vi "AlliGator Settings Window.vi"() -> ()   [LabVIEW 2021, in "AlliGator Settings.lvlib"]
doc: "GUI providing access to settings parameters for all aspect of AlliGator's functions."
uses:
  AlliGator Settings.lvlib
  Phasor Plot/AlliGator Phasor Plot Size.ctl
  AlliGator Background Subtraction Parameters.ctl
  Graphs/XY Graph/XY Graph Plot Shift Parameters.ctl
  Graphs/XY Graph/XY Graph Plot Shift Method.ctl
  Image/Image Save File Format.ctl
  AlliGator Low Count Pixels Rejection Options.ctl
  Phasor/Phasor Ratio Type.ctl
  Decay Analysis/Decay Preprocessing/AlliGator Baseline Subtraction Method.ctl
  Fits/IRF(X)PSED/Decay Fit Options v4.ctl
  Fits/Decay Convolution/Decay Model.ctl
  Fits/Residual Type.ctl
  Fits/IRF(X)PSED/Fit Weights Type v2.ctl
  Fits/Non-linear Fitting Method v2.ctl
  Fits/Fit Calculation Method.ctl
  Fits/Non-linear Fitting Algorithm.ctl
  Fits/IRF(X)PSED/Decay Fit Parameters & Derived Quantities List v2.ctl
  Decay Analysis/Decay Fit/AlliGator Decay Fit Parameter Constraints 2.ctl
  Fits/IRF(X)PSED/Decay Fit Parameters In List.ctl
  Decay Analysis/IRF/AlliGator IRF Optimization Controls.ctl
  Decay Analysis/IRF/AlliGator IRF Deconvolution Metrics.ctl
  Math/Advanced Signal Processing Toolkit/Wavelet Analysis Options.ctl
  AlliGator High Count Pixels Rejection Options.ctl
  AlliGator Image Smoothing Options.ctl
  Arrays/Kernel Type.ctl
  Arrays/Smoothing Algorithm.ctl
  Fits/Square Pulse/Square Pulse Options.ctl
  Fits/Square Pulse/Square Pulse Levels Type.ctl
  Source Image/AlliGator Image Binning Options.ctl
  Phasor Plot/AlliGator Phasor Plot Smoothing Options.ctl
  AlliGator Phasor Plot Graphics Options.ctl
  AlliGator Exported Image Settings.ctl
  Fits/IRF(X)PSED/IRF(X)PSED Extraction Options.ctl
  Fits/IRF(X)PSED/Fourier Series Smoothing Option.ctl
  Fits/IRF(X)PSED/Fourier Series Truncation.ctl
  Fits/IRF(X)PSED/IRF Extraction Method.ctl
  Phasor/Phasor Explorer Display Parameters.ctl
  Phasor/Phasor Type of Series.ctl
  Phasor/Phasor Explorer Decay Parameters.ctl
  Phasor/Phasor IRF Model.ctl
  Phasor/Phasor Explorer Phasor Parameters.ctl
  Phasor/Phasor Calculation Type.ctl
  Phasor/Phasor SEPL Type.ctl
  Phasor/Phasor Explorer Gate Parameters.ctl
  Phasor/Phasor Gate Type.ctl
  Phasor/Phasor Type of User-defined Function.ctl
  Phasor/Phasor Explorer Gate Parameter to Adjust.ctl
  AlliGator Define Gates to.ctl
  AlliGator Gates to Keep.ctl
  Phasor Ratio/AlliGator Phasor Ratio Color-Coded Quantity.ctl
  Phasor/Phasor Calibration Type.ctl
  Histograms/Linear Histogram Options.ctl
  Histograms/Histogram Bin Option.ctl
  Histograms/Histogram Bin Position.ctl
  AlliGator Gate Arithmetic.ctl
  Phasor Ratio/AlliGator Phasor Reference Associated with Shortest Lifetime.ctl
  AlliGator Python Settings.ctl
  SwissSPAD/SwissSPAD Live_Image Display Options.ctl
  AlliGator Average Lifetime Options.ctl
  Phasor Calibration/AlliGator Calibration Map Algorithm.ctl
  Decay Analysis/Decay Fit/AlliGator Guess Parameters Options.ctl
  Phasor/Phasor Standard Deviation Options.ctl
  Source Image/AlliGator Source Image Scale Bar Options.ctl
  Fits/IRF(X)PSED/MLE Baseline Offset Type.ctl
  Fits/Optimal Offset Selection Criterion.ctl
  AlliGator Settings Q Element.ctl
  AlliGator Settings Q Action.ctl
  Globals, Variables, Constants/AlliGator Refnums List.ctl
  AlliGator Settings List.ctl
  Globals, Variables, Constants/AlliGator Variables List.ctl
  Image/Image Hot Pixel Map Target.ctl
  Action Engine/AlliGator Q Element.ctl
  Action Engine/AlliGator Q Event.ctl
  Palette/Image Palette Information.ctl
  Image/Image Display Palette Type.ctl
  Notebook/Notebook Parameters List.ctl
  GUI/AlliGator Skippable Windows Status.ctl
  AlliGator Quantities.ctl
  f3e5a785-d283-42c9-a630-fb32b7f70655.vi
  c46dad3f-f40e-47bf-8043-7fc63249f95d.vi
  Variant/Variant to Data/Variant to [String].vi
  Variant/Variant to Data/Variant to I32.vi
  Variant/Variant to Data/Variant to Boolean.vi
  Formula/Aliases Definition Window.vi
  Variant/Variant to Data/Variant to U16.vi
  Variant/Variant to Data/Variant to String.vi
  Variant/Variant to Data/Variant to Path.vi
  Variant/Variant to Data/Variant to U32.vi
  Action Engine/AlliGator Action Engine.lvlib
  Globals, Variables, Constants/AlliGator Globals, Variables & Constants.lvlib
  Variant/Variant to Data/Variant to Data.lvlib
  Palette/Palette.lvlib
  Image/Image.lvlib
  GUI/AlliGator GUI.lvlib
  Phasor Plot/AlliGator Phasor Plot.lvlib
  Phasor Graph/AlliGator Phasor Graph.lvlib
  Error/Error.lvlib
  Graphs/Plot Editor/Plot Editor.lvlib
  Phasor/Phasor Explorer.lvlib
  Phasor Ratio/AlliGator Phasor Ratio.lvlib
  Utilities/Utilities.lvlib
  <vilib>/vision/NI_Vision_Development_Module.lvlib
  Python Plugins API/AlliGator Python Plugins.lvlib
  Notebook/Notebook.lvlib
  SwissSPAD/SwissSPAD Live.lvlib
  Formula/Formula.lvlib
  Fits/Fits.lvlib
  Phasor/Phasor.lvlib
  Graphs/XY Graph/XY Graph Add-Ons.lvlib
  Decay Analysis/Decay Fit/AlliGator Decay Fit.lvlib
  Decay Analysis/IRF/AlliGator IRF.lvlib
  Math/Math.lvlib
  Arrays/Arrays.lvlib
  Source Image/AlliGator Source Image.lvlib
  Histograms/Histogram Window.lvlib
  Phasor Calibration/AlliGator Phasor Calibration.lvlib
  Decay Analysis/Decay Preprocessing/AlliGator Decay Preprocessing.lvlib
panel:
  in  "Settings Tabs":T1(tab)
  in  "Source Image Tabs":T2(tab)
  in  "Hot Pixel Removal":T3 caption="Hot Pixel Removal (*)" {"Percentile" min=0 max=100}
  in  "Use Image Histogram for Contrast":bool=TRUE
  in  "Low Count Pixels Rejection Options":T4={"Background Low Threshold Factor"=0.0, "Fixed Low Background Threshold"=20000.0, "Reject Low Count Pixels"=FALSE, "Low Percentile"=0.0} {"Low Percentile" min=0.0 max=100.0}
  in  "High Count Pixels Rejection Options":T5={"Background High Threshold Factor"=0.0, "Fixed High Background Threshold"=1.0, "Reject High Count Pixels"=FALSE, "High Percentile"=100.0} {"High Percentile" min=0.0 max=100.0}
  in  "ROI Creation":string="ROI Creation"
  in  "Image Pre-Processing Operations Order":u16(ring) items=["Remove Screamers", "Pile-up Correction", "Binning", "Smoothing", "Rescaling"]
  in  "Dead Left Columns Correction":bool
  in  "ROI Diameter":i32=12
  in  "Use Fixed ROI Diameter":bool
  in  "ROI Center Color":u32(colorbox)=16711680
  in  "Peak Threshold":dbl=500.0
  in  "Image Smoothing Options":T6={"Use Image Smoothing"=FALSE, "Kernel Type"=enum."Bilinear", "Bin"=1, "Algorithm"=enum."Rapid"} caption="Image Smoothing Options (*)" {"Bin" min=1}
  in  "Image Binning Options":T9={"Use Image Binning"=FALSE, "X Bin"=1, "Y Bin"=1} caption="Image Binning Options (*)" {"Y Bin" min=1; "X Bin" min=1}
  in  "Invert Binary Mask":bool
  in  "Intensity Threshold":dbl=500.0
  in  "Overlay Analyzed ROI Center":bool
  in  "Save Source Image":bool caption="Save Image"
  in  "Median Overlay Color":u32(colorbox)
  in  "Overlay ROI Median":bool=TRUE caption="Use Image Brightness"
  in  "Use Image Brightness":bool=TRUE
  in  "Blend Overlay with Image Background":bool=TRUE
  in  "Scale Bar Options":T10 caption="Scale Bar Options (*)"
  in  "Image Resolution (Pixel Size)":dbl[unit]
  in  "Dataset Scaling Factor":dbl=1.0 caption="Scaling Factor" min=0.0
  in  "Gate Image Integration":dbl[unit]=3e-10 min=0.0 format="%#.3g"
  in  "Gate Image Exposure":dbl[unit]=3e-10 min=0.0 format="%#.3g"
  in  "Available Channel Names":string[](array[string])
  in  "Background File Subtraction":bool
  in  "Background Scaling Factor":dbl=1.0 caption="Scaling Factor" min=0.0
  in  "Background File":path caption="Background Dataset"
  in  "Background Pile-up Correction":bool caption="Pile-up Correction"
  in  "Background Pixel Well Capacity":u32=1 caption="Max Value" min=1 step=1
  in  "Pixel Well Capacity":u32=1 caption="Max Value" min=1 step=1
  in  "Pile-up Correction":bool
  in  "Channel Arithmetic":T11 caption="Channel Arithmetic (*)"
  in  "Channel Name":u16(ring) items=["Gate"]
  in  "Gates to Keep":T12={"First"=0, "Last"=4294967295} caption="Gates to Keep (*)"
  in  "Define Gates to":T13 caption="Define Gates to (*)"
  in  "SYNC Period":dbl[unit] min=0.0 format="%#.3g"
  out "Natural Frequency":dbl[unit] min=0.0 format="%#.3g"
  in  "# Gates":u32=1 min=1 step=1
  in  "Gate Step":u32=1 caption="Gate Step (*)" min=1 step=1
  in  "Gate Width":dbl[unit]=3e-10 min=0.0 format="%#.3g"
  in  "Nanotime Gate Separation":dbl[unit]=4e-11 caption="Gate Separation" min=0.0 format="%#.3g"
  in  "Gates to Skip":T14 caption="Gates to Skip (*)"
  in  "Laser Period":dbl[unit] min=0.0 format="%#.3g"
  in  "Fluorescence Decay Tabs":T15(tab) caption="Fluorescence Decay Tab"
  in  "[0-1]-Normalize Decay":bool caption="1- Normalize Decay"
  in  "# Folds":u32=1 min=1
  in  "Fold Decay":bool caption="Straighten Decay"
  in  "Use Decay Pre-Processing":bool=TRUE
  in  "Head Fraction":dbl min=0.0 max=1.0 format="%.4g"
  in  "Use Cursors":bool
  in  "Use Periodicity":bool
  in  "Pixel-Normalize Decay":bool
  in  "Constant Background":dbl=1.0
  in  "Verbose Decay Pre-Processing":bool=TRUE
  in  "Decay Pre-Processing Operations Order":u16(ring) items=["Background subtraction", "Reverse", "Smoothen", "Straighten", "Shift", "Extrapolate", "Normalize", "Fold"]
  in  "Straighten Decay":bool
  in  "Background Subtraction":bool=TRUE
  in  "Baseline Subtraction Method":T16=enum."Min"
  in  "Background Definition Range":T17={"Min Gate"=0.0, "Max Gate"=8e-10} {"Max Gate" min=0.0 format="%#_5g"; "Min Gate" min=0.0 format="%#_5g"}
  in  "Additional Points":u32
  in  "Tail Fraction":dbl min=0.0 max=1.0 format="%.4g"
  in  "Extrapolate Decay":bool
  in  "Shift Decay":bool
  in  "Smoothen Decay":bool
  in  "Smoothing Parameter":dbl=-1.0 min=0.0 max=1.0
  in  "1-Normalize Decay":bool caption="1- Normalize Decay"
  in  "Decay Shift Parameters":T18
  in  "Reverse Gates":bool
  in  "Average Lifetime Options":T20={"Use Local IRF "=TRUE, "Use IRF Offset"=TRUE, "Use Fixed Offset"=TRUE, "Fixed Offset"=0.0, "Baseline %"=0.0} caption="Use Local IRF" {"Baseline %" min=0.0 max=100.0}
  in  "IRF Extraction Options":T21={"Time Constant for IRF Extraction"=1e-18, "IRF Order"=1, "Fourier Series Smoothing"=enum."None", "Noise Threshold"=0.0, "Smoothing Width"=0.0, "Fourier Series Truncation"=enum."Automatic", "Truncation Order"=0, "Save Power Spectrum"=FALSE, "Smoothing"=FALSE, "Smoothing Parameter"=0.0, "Smoothing Order"=1, "Method"=enum."Direct"} {"Smoothing Order" max=100 step=1; "Smoothing Parameter" min=-1.0 max=1.0; "Time Constant for IRF Extraction" min=0.0 format="%#_5g"}
  in  "IRF Optimization Options":T25={"Search Range"=1e-18, "Search Step"=1e-09, "Tail Threshold (%)"=1e-09, "Regularized IRF"=FALSE, "Export Plot"=FALSE, "Export Data"=FALSE, "Smooth Metrics"=FALSE, "S-G Side Points"=1, "S-G Polynomial Order"=3, "Metrics"=enum."Tail Average"} {"S-G Polynomial Order" min=3 max=10; "S-G Side Points" min=1; "Tail Threshold (%)" min=0.0 max=100.0; "Search Step" min=0.0; "Search Range" min=0.0}
  in  "Square Pulse Options":T27={"Method"=enum."Mode", "# Bins"=0, "Threshold %"=10.0, "Center on Midpoint"=FALSE, "Smoothen Plot"=FALSE} {"Threshold %" min=0.0 max=100.0}
  in  "Wavelet Analysis Options":T29={"Wavelet"=enum."db02", "Option for Approximate Coefficients"=enum."None", "# Levels"=1, "Threshold Settings"={"Thresholding Rule"=enum."Universal", "Rescaling Method"=enum."Single level", "Soft Threshold?"=TRUE}, "Wavelet Transform Type"=enum."Discrete"}
  in  "Extract IRF instead of Decay":bool
  in  "Use Data Information Laser Period":bool
  in  "Use Legacy Fitting Approach":bool
  in  "Fit Options":T30={"Show Fit Residuals"=TRUE, "Fit Model"=enum."1-Exponential", "Residual Type"=enum."Standard", "Max Decay Percentile"=1.0, "Min Decay Percentile"=0.0, "Show Full Decay"=TRUE, "Weights"=enum."1/Variance (Neyman)", "Fitting Method"=enum."Least Square", "Compute Parameter Uncertainties"=TRUE, "Periodic Boundaries"=FALSE, "Model Calculation"=enum."Simulation", "Period"=1.2500000000000001e-08, "Termination Criteria"={"Max Iterations"=1000, "Max Function Calls"=0, "Max Time"=1000.0, "Function Tolerance"=1e-06, "Parameter Tolerance"=1e-06, "Gradient Tolerance"=0.0, "Min Lambda"=1e-06, "Max Lambda"=1e-06, "Initial Tick Count"=0}, "Offset Resolution"=4e-11, "Use Local IRF"=TRUE, "Fitting Algorithm"=enum."Levenberg-Marquardt", "Show Confidence Interval "=TRUE, "Confidence Level"=95.0} {"Confidence Level" min=0.0 max=100.0; "Offset Resolution" min=0.0; "Period" min=0.0; "Min Decay Percentile" min=0.0 max=100.0; "Max Decay Percentile" min=0.0 max=100.0}
  in  "MLE Baseline Offset Type":T37
  in  "MLE Baseline Offset":dbl
  in  "Optimal Offset Selection Criterion":T38
  in  "Guess Parameters Options":T39 caption="Options"
  in  "Use Last Fitted Parameters":bool
  in  "Guess Parameter Names":T40[](array[typedef]) caption="Names"
  in  "Use Guess Parameters":bool
  in  "Guess Parameter Values":dbl[](array[numeric]) caption="Values"
  in  "Fit Parameter Constraints":T41[](array[typedef]) {"Max Value" format="%#.3g"; "Min Value" format="%#.3g"}
  in  "Displayed Fit Parameters":T42[](array[typedef])
  in  "Export Tabulated Results":bool=TRUE
  in  "Fluorescence Decay Graph Default Plot Style":cluster{"X":dbl, "Y":dbl}[](graph) caption="Phasor Graph Default Plot Style"
  in  "Decay Graph Color Array":u32[](array[colorbox])
  in  "Show Last Decay Only":bool caption="Show Last Decay only"
  in  "Max Peak Value":dbl
  in  "Reject High Decay Peak Pixels":bool
  in  "Min Peak Value":dbl
  in  "Reject Low Decay Peak Pixels":bool
  in  "Intensity Correction File":path
  in  "Use Intensity Correction File":bool
  in  "Use File Timestamp":bool
  in  "Time Step":dbl[unit]=1.0
  in  "Phasor Plot Tabs":T43(tab)
  in  "Intensity-weighted Phasor Plot":bool
  in  "Phasor Plot Smoothing Options":T44={"Use Phasor Plot Smoothing"=FALSE, "Kernel Type"=enum."Uniform", "Bin"=1, "Algorithm"=enum."Rapid"} {"Bin" min=1 step=2}
  in  "Phasor Plot Frequency":dbl[unit]=80000000.0 caption="Phasor Frequency"
  in  "Selected Image ROI(s)":bool
  in  "All Image ROIs":bool
  in  "Selected Phasor Plot ROI(s)":bool
  in  "All Phasor Plot ROIs":bool
  in  "Cumulative Phasor Plot":bool
  in  "Store Phasor Harmonics":bool
  in  "Phasor Ratio Color Scale":dbl(ramp)
  in  "Phasor Ratio Decay Range":dbl=1.0 caption="Decay Range"
  in  "Phasor Ratio Reference Colors":T45={"Reference 1"=3381759, "Reference 2"=3381759, "Boundary"=3381759} caption="Reference Colors"
  in  "Exponential Fading":bool
  in  "Phasor Ratio Color Map Type":T46(radio) caption="Color Map Type"
  out "Phasor Ratio Color Map":string caption="Average Lifetime Color Map"
  out "Ref 2 Label":string="Ref 1"
  out "Ref 1 Label":string="Ref 2"
  in  "Phasor Ratio Display Range":cluster{dbl, dbl}(slide)={0.0, 454.0} caption="Average Lifetime Display Range" scale=0.0..0.1 scale format="%#.3g"
  in  "Reference Radius":i32=512 min=1
  in  "Phasor Ratio Color-Coded Quantity":T47 caption="Displayed Quantity"
  in  "Draw Reference Segment":bool
  in  "User-Defined Quantity":string
  in  "Blend Overlay with Phasor Background":bool=TRUE
  in  "Use Phasor Brightness":bool
  in  "Phasor Plot Size":T48={"H"=512, "V"=512, "Margin"=0.2} {"Margin" min=0.0}
  in  "Phasor Plot Graphics Options":T49={"UC Color"=3381759, "Show UC Tau Ticks"=FALSE, "SEPL Color"=3381759, "Show SEPL Tau Ticks"=FALSE, "Axes Color"=16776960, "Show (g,s) Ticks"=FALSE, "Show UC"=FALSE, "Show SEPL"=FALSE, "Show Axes"=FALSE, "Show UC Tau Labels"=FALSE, "Show SEPL Tau Labels"=FALSE, "Show (g,s) Labels"=FALSE, "UC Label Size"=18, "UC Label Distance"=0.0, "SEPL Label Size"=18, "SEPL Label Distance"=0.0, "Axes Label Size"=18, "Axes Label Distance"=0.0}
  in  "Intensity-weighted Phasor Graph":bool
  in  "Define Shortest Lifetime as":T50
  in  "Save Phasor Graph Image":bool
  in  "Phasor Graph Frequency":dbl[unit]=80000000.0 caption="Phasor Frequency"
  in  "Phasor Ratio Type":T51
  in  "Pixel-level Phasor Computation":bool
  in  "Phasor SDV Options":T52={"Compute Estimated SDV"=FALSE, "# Replicas"=100, "Use Estimated Average Phasor"=FALSE}
  in  "SEPL Tabs":enum32{"Display", "Phasor", "IRF", "Gates"}(tab)
  in  "Display Parameters":T53={"# Points"=1000, "Ramp Type"=enum."Logarithmic", "Type of Series"=enum."1-Exp Decays", "Min tau"=1.0000000000000002e-12, "Max tau"=1.0000000000000001e-07, "Include 0"=FALSE, "Include Infinity"=FALSE} {"Min tau" min=0.0; "Max tau" min=0.0; "# Points" min=1 step=1}
  in  "Phasor Parameters":T55={"Harmonic Frequency"=0.0, "Use f* = 1/D Frequency"=FALSE, "Calibrated Phasor"=FALSE, "Calibration Lifetime"=1e-09, "Phasor Calculation"=enum."Direct Sum", "SEPL Type"=enum."UC", "# Gates"=1.0, "Square Gate Width"=1e-09, "Show Ticks"=FALSE} {"Square Gate Width" min=0.0; "# Gates" min=0.0; "Calibration Lifetime" min=0.0; "Harmonic Frequency" min=0.0}
  in  "Decay & IRF Parameters":T58={"Lifetime"=3.0000000000000004e-09, "IRF Offset"=0.0, "IRF Period"=1.2500000000000001e-08, "Normalized Decays"=FALSE, "IRF Model"=enum."Dirac", "IRF Parameter 1"=0.0} caption="IRF Parameters" {"Lifetime" min=0.0; "IRF Period" min=0.0}
  in  "Edit User-defined Function":bool caption="Edit User-defined Gate"
  in  "Gate Parameter to Adjust":T60 caption="Adjust"
  in  "Match Laser Period":bool=TRUE
  in  "Gate Parameters":T61={"First Gate Start"=0.0, "Use Gate Center"=FALSE, "Gate Width"=0.0, "Gate Step"=0.0, "# Gates"=1.0, "Gate Type"=enum."Square", "Edge Width"=0.0, "Top Slope"=0.0, "Reversed Sawtooth?"=FALSE, "Analytical Computation"=FALSE, "Integration"=enum."Item 0", "Tolerance"=1.0, "# Steps"=1.0, "Type of User-defined Function"=enum."Gate", "Use Gate Step"=FALSE} {"# Steps" min=0.0; "Tolerance" min=0.0; "Top Slope" min=0.0; "Edge Width" min=0.0; "Gate Step" min=0.0; "# Gates" min=1.0 step=1.0; "Gate Width" min=0.0}
  in  "Use Current Dataset Parameters":bool
  in  "Calibration Map Algorithm":T64
  in  "Calibration Type":T65=enum."Single Phasor"
  in  "Backup Calibration Type":T66(ring) caption="Backup Calibration"
  in  "Use Backup Calibration if needed":bool=TRUE
  in  "Calibration Lifetime":dbl[unit]=1e-09
  in  "Lifetime Analysis Graph Default Plot Style":cluster{"X":dbl, "Y":dbl}[](graph) caption="Phasor Graph Default Plot Style"
  in  "Decay Analysis Parameters":T18
  in  "Plugins Folder":bool
  in  "Parameter Names only":bool
  in  "Send JSON to Clipboard":bool
  in  "Reset Python Session":bool
  out "Valid Python Session":bool
  in  "Python Settings":T67
  in  "Transparent Mask Color":u32(colorbox)
  in  "ROI Description Max Characters":i32=256
  in  "Beep on Error":bool caption="Verbose Error Mode"
  in  "# Logical Processors Used":i32 caption="Used" min=1 max=16
  out "# Logical Processors":i32
  in  "Histogram Options":T68={"Bin Size"=0.0, "Bin Number"=0, "Bin Option"=enum."Bin Number", "Min Value"=-inf, "Max Value"=inf, "Filter NaN & Infinite Values"=TRUE, "Frequency Plot"=FALSE, "Align Bins"=FALSE, "Bin Location"=enum."Left", "Project Outside Values"=FALSE, "Max Histogram Size"=100000} {"Max Histogram Size" format="%.0e"}
  in  "Exported Gate Image Settings":T71
  in  "Restore Skipped Dialogs":bool
  in  "Verbose Error Mode":bool
  in  "Verbose Settings Mode":bool
  in  "Beep after Script":bool
  in  "Include Loading in Timing":bool
  in  "Verbose Mode":bool
  in  "Saved Displayed Image File Format":T72
  # "Image ROI"
  # "Gates Characteristics"
  # "Dataset Pile-up Correction (*)"
  # "Background File Subtraction (*)"
  # "Guess Parameters"
  # "Limit Phasor Plot Calculation  to:"
  # "Limit Phasor Plot Analysis  to:"
  # "Phasor Ratio/Average Lifetime Style Options"
  # "Phasor Plot Size & Style"
  # "Calibration Options"
  # "Image Saving Options"
  # "UI Options"
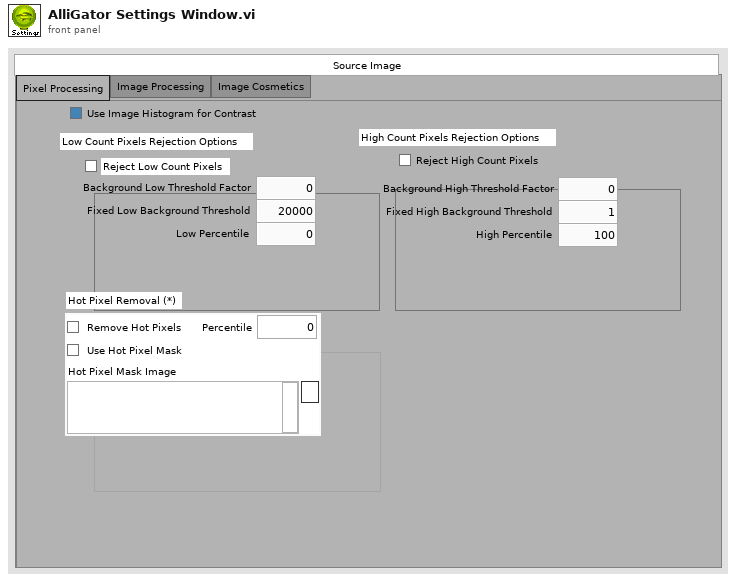
[diagram p1: front panel]
types:
  T1 = enum32{"Source Image", "Data Information", "Fluorescence Decay", "Fluorescence Decay Statistics", "Intensity Time Trace", "Phasor Plot", "Phasor Graph", "Single-Exponential Phasor Locus (SEPL)", "Phasor Calibration", "Lifetime Analysis", "Plugins", "Miscellaneous"}
  T2 = enum32{"Pixel Processing", "Image Processing", "Image Cosmetics"}
  T3 = typedef "SwissSPAD Live.lvlib/SwissSPAD Live_Image Display Options.ctl" = cluster{"Remove Screamers":bool, "Delta":sgl, "Equalize Histogram":bool, "Percentile":sgl, "Hot Pixel Mask Image":path, "Use Hot Pixel Mask":bool}
  T4 = typedef "AlliGator Settings.lvlib/AlliGator Low Count Pixels Rejection Options.ctl" = cluster{"Background Low Threshold Factor":dbl, "Fixed Low Background Threshold":dbl, "Reject Low Count Pixels":bool, "Low Percentile":dbl}
  T5 = typedef "AlliGator Settings.lvlib/AlliGator High Count Pixels Rejection Options.ctl" = cluster{"Background High Threshold Factor":dbl, "Fixed High Background Threshold":dbl, "Reject High Count Pixels":bool, "High Percentile":dbl}
  T6 = typedef "AlliGator Settings.lvlib/AlliGator Image Smoothing Options.ctl" = cluster{"Use Image Smoothing":bool, "Kernel Type":T7, "Bin":i32, "Algorithm":T8}
  T7 = typedef "Arrays.lvlib/Kernel Type.ctl" = enum16{"Uniform", "Bilinear", "Gaussian"}
  T8 = typedef "Arrays.lvlib/Smoothing Algorithm.ctl" = enum16{"Rapid", "Thorough"}
  T9 = typedef "AlliGator Source Image.lvlib/AlliGator Image Binning Options.ctl" = cluster{"Use Image Binning":bool, "X Bin":i32, "Y Bin":i32}
  T10 = typedef "AlliGator Source Image.lvlib/AlliGator Source Image Scale Bar Options.ctl" = cluster{"Show Scale Bar Overlay":bool, "Scale Bar Length":dbl[unit], "Scale Bar Color":u32, "Scale Bar X":u32, "Scale Bar Y":u32, "Scale Bar Height":dbl[unit]}
  T11 = typedef "AlliGator Settings.lvlib/AlliGator Gate Arithmetic.ctl" = enum16{"None", "INT-G2", "G2/INT*<INT>", "(1 - G2/INT)*<INT>"}
  T12 = typedef "AlliGator Settings.lvlib/AlliGator Gates to Keep.ctl" = cluster{"First":u32, "Last":u32}
  T13 = typedef "AlliGator Settings.lvlib/AlliGator Define Gates to.ctl" = enum32{"Skip", "Keep"}
  T14 = typedef "AlliGator Settings.lvlib/AlliGator Background Subtraction Parameters.ctl" = cluster{"Start":u32, "End":u32}
  T15 = enum32{"Decay Pre-Processing", "Advanced Analysis", "Fit Options", "Fit Parameters", "Styles"}
  T16 = typedef "AlliGator Decay Preprocessing.lvlib/AlliGator Baseline Subtraction Method.ctl" = enum16{"Mean", "Min", "Square Gated Single-Exponential", "File", "Constant"}
  T17 = cluster{"Min Gate":dbl[unit], "Max Gate":dbl[unit]}
  T18 = typedef "XY Graph Add-Ons.lvlib/XY Graph Plot Shift Parameters.ctl" = cluster{"Type":T19, "Shift":dbl[unit], "Threshold":dbl, "Rotate":bool}
  T19 = typedef "XY Graph Add-Ons.lvlib/XY Graph Plot Shift Method.ctl" = enum16{"Default", "CFD", "Threshold", "Cross-Correlation"}
  T20 = typedef "AlliGator Settings.lvlib/AlliGator Average Lifetime Options.ctl" = cluster{"Use Local IRF ":bool, "Use IRF Offset":bool, "Use Fixed Offset":bool, "Fixed Offset":dbl[unit], "Baseline %":dbl}
  T21 = typedef "Fits.lvlib/IRF(X)PSED Extraction Options.ctl" = cluster{"Time Constant for IRF Extraction":dbl[unit], "IRF Order":i32, "Fourier Series Smoothing":T22, "Noise Threshold":dbl, "Smoothing Width":dbl, "Fourier Series Truncation":T23, "Truncation Order":i32, "Save Power Spectrum":bool, "Smoothing":bool, "Smoothing Parameter":dbl, "Smoothing Order":u32, "Method":T24}
  T22 = typedef "Fits.lvlib/Fourier Series Smoothing Option.ctl" = enum16{"None", "Lanczos Factors", "Fejer Summation"}
  T23 = typedef "Fits.lvlib/Fourier Series Truncation.ctl" = enum16{"Automatic", "Fixed"}
  T24 = typedef "Fits.lvlib/IRF Extraction Method.ctl" = enum16{"Direct", "Topless", "Toeplitz"}
  T25 = typedef "AlliGator IRF.lvlib/AlliGator IRF Optimization Controls.ctl" = cluster{"Search Range":dbl[unit], "Search Step":dbl[unit], "Tail Threshold (%)":dbl, "Regularized IRF":bool, "Export Plot":bool, "Export Data":bool, "Smooth Metrics":bool, "S-G Side Points":i32, "S-G Polynomial Order":i32, "Metrics":T26}
  T26 = typedef "AlliGator IRF.lvlib/AlliGator IRF Deconvolution Metrics.ctl" = enum16{"Tail Average", "Tail SDV", "Tail Max", "Tail Average * SDV", "Tail Slope", "Residuals ACF SDV", "Delta tau", "Reduced Chi2", "Residuals Area"}
  T27 = typedef "Fits.lvlib/Square Pulse Options.ctl" = cluster{"Method":T28, "# Bins":i32, "Threshold %":dbl, "Center on Midpoint":bool, "Smoothen Plot":bool}
  T28 = typedef "Fits.lvlib/Square Pulse Levels Type.ctl" = enum16{"Mode", "Mean"}
  T29 = typedef "Math.lvlib/Wavelet Analysis Options.ctl" = cluster{"Wavelet":enum16{"db02", "db03", "db04", "db05", "db06", "db07", "db08", "db09", "db10", "db11", "db12", "db13", "db14", "Haar", "bior1_3", "bior1_5", "bior2_2", "bior2_4", "bior2_6", "bior2_8", "bior3_1", "bior3_3", "bior3_5", "bior3_7", "bior3_9", "bior4_4 (FBI)", "bior5_5", "bior6_8", "coif1", "coif2", "coif3", "coif4", "coif5", "sym2", "sym3", "sym4", "sym5", "sym6", "sym7", "sym8"}, "Option for Approximate Coefficients":enum16{"None", "Threshold", "Detrend"}, "# Levels":i32, "Threshold Settings":cluster{"Thresholding Rule":enum16{"SURE", "Hybrid", "Universal", "Minimax"}, "Rescaling Method":enum16{"One", "Single level", "Multiple levels"}, "Soft Threshold?":bool}, "Wavelet Transform Type":enum16{"Discrete", "Undecimated"}}
  T30 = typedef "Fits.lvlib/Decay Fit Options v4.ctl" = cluster{"Show Fit Residuals":bool, "Fit Model":T31, "Residual Type":T32, "Max Decay Percentile":dbl, "Min Decay Percentile":dbl, "Show Full Decay":bool, "Weights":T33, "Fitting Method":T34, "Compute Parameter Uncertainties":bool, "Periodic Boundaries":bool, "Model Calculation":T35, "Period":dbl[unit], "Termination Criteria":cluster{"Max Iterations":i32, "Max Function Calls":i32, "Max Time":dbl[unit], "Function Tolerance":dbl, "Parameter Tolerance":dbl, "Gradient Tolerance":dbl, "Min Lambda":dbl, "Max Lambda":dbl, "Initial Tick Count":u32}, "Offset Resolution":dbl[unit], "Use Local IRF":bool, "Fitting Algorithm":T36, "Show Confidence Interval ":bool, "Confidence Level":dbl}
  T31 = typedef "Fits.lvlib/Decay Model.ctl" = enum16{"1-Exponential", "2-Exponentials"}
  T32 = typedef "Fits.lvlib/Residual Type.ctl" = enum16{"Standard", "Normalized", "Reduced"}
  T33 = typedef "Fits.lvlib/Fit Weights Type v2.ctl" = enum16{"Unweighted", "1/Variance (Neyman)", "1/Variance (Pearson)", "Best of All"}
  T34 = typedef "Fits.lvlib/Non-linear Fitting Method v2.ctl" = enum16{"Least Square", "Least Absolute Residual", "Bisquare", "MLE", "-", "Best of All"}
  T35 = typedef "Fits.lvlib/Fit Calculation Method.ctl" = enum16{"Simulation", "Convolution", "Integration"}
  T36 = typedef "Fits.lvlib/Non-linear Fitting Algorithm.ctl" = enum16{"Levenberg-Marquardt", "Trust-Region Dogleg"}
  T37 = typedef "Fits.lvlib/MLE Baseline Offset Type.ctl" = enum32{"Absolute", "Percentage"}
  T38 = typedef "Fits.lvlib/Optimal Offset Selection Criterion.ctl" = enum16{"Min Chi^2", "Max R^2"}
  T39 = typedef "AlliGator Decay Fit.lvlib/AlliGator Guess Parameters Options.ctl" = enum16{"Numerically estimated", "User-provided", "User-provided (normalized)", "Last valid fitted parameters"}
  T40 = typedef "Fits.lvlib/Decay Fit Parameters In List.ctl" = enum16{"Offset", "Baseline", "A_1", "tau_1", "A_2", "tau_2"}
  T41 = typedef "AlliGator Decay Fit.lvlib/AlliGator Decay Fit Parameter Constraints 2.ctl" = cluster{"Fit Parameter":T40, "Min Value":dbl, "Max Value":dbl, "Global":bool, "Used":bool}
  T42 = typedef "Fits.lvlib/Decay Fit Parameters & Derived Quantities List v2.ctl" = enum16{"Offset", "Baseline", "A_1", "tau_1", "A_2", "tau_2", "<tau>_a", "f1_a", "f2_a", "<tau>_i", "f1_i", "f2_i", "-", "R^2", "Chi^2"}
  T43 = enum32{"Phasor Plot Calculation", "Phasor Plot Information Overlay", "Phasor Plot Appearance"}
  T44 = typedef "AlliGator Phasor Plot.lvlib/AlliGator Phasor Plot Smoothing Options.ctl" = cluster{"Use Phasor Plot Smoothing":bool, "Kernel Type":T7, "Bin":i32, "Algorithm":T8}
  T45 = cluster{"Reference 1":u32, "Reference 2":u32, "Boundary":u32}
  T46 = enum32{"Interpolate Reference Colors", "Use Custom Map"}
  T47 = typedef "AlliGator Phasor Ratio.lvlib/AlliGator Phasor Ratio Color-Coded Quantity.ctl" = enum16{"Phasor Ratio (f1 or a1)", "Average Lifetime (<tau>_i or <tau>_a))", "User-Defined Quantity"}
  T48 = typedef "AlliGator Phasor Plot.lvlib/AlliGator Phasor Plot Size.ctl" = cluster{"H":i32, "V":i32, "Margin":dbl}
  T49 = typedef "AlliGator Settings.lvlib/AlliGator Phasor Plot Graphics Options.ctl" = cluster{"UC Color":u32, "Show UC Tau Ticks":bool, "SEPL Color":u32, "Show SEPL Tau Ticks":bool, "Axes Color":u32, "Show (g,s) Ticks":bool, "Show UC":bool, "Show SEPL":bool, "Show Axes":bool, "Show UC Tau Labels":bool, "Show SEPL Tau Labels":bool, "Show (g,s) Labels":bool, "UC Label Size":i16, "UC Label Distance":dbl, "SEPL Label Size":i16, "SEPL Label Distance":dbl, "Axes Label Size":i16, "Axes Label Distance":dbl}
  T50 = typedef "AlliGator Phasor Ratio.lvlib/AlliGator Phasor Reference Associated with Shortest Lifetime.ctl" = enum32{"Reference 1", "Reference 2"}
  T51 = typedef "Phasor.lvlib/Phasor Ratio Type.ctl" = enum32{"Intensity-weighted", "Amplitude-weighted"}
  T52 = typedef "Phasor.lvlib/Phasor Standard Deviation Options.ctl" = cluster{"Compute Estimated SDV":bool, "# Replicas":u32, "Use Estimated Average Phasor":bool}
  T53 = typedef "Phasor Explorer.lvlib/Phasor Explorer Display Parameters.ctl" = cluster{"# Points":i32, "Ramp Type":enum16{"Linear", "Logarithmic"}, "Type of Series":T54, "Min tau":dbl[unit], "Max tau":dbl[unit], "Include 0":bool, "Include Infinity":bool}
  T54 = typedef "Phasor.lvlib/Phasor Type of Series.ctl" = enum16{"1-Exp Decays", "Linear Combination of 1-Exp"}
  T55 = typedef "Phasor Explorer.lvlib/Phasor Explorer Phasor Parameters.ctl" = cluster{"Harmonic Frequency":dbl[unit], "Use f* = 1/D Frequency":bool, "Calibrated Phasor":bool, "Calibration Lifetime":dbl[unit], "Phasor Calculation":T56, "SEPL Type":T57, "# Gates":dbl, "Square Gate Width":dbl[unit], "Show Ticks":bool}
  T56 = typedef "Phasor.lvlib/Phasor Calculation Type.ctl" = enum16{"Direct Sum", "Analytical Formula"}
  T57 = typedef "Phasor.lvlib/Phasor SEPL Type.ctl" = enum16{"UC", "L_N", "L_N[W]", "L_X"}
  T58 = typedef "Phasor Explorer.lvlib/Phasor Explorer Decay Parameters.ctl" = cluster{"Lifetime":dbl[unit], "IRF Offset":dbl[unit], "IRF Period":dbl[unit], "Normalized Decays":bool, "IRF Model":T59, "IRF Parameter 1":dbl[unit]}
  T59 = typedef "Phasor.lvlib/Phasor IRF Model.ctl" = enum16{"Dirac", "Exponential"}
  T60 = typedef "Phasor Explorer.lvlib/Phasor Explorer Gate Parameter to Adjust.ctl" = enum16{"Gate Step", "# Gates"}
  T61 = typedef "Phasor Explorer.lvlib/Phasor Explorer Gate Parameters.ctl" = cluster{"First Gate Start":dbl[unit], "Use Gate Center":bool, "Gate Width":dbl[unit], "Gate Step":dbl[unit], "# Gates":dbl, "Gate Type":T62, "Edge Width":dbl[unit], "Top Slope":dbl[unit], "Reversed Sawtooth?":bool, "Analytical Computation":bool, "Integration":enum32{"Item 0", "Item 1"}, "Tolerance":dbl, "# Steps":dbl, "Type of User-defined Function":T63, "Use Gate Step":bool}
  T62 = typedef "Phasor.lvlib/Phasor Gate Type.ctl" = enum16{"Square", "Finite Edge Square", "Finite Edge, Tilted Top Square", "Triangle", "Sawtooth", "User-defined"}
  T63 = typedef "Phasor.lvlib/Phasor Type of User-defined Function.ctl" = enum16{"Gate", "IRF"}
  T64 = typedef "AlliGator Phasor Calibration.lvlib/AlliGator Calibration Map Algorithm.ctl" = enum16{"Simple Search", "Min Distance"}
  T65 = typedef "Phasor.lvlib/Phasor Calibration Type.ctl" = enum16{"None", "Single Phasor", "Phasor Series", "Phasor Map"}
  T66 = enum16{"Single Calibration", "Nearest Valid Calibration"}
  T67 = typedef "AlliGator Settings.lvlib/AlliGator Python Settings.ctl" = cluster{"Python Version":string, "Use PATH definition":bool, "Python.exe Path":path, "Include Example Plugins":bool}
  T68 = typedef "Histogram Window.lvlib/Linear Histogram Options.ctl" = cluster{"Bin Size":dbl, "Bin Number":i32, "Bin Option":T69, "Min Value":dbl, "Max Value":dbl, "Filter NaN & Infinite Values":bool, "Frequency Plot":bool, "Align Bins":bool, "Bin Location":T70, "Project Outside Values":bool, "Max Histogram Size":i32}
  T69 = typedef "Histogram Window.lvlib/Histogram Bin Option.ctl" = enum32{"Bin Number", "Bin Size"}
  T70 = typedef "Histogram Window.lvlib/Histogram Bin Position.ctl" = enum16{"Left", "Center", "Right"}
  T71 = typedef "AlliGator Settings.lvlib/AlliGator Exported Image Settings.ctl" = cluster{"bitness":bool, " Min Value":sgl, " Max Value":sgl}
  T72 = typedef "Image.lvlib/Image Save File Format.ctl" = enum16{"PNG", "JPEG", "BMP"}
  T73 = typedef "AlliGator Settings.lvlib/AlliGator Settings List.ctl" = enum16{"GUI:Visible Settings Tab", "GUI:Last Run Version", "Source Image:Use Image Histogram for Contrast", "Source Image:Low Count Pixels Rejection Options", "Source Image:High Count Pixels Rejection Options", "Source Image:Use Image Brightness", "Source Image:Blend Overlay with Image Background", "Source Image:Use Fixed ROI Diameter", "Source Image:ROI Diameter", "Source Image:ROI Center Color", "Source Image:Peak Threshold", "Source Image:Intensity Threshold", "Source Image:Image Binning Options", "Source Image:Image Smoothing Options", "Source Image:Image Histogram Active", "Source Image:Invert Binary Mask", "Source Image:Hot Pixel Removal", "Source Image:Overlay Analyzed ROI Center", "Source Image:Auto-Adjust Contrast", "Source Image:Histogram Lower Percentile", "Source Image:Histogram Upper Percentile", "Source Image:Save Source Image", "Source Image:Scale Bar Options", "Source Image:Image Resolution (Pixel Size)", "Source Image:Flatfield Correction", "Source Image:Show Dead Left Columns Correction", "Source Image:Dead Left Columns Correction", "Source Image:Image Pre-Processing Operations Order", "Source Image:Overlay ROI Median", "Source Image:Median Overlay Color", "Data Information:Gate Width", "Data Information:Nanotime Gate Separation", "Data Information:Macrotime Gate Separation", "Data Information:Gate Step", "Data Information:# Gates", "Data Information:Gate Image Exposure", "Data Information:Gate Image Integration", "Data Information:Gates to Skip", "Data Information:Gates to Keep", "Data Information:Define Gates to", "Data Information:Channel Name", "Data Information:Available Channel Names", "Data Information:Channel Arithmetic", "Data Information:Background File Subtraction", "Data Information:Background File", "Data Information:Background Scaling Factor", "Data Information:Background Pile-up Correction", "Data Information:Background Pixel Well Capacity", "Data Information:Laser Period", "Data Information:SYNC Period", "Data Information:Pile-up Correction", "Data Information:Pixel Well Capacity", "Data Information:Dataset Scaling Factor", "Fluorescence Decay_Decay Pre-Processing:Reverse Gates", "Fluorescence Decay_Decay Pre-Processing:Verbose Decay Pre-Processing", "Fluorescence Decay_Decay Pre-Processing:Use Decay Pre-Processing", "Fluorescence Decay_Decay Pre-Processing:Background Subtraction", "Fluorescence Decay_Decay Pre-Processing:Background Definition Range", "Fluorescence Decay_Decay Pre-Processing:Baseline Subtraction Method", "Fluorescence Decay_Decay Pre-Processing:Decay Pre-Processing Operations Order", "Fluorescence Decay_Decay Pre-Processing:Smoothing Parameter", "Fluorescence Decay_Decay Pre-Processing:Shift Decay", "Fluorescence Decay_Decay Pre-Processing:Decay Shift Parameters", "Fluorescence Decay_Decay Pre-Processing:Fold Decay", "Fluorescence Decay_Decay Pre-Processing:# Folds", "Fluorescence Decay_Decay Pre-Processing:1-Normalize Decay", "Fluorescence Decay_Decay Pre-Processing:[0-1]-Normalize Decay", "Fluorescence Decay_Decay Pre-Processing:Smoothen Decay", "Fluorescence Decay_Decay Pre-Processing:Extrapolate Decay", "Fluorescence Decay_Decay Pre-Processing:Use Periodicity", "Fluorescence Decay_Decay Pre-Processing:Use Cursors", "Fluorescence Decay_Decay Pre-Processing:Tail Fraction", "Fluorescence Decay_Decay Pre-Processing:Head Fraction", "Fluorescence Decay_Decay Pre-Processing:Additional Points", "Fluorescence Decay_Decay Pre-Processing:Straighten Decay", "Fluorescence Decay_Decay Pre-Processing:Constant Background", "Fluorescence Decay_Decay Pre-Processing:Pixel-Normalize Decay", "Fluorescence Decay_Advanced Analysis:Extract IRF instead of Decay", "Fluorescence Decay_Advanced Analysis:IRF Extraction Options", "Fluorescence Decay_Advanced Analysis:IRF Optimization Options", "Fluorescence Decay_Advanced Analysis:Square Pulse Options", "Fluorescence Decay_Advanced Analysis:IRF Order", "Fluorescence Decay_Advanced Analysis:IRF Time Constants", "Fluorescence Decay_Advanced Analysis:Wavelet Analysis Options", "Fluorescence Decay_Advanced Analysis:Average Lifetime Options", "Fluorescence Decay_Fit Options:Fit Options", "Fluorescence Decay_Fit Options:Use Legacy Fitting Approach", "Fluorescence Decay_Fit Options:Use Data Information Laser Period", "Fluorescence Decay_Fit Parameters:Displayed Fit Parameters", "Fluorescence Decay_Fit Parameters:Fit Parameter Constraints", "Fluorescence Decay_Fit Parameters:Export Tabulated Results", "Fluorescence Decay_Fit Parameters:MLE Baseline Offset Type", "Fluorescence Decay_Fit Parameters:MLE Baseline Offset", "Fluorescence Decay_Fit Parameters:Guess Parameter Names", "Fluorescence Decay_Fit Parameters:Guess Parameter Values", "Fluorescence Decay_Fit Parameters:Guess Parameters Options", "Fluorescence Decay_Fit Parameters:Optimal Offset Selection Criterion", "Fluorescence Decay_Styles:Show Last Decay Only", "Fluorescence Decay_Styles:Decay Graph Color Array", "Fluorescence Decay:Decay Graph Active", "Fluorescence Decay Statistics:Min Peak Value", "Fluorescence Decay Statistics:Reject Low Decay Peak Pixels", "Fluorescence Decay Statistics:Reject High Decay Peak Pixels", "Fluorescence Decay Statistics:Max Peak Value", "Time Traces:Use File Timestamp", "Time Traces:Time Step", "Time Traces:Use Intensity Correction File", "Time Traces:Intensity Correction File", "Phasor Plot:Phasor Plot Smoothing Options", "Phasor Plot:Phasor Plot Size", "Phasor Plot:Phasor Plot Graphics Options", "Phasor Plot:Cumulative Phasor Plot", "Phasor Plot:Use Phasor Brightness", "Phasor Plot:Blend Overlay with Phasor Background", "Phasor Plot:Save Phasor Plot", "Phasor Plot:Show References", "Phasor Plot:Phasor Ratio Decay Range", "Phasor Plot:Exponential Fading", "Phasor Plot:Phasor Ratio Reference Colors", "Phasor Plot:Reference Radius", "Phasor Plot:Show Color Map Vertices", "Phasor Plot:Phasor Plot Active", "Phasor Plot:Phasor Ratio Color Map Type", "Phasor Plot:Phasor Ratio Color Map", "Phasor Plot:Phasor Ratio Display Range", "Phasor Plot:Selected Image ROI(s)", "Phasor Plot:All Image ROIs", "Phasor Plot:Selected Phasor Plot ROI(s)", "Phasor Plot:All Phasor Plot ROIs", "Phasor Plot:Phasor Ratio Color-Coded Quantity", "Phasor Plot:Store Phasor Harmonics", "Phasor Plot:Draw Reference Segment", "Phasor Plot:User-Defined Quantity", "Phasor Plot:Color Scale High Color", "Phasor Plot:Color Scale Low Color", "Phasor Plot:Intensity-weighted Phasor Plot", "Phasor Graph:Phasor Frequency", "Phasor Graph:Phasor Ratio Type", "Phasor Graph:Pixel-level Phasor Computation", "Phasor Graph:Save Phasor Graph", "Phasor Graph:Phasor Graph Active", "Phasor Graph:Phasor SDV Options", "Phasor Graph:Intensity-weighted Phasor Graph", "Phasor Graph:Define Shortest Lifetime as", "Phasor Calibration:Use Backup Calibration if needed", "Phasor Calibration:Backup Calibration Type", "Phasor Calibration:Calibration Type", "Phasor Calibration:Calibration Lifetime", "Phasor Calibration:Calibration Map Algorithm", "Single-Exponential Phasor Locus (SEPL):Gate Parameters", "Single-Exponential Phasor Locus (SEPL):User-defined Gate", "Single-Exponential Phasor Locus (SEPL):User-defined IRF", "Single-Exponential Phasor Locus (SEPL):Phasor Parameters", "Single-Exponential Phasor Locus (SEPL):Decay & IRF Parameters", "Single-Exponential Phasor Locus (SEPL):Display Parameters", "Lifetime Analysis:Decay Analysis Parameters", "Lifetime Analysis:Lifetime Map Active", "Plugins:Python Settings", "Miscellaneous:Verbose Mode", "Miscellaneous:Beep after Script", "Miscellaneous:Saved Image File Format", "Miscellaneous:Exported Gate Image Settings", "Miscellaneous:Include Loading in Timing", "Miscellaneous:Verbose Settings Mode", "Miscellaneous:Histogram Options", "Miscellaneous:Beep on Error", "Miscellaneous:# Logical Processors Used", "Miscellaneous:ROI Description Max Characters", "Miscellaneous:Verbose Error Mode", "Miscellaneous:Transparent Mask Color"}
  T74 = typedef "AlliGator Globals, Variables & Constants.lvlib/AlliGator Refnums List.ctl" = enum16{"---------- AlliGator Controls ----------", "AlliGator Tab Control Refnum", "---------- AlliGator Indicators ----------", "Source Image Display Refnum", "Phasor Plot Display Refnum", "Decay Fit Parameter Map Refnum", "---------- AlliGator VIs ----------", "AlliGator Refnum", "AlliGator Settings Refnum", "AlliGator Launcher Refnum"}
  T75 = enum32{"Invalid", "Standard", "Closed", "Hidden", "Minimized", "Maximized"}
  T76 = typedef "AlliGator Settings.lvlib/AlliGator Settings Q Action.ctl" = enum16{"Idle", "Initialization", "End Initialization", "Refresh All Parameters", "Show Window", "Cumulative Phasor Plot Checkbox", "Shift Decay Checkbox", "Use Cursor (Extrapolate) Checkbox", "Use Periodicity (Extrapolate) Checkbox", "Baseline Subtraction Method", "Extrapolate Decay Checkbox", "Use Fixed ROI Diameter Checkbox", "Use File Timestamp Checkbox", "Use Calibration Phasor Curve Checkbox (deprecated)", "Use Single Phasor Calibration Checkbox (deprecated)", "Use Calibration Phasor Map Checkbox (deprecated)", "Smooth Decay Checkbox", "Phasor Ratio Color Map Type Radio Button", "Set Phasor Ratio Color Map", "Update SEPL Parameters", "Update SEPL Plot", "Define IRF Time Constants", "Set SEPL Parameters to Dataset Ones", "Define Gates to Use", "Fit Options Changed", "Phasor Ratio Color-Coded Quantity Changed", "Update Natural Frequency", "Channel Name Changed", "Send Parameters JSON Strings to Clipboard", "Load Hot Pixel Mask Image", "Get Phasor Ratio Color Scale Hi/Lo Colors", "Store Phasor Ratio Color Scale Hi/Lo Colors", "Quit"}
  T77 = typedef "AlliGator Settings.lvlib/AlliGator Settings Q Element.ctl" = cluster{"Action":T76, "Data":variant}
  T78 = typedef "AlliGator Globals, Variables & Constants.lvlib/AlliGator Variables List.ctl" = enum16{"---- GUI ----", "GUI:Initialization Status", "GUI:State Indicators Refnum", "GUI:Original AlliGator Menu Items", "GUI:Current Action Loop State", "GUI:Script in progress", "GUI:Playback", "GUI:Loop Playback", "GUI:Search ROI Used", "GUI:Search ROI", "Decay Graph Max Legend Size", "Intensity Graph Max Legend Size", "Decay Statistics Graph Max Legend Size", "Phasor Graph Max Legend Size", "Phasor Ratio Graph Max Legend Size", "Lifetime Graph Max Legend Size", "---- Files ----", "Files:Export Dataset Frames as Individual Files", "Files:Show Batch Export Help Balloons", "Files:Frames in Dataset", "Files:ptu File Frame Start Indices", "Files:Current Frame in Dataset", "Files:Current Frame Timestamp", "Files:Dataset Loaded", "Files:Dataset Metadata", "Files:Dataset Channel", "Files:Dataset Data Description", "Files:Background Dataset Metadata", "Files:Background Dataset Channel", "Files:Background Dataset Data Description", "Files:Background File Subtraction", "Files:Background File Path", "Files:Background File Pile-up Correction", "Files:Background File Pixel Well Capacity", "Files:Background File Scaling Factor", "Files:Current Dataset Load Settings", "Files:Dataset Path", "Files:ICCD-specific Information", "Files:Macrotime Gate Separation", "------ Python Plugins ------", "Python Plugins:Information", "Python Plugins:Python Session", "Python Plugins:Valid Python Session?", "---- Source Image ----", "Source Image:ROIs", "Source Image:Current ROI", "Source Image:ROI Event Refnum", "X_Source Image:Display Range", "X_Source Image:Palette Information", "X_Source Image:Type of Displayed Image", "X_Time Gate Slider", "Source Image:Palette List", "Source Image:Scale", "Source Image:ROI Overlay Color", "Source Image:Overlay to Erase", "Source Image:Is Displayed Image Accumulated", "Source Image:White Light Image Modified", "Source Image:Mask Image Modified", "---- Image Profile Window ----", "Image Profile:Window Event Refnum", "Image Profile:IntensityType", "Image Profile:Intensity Average Type", "Image Profile:Intensity-weighted SDV", "Image Profile:Box Profile Type", "Image Profile:Window Open", "Image Profile:Plotted Fit Parameter", "------ Phasor Graph -------", "Phasor Graph:Show Line", "---- Phasor Plot ---", "Phasor Plot:Parameters Changed", "Phasor Plot:FLI Dataset Modified since last Calculation", "Phasor Harmonics Data", "Selected Phasor Harmonics", "Phasor Harmonic Manager Event Refnum", "Phasor Plot:ROIs", "Phasor Plot:Current ROI", "Phasor Plot:ROI Event Refnum", "Phasor Plot:Image Reference Points", "Phasor Plot:Computed", "Phasor Plot:Palette Information", "Phasor Plot:Palette List", "Phasor Plot:Phasor Ratio Palette Information", "Phasor Plot:Phasor Ratio Palette List", "Phasor Plot:Image Scale", "Phasor Plot:Image Overlay to Erase", "Phasor Plot:Image Elements to Update", "Phasor Plot:Current Calculation Parameters", "Phasor Plot:Current Calibration Options", "Phasor Plot:Reset Cumulated Phasor Plot", "Phasor Plot:Reference 1", "Phasor Plot:Lifetime Reference 1", "Phasor Plot:Reference 1 Frequency", "Phasor Plot:Reference 2", "Phasor Plot:Lifetime Reference 2", "Phasor Plot:Reference 2 Frequency", "---- Decay Analysis ----", "Number of Selected Decays to Fit", "LS Fit Results", "LAR Fit Results", "BS Fit Results", "Last Decay Max - Min", "Best Fit Parameters", "Best Fit Parameter Names", "Actual Size X", "Actual Size Y", "Binning X", "Binning Y", "Actual # Gates", "Dataset Number", "Gates to...", "Gates Skipped", "Gates to keep", "Gate Step", "Gate Separation", "Reversed Gates", "Pile-up Correction", "Pixel Well Capacity", "Background Subtracted", "Background Subtraction Method", "Background Definition Range", "Background File (deprecated)", "Number of Dataset Accumulated", "Array of Accumulated Dataset Paths", "Do Averaged Datasets", "Destination File Path", "Process Plot Target", "Use 1/D as Phasor Frequency", "---- Decay Fit Parameter Map -----", "Decay Fit Parameter Map:Palette Information", "Decay Fit Parameter Map:Palette List", "Decay Fit Parameter Map:X Resolution", "Decay Fit Parameter Map:Y Resolution", "Decay Fit Parameter Map:Use Decay Fit Result Constraints", "Decay Fit Parameter Map:Decay Fit Result Constraints", "Decay Fit Parameter Map:Decay Fit Result Constraints Applied", "---- Parameter Map ----", "Parameter Map:Palette Information", "Parameter Map:Palette List", "------- Local Decay Window ---------", "Local Decay Graph Window:Event Refnum", "Local Decay Graph Window:Use normalized IRF for convolution", "----- Miscellaneous ----", "Misc:Skippable Dialog Windows Status"}
  T79 = typedef "Image.lvlib/Image Hot Pixel Map Target.ctl" = enum16{"U8", "U16", "SGL"}
  T80 = typedef "AlliGator Action Engine.lvlib/AlliGator Q Element.ctl" = cluster{"AlliGator Q Event":T81, "Data":variant}
  T81 = typedef "AlliGator Action Engine.lvlib/AlliGator Q Event.ctl" = enum16{"---- Files ----", "Files:Set Batch Export Files To Save", "Files:Set Dataset Loading & Pre-processing Options", "Files:Check #Frames in Dataset", "Files:Increment Frame Index", "Files:Open Mask Image", "Files:Open White Light Image", "Files:Open Single Dataset", "Files:New Folder of Folders Selected", "Files:Load File (all Types)_Scriptable", "Files:Move Flattened Series to Folders Series", "Files:Select Folder", "Files:Load FLI Dataset", "Files:Load Swiss SPAD 1 Dataset", "Files:Load Swiss SPAD 2 Dataset", "Files:Load .sdt FLI Dataset", "Files:Load .ptu FLI Dataset", "Files:Load .bin FLI Dataset", "Files:Load Single Gate Image Folder", "Files:Load I/m/phi Dataset (deprecated)", "Files:Load Single Image", "Files:Subtract Background File", "Files:Export FLI Dataset", "Files:Load HDF5 FLI Dataset", "Files:Set Destination File Path", "Files:Save Mask Image", "Files:Batch Conversion", "Files:New Folder Selected", "Files:Close FLI Dataset", "Files:Close FLI Dataset Series", "Files:Close White Light Image", "Files:Close Mask Image", "---- FLI Dataset ----", "FLI Dataset:Channel Arithmetic", "FLI Dataset:Export Average Lifetime Map as ASCII", "FLI Dataset:Export User-Defined Quantity Map as ASCII", "FLI Dataset:Python Function FLI Dataset Event", "FLI Dataset:ROI Analysis", "FLI Dataset:Tilted Logistic Square Gated IRF Characteristics Map", "FLI Dataset:Logistic Square Gated IRF Characteristics Map", "FLI Dataset:Square Gated IRF Characteristics Map", "FLI Dataset:Multi-ROI Single-Pixel Phasor Analysis", "FLI Dataset:Multi-ROI Single-Pixel NLSF Analysis", "FLI Dataset:All ROIs IRF Extraction", "FLI Dataset:All ROIs Decay Fit Non-Interactive (Fast + Individual IRF)", "FLI Dataset:All ROIs Phasor Analysis", "FLI Dataset:All ROIs Decay Fit", "FLI Dataset:Fluorescence Decay Statistics", "FLI Dataset:Update Decay Statistics Graph", "FLI Dataset:Get Decay from ROI", "FLI Dataset:All ROIs Average Lifetimes", "FLI Dataset:Save/Load Local IRFs", "FLI Dataset:Clear Local IRFs", "FLI Dataset:Phasor Calibration Maps (# Gates Series) Script", "FLI Dataset:Calibrated Phasor Map Series", "---- FLI Dataset Series ----", "FLI Dataset Series:Sum All Datasets in Series", "FLI Dataset Series:Add Dataset to Accumulated Dataset", "FLI Dataset Series:Display Accumulated Dataset", "FLI Dataset Series:Clear Dataset Series Sum", "FLI Dataset Series:Time-Series Analysis (NLSF)", "FLI Dataset Series:Time-Series Analysis (Phasor)", "---- Image ----", "Image:Update Image Profile Plots", "Image:Image Histogram Cursor Move", "Image:Image Histogram", "Image:Image Contrast", "Image:Set Image Histogram Cursor Move Flag", "Image:Clear Image Overlay", "Image:Use ROI as Search Area", "Image:Set ROI Diameter", "Image:Save Image Data as TIFF", "Image:Save Displayed Image with Overlay", "Image:Save Image Overlay Only", "Image:Save Image as Hot Pixel Mask", "Image:Change Source Image Color Palette", "Image:Copy Image to Clipboard", "Image:Source Image ROI Selection", "Image:Delete All ROIs", "Image:Delete All Unselected ROIs", "Image:Delete ROI", "Image:Merge All ROIs", "Image:Store ROI", "Image:Source Image ROI Storage", "Image:Export ROI Description to Notebook", "Image:Save ROI", "Image:Load ROI", "Image:Paste ROI Definition", "Image:Clear ROI", "Image:Identify ROIs in Mask Image", "Image:Create Complementary ROI", "Image:Create Contour ROI", "Image:Create ROI(s) from Pixels with Peak above Min_Scriptable", "Image:Create ROI(s) from Pixels with Intensity above Min_Scriptable", "Image:Compute ROI Statistics", "Image:Delete ROI(s) based on ROI Characteristics", "Image:Create ROI Grid", "Image:ROI to Individual Pixel ROIs", "Image:Python Function Source Image Event", "Image:Show Phasor Calibration Map ROI Centers", "Image:Convert ROI to Mask Image", "Image:Mouse Move", "Image:Mouse Up", "Image:Set Source Image Mouse Move Flag", "Image:Add Scale Bar Overlay", "Image:Delete Existing ROIs Option", "Image:Overlay ROI Median", "Image:Check Current ROI", "Image:Update True Pixel Value", "---- Decay ----", "Decay:Clear IRF/Reference Plot", "Decay:Add Decay to Graph", "Decay:Smoothen Plot", "Decay:Smoothen Plot Tail", "Decay:Average Selected Plots", "Decay:Extract IRF", "Decay:Optimal IRF Extraction", "Decay:Threshold IRF", "Decay:Fit to Model IRF", "Decay:Fit IRF to Square Gate", "Decay:Fit IRF to Logistic Square Gate", "Decay:Fit IRF to Tilted Logistic Square Gate", "Decay:Create Bounding Cursors Set", "Decay:Export Bounding Cursors Definition to Notebook", "Decay:Denoise Plot", "Decay:Compute Cumulative Function", "Decay:Use as Reference Decay", "Decay:Show Reference Decay/IRF", "Decay:Extrapolate Decay", "Decay:Create Head & Tail Bounding Cursors", "Decay:Store Cursor-defined Head & Tail Fractions", "Decay:Rebin Plot", "Decay:1-Normalize Decay", "Decay:[0-1]-Normalize Plot", "Decay:Straighten Decay", "Decay:Shift Decay", "Decay:Fold Decay", "Decay:Fit Decay", "Decay:Global Fit of Selected Decays", "Decay:Post Global Fit Script", "Decay:Add Global Fit Parameters to Graph", "Decay:Add Decay Parameter(s) to Plot (Graph)", "Decay:Export Decay to Phasor Graph", "Decay:Compute Average Lifetime", "Decay:Plot Convolution", "Decay:Graph Tip Strip Update", "---- Decay Statistics ----", "Decay Statistics:Tip Strip Update", "---- Intensity Time Trace ----", "Intensity Time Trace:Use File Timestamp", "Intensity Time Trace:Load Intensity Corrections File", "Intensity Time Trace:Clear Intensity Corrections File", "Intensity Time Trace:Tip Strip Update", "---- Phasor Plot ----", "Phasor Plot:Build Phasor Plot", "Phasor Plot:Change Phasor Plot Color Palette", "Phasor Plot:Adjust Phasor Plot Display Range", "Phasor Plot:Highlight Image ROI in Phasor Plot", "Phasor Plot:Save Phasor Plot Image with Overlay", "Phasor Plot:Export Complex Phasor Map", "Phasor Plot:Export Phasor Ratio Map", "Phasor Plot:Export Average Lifetime Map", "Phasor Plot:Compute Phase Lifetime Histogram", "Phasor Plot:Compute Phasor Ratio Histogram", "Phasor Plot:Compute Phase Lifetime vs Intensity Scatter Plot", "Phasor Plot:Weber 2-Component Decomposition", "Phasor Plot:Update Phasor Color Map Vertices", "Phasor Plot:Clear Phasor Overlay", "Phasor Plot:Use Segment Extremities as References", "Phasor Plot:Use UC/Segment Intersections as References", "Phasor Plot:Use UC/Principal Axis Intersections as References", "Phasor Plot:Use UC/Linear Fit Intersections as References", "Phasor Plot:Update Phasor Plot Reference", "Phasor Plot:Show Local Phasor Info in Phasor Plot", "Phasor Plot:Update Phasor Plot State", "Phasor Plot:Phasor Plot ROI Storage", "Phasor Plot:Phasor Plot ROI Selection", "Phasor Plot:Python Function Phasor Plot Event", "Phasor Plot:Overlay Phasor ROI, Ratio or Map in Source Image", "Phasor Plot:Compute Decay of Selected Phasors", "Phasor Plot:Phasor at Image Pixel", "Phasor Plot:Mouse Move", "Phasor Plot:Mouse Up", "Phasor Plot:Display Range Mouse Move", "Phasor Plot:Set Mouse Move Flag", "Phasor Plot:Update True Phasor Plot Value", "---- Phasor Graph ----", "Phasor Graph:Get Phasor Value", "Phasor Graph:Create New Phasor Plot Dialog", "Phasor Graph:Update Last Phasor Value", "Phasor Graph:Update Phasor (m, phi)", "Phasor Graph:Remove Single Phasor from Plot", "Phasor Graph:Add Single Phasor to Plot", "Phasor Graph:Remove Phasor Plot", "Phasor Graph:Remove Selected Phasor Plots", "Phasor Graph:Clear Phasor Data", "Phasor Graph:Clear Phasor Graph", "Phasor Graph:Cursor Move", "Phasor Graph:Draw Cursor Connecting Line", "Phasor Graph:Clear Cursor Connecting Line", "Phasor Graph:Find UC Intersection", "Phasor Graph:Use UC/Cursor-Defined Line Intersections", "Phasor Graph:Use Selected Plots Fitted Line/UC Intersections", "Phasor Graph:Use Selected Plots Principal Axis/UC Intersections", "Phasor Graph:Show Single Phasor", "Phasor Graph:Save Single Phasor Plot", "Phasor Graph:Save All Phasor Plots", "Phasor Graph:Load Phasor Plot(s)", "Phasor Graph:Phasor Multiplication", "Phasor Graph:Compute Average Phasor", "Phasor Graph:Compute Multiple Average Phasors (Selected Plots)", "Phasor Graph:Export Single Phasor Plot Phase Lifetimes", "Phasor Graph:Parameter 2 vs Parameter 1 Scatter Plot", "Phasor Graph:Use Cursor n Location", "Phasor Graph:Set Reference n to Current Phase Lifetime Value", "Phasor Graph:Set Reference n to Lifetime Value", "Phasor Graph:Set Cursor n Location", "Phasor Graph:Save Phasor Graph Image", "Phasor Graph:Update SEPL Plot", "Phasor Graph:Export Single Phasor Plot Data", "Phasor Graph:Export Selected Phasor Plots Data", "Phasor Graph:Python Function Phasor Graph Event", "Phasor Graph:Tip Strip Update", "---- Calibration ----", "Calibration:Set Calibration Type", "Calibration:Load/Save Phasor Calibration", "Calibration:Load/Save Phasor Calibration Series", "Calibration:Load/Save Phasor Calibration Map", "Calibration:Use as Calibration", "Calibration:Compute Optimal Calibration from Phasor References", "Calibration:Clear Phasor Calibration", "Calibration:Single Phasor Calibration Information", "Calibration:Use as Calibration Series", "Calibration:Use as Calibration Map", "Calibration:Clear Calibration Series", "Calibration:Phasor Calibration Series Information", "Calibration:Clear Calibration Map", "Calibration:Phasor Calibration Map Information", "Calibration:Apply Phasor Calibration", "Calibration:Update Single Plot Calibration", "Calibration:Update Multiple Plots Calibration", "Calibration:Clear Single Plot Calibration", "Calibration:Clear All Plots Calibrations", "Calibration:Clear Plot(s) Calibration(s)?", "---- Phasor Ratio ----", "Phasor Ratio:Clear Reference n", "Phasor Ratio:Toggle Selected Plot(s)  Lock to Reference 1", "Phasor Ratio:Use as Reference n", "Phasor Ratio:Send Reference n to Notebook", "Phasor Ratio:Toggle Selected Plot(s)  Lock to Reference 2", "Phasor Ratio:Compute Phasor Ratio at Mouse Location", "Phasor Ratio:Compute Phasor Plot's Average Phasor Ratio", "Phasor Ratio:Compute Time-Series Phasor Ratios", "Phasor Ratio:Fit Line to Phasor Ratio Plot", "Phasor Ratio:Save References", "Phasor Ratio:Load References", "Phasor Ratio:Update Phasor Reference 1", "Phasor Ratio:Update Phasor Reference 2", "Phasor Ratio:Move Cursor n to Reference n", "Phasor Ratio:Use as Phasor Reference 1 Lifetime", "Phasor Ratio:Use as Phasor Reference 2 Lifetime", "Phasor Ratio:Export Phasor Ratio Map as ASCII", "Phasor Ratio:Tip Strip Update", "---- Lifetime & Other Parameters Graph ----", "Lifetime:Compute Sliced Mean, SDV and CV Plots", "Lifetime:Plot Decay Shifts", "Lifetime:Plot Histogram", "---- Decay Fit Parameter Map ----", "Decay Fit Parameter Map:Export ROI NLSF Data as ASCII", "Decay Fit Parameter Map:Set Decay Fit Parameter Map Selection", "Decay Fit Parameter Map:Build Decay Fit Parameter Map", "Decay Fit Parameter Map:Change Decay Fit Parameter Map Color Palette", "Decay Fit Parameter Map:Export Decay Fit Parameter Map Data as ASCII", "Decay Fit Parameter Map:Export All Decay Fit Parameter Maps Data as ASCII", "Decay Fit Parameter Map:Selected Parameter Scatterplot", "Decay Fit Parameter Map:Parameter 2 vs Parameter 1 Scatterplot", "Decay Fit Parameter Map:Save Decay Fit Parameter Map Image", "Decay Fit Parameter Map:Save-Load IRFs & Fit Data", "Decay Fit Parameter Map:Update Local Decay Plots", "Decay Fit Parameter Map:Python Function Decay Fit Parameters Map Event", "Decay Fit Parameter Map:Overlay Decay Fit Parameter Map in Source Image", "Decay Fit Parameter Map:Selected Parameter vs Intensity Scatterplot", "Decay Fit Parameter Map:Mouse Up", "Decay Fit Parameter Map:Mouse Move", "Decay Fit Parameter Map:Display Range Mouse Move", "Decay Fit Parameter Map:Change Map Resolution", "Decay Fit Parameter Map:Variance Significance Maps", "Decay Fit Parameter Map:Fit Result Constraints Window", "---- Parameter Map ----", "Parameter Map:Export ROI Parameters Data as ASCII", "Parameter Map:Delete Parameter Map Set", "Parameter Map:Update Parameter List", "Parameter Map:Build Parameter Map", "Parameter Map:Change Parameter Map Color Palette", "Parameter Map:Export Parameter Map Data as ASCII", "Parameter Map:Export All Parameter Maps Data as ASCII", "Parameter Map:Selected Parameter Scatterplot", "Parameter Map:Parameter 2 vs Parameter 1 Scatterplot", "Parameter Map:Selected Parameter vs Intensity Scatterplot", "Parameter Map:Save Parameter Map Image", "Parameter Map:Save-Load IRFs & Parameter Maps (TODO)", "Parameter Map:Set Parameter Map Selection", "Parameter Map:Python Function Parameter Map Event", "Parameter Map:Overlay Parameter Map in Source Image", "Parameter Map:Update Local Decay Plots", "Parameter Map:Mouse Up", "Parameter Map:Mouse Move", "Parameter Map:Display Range Mouse Move", "---- Generic Graph ----", "Generic Graph:Generic XY Graph Event", "Generic Graph:Python Function XY Graph Event", "Generic Graph:New Plot", "Generic Graph:Save Plot", "Generic Graph:XY Plot Histogram", "Generic Graph:Set XY Graph Plot Name", "Generic Graph:Set Last Cursor Style", "Generic Graph:Tip Strip Update", "---- GUI ----", "GUI:Start Script", "GUI:Type of Displayed Image Changed", "GUI:Gate Image Slide Changed", "GUI:Show Busy Icon", "GUI:Show Busy Icon & Abort Button", "GUI:Hide Busy Icon", "GUI:Hide Busy Icon & Abort Button", "GUI:Abort", "GUI:End Script", "GUI:Start Timing", "GUI:End Timing", "GUI:Set State Indicator", "GUI:Send Parameters JSON Strings to Clipboard", "GUI:Set Gate Step", "GUI:Idle", "GUI:Initialization", "GUI:Quit", "GUI:Increment Dataset Index", "GUI:Set Dataset Index to -1", "GUI:Time Series Slider Moved", "GUI:Time Series Slider Changed", "GUI:Toggle Playback or Loop", "GUI:Playback Script", "GUI:Set Phasor Frequency", "GUI:Open Window", "GUI:Start Test Script", "GUI:End Test Script", "GUI:Set Verbose Mode", "GUI:Set Verbose Settings Mode", "DEBUG"}
  T82 = typedef "Palette.lvlib/Image Palette Information.ctl" = cluster{"Palette Name [# Colors,int?,inv?]":string, "Palette Type":T83, "Palette Colors":u32[], "Interpolate?":bool}
  T83 = typedef "Image.lvlib/Image Display Palette Type.ctl" = u32
  T84 = typedef "Palette.lvlib/Interpolated Color Scale Definition.ctl" = cluster{"Color Scale Points":cluster{"Value":dbl, "Color":u32}[], "Color Scale Name":string}
  T85 = typedef "Notebook.lvlib/Notebook Parameters List.ctl" = enum16{"First Opening?", "Saved Notebook?", "Saved Notebook Path", "Beep on Error?", "Notebook Themes", "Current Theme Name"}
  T86 = typedef "AlliGator GUI.lvlib/AlliGator Skippable Windows Status.ctl" = cluster{"Dialog Window Name":string, "Is skipped":bool}
  T87 = typedef "AlliGator Settings.lvlib/AlliGator Quantities.ctl" = string[]
  T88 = typedef "XY Graph Add-Ons.lvlib/XY Graph Plot Data.ctl" = cluster{"X Array":dbl[], "Y Array":dbl[]}
  T89 = typedef "AlliGator Settings Window Messages.ctl" = enum16{"Idle", "Subscribe", "Unsubscribe", "Refresh Parameter", "Refresh All Parameters", "Quit"}
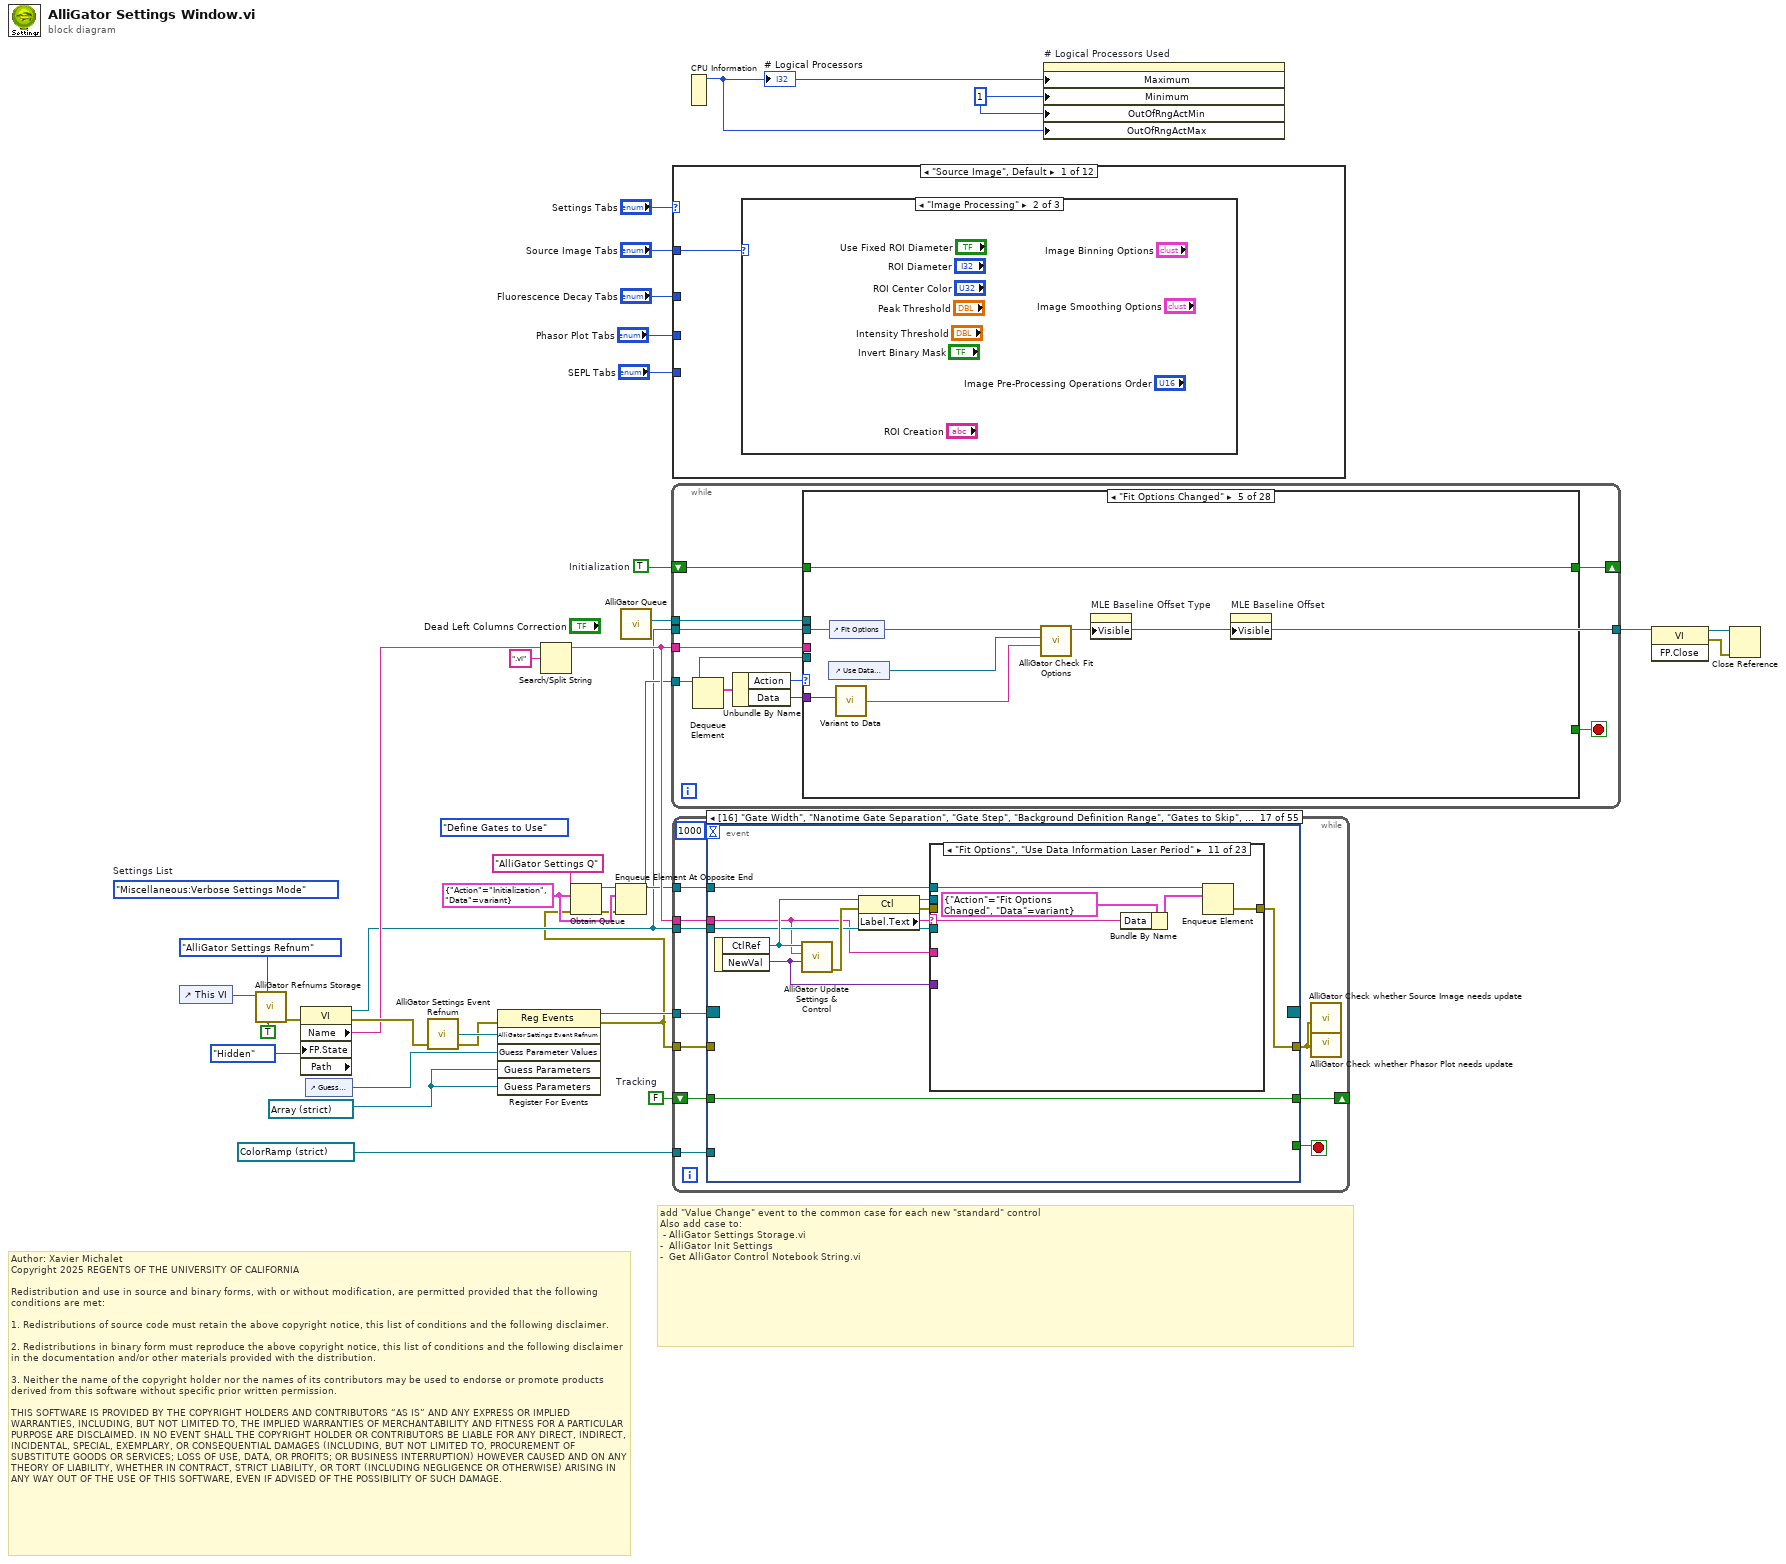
[diagram p0: block diagram]
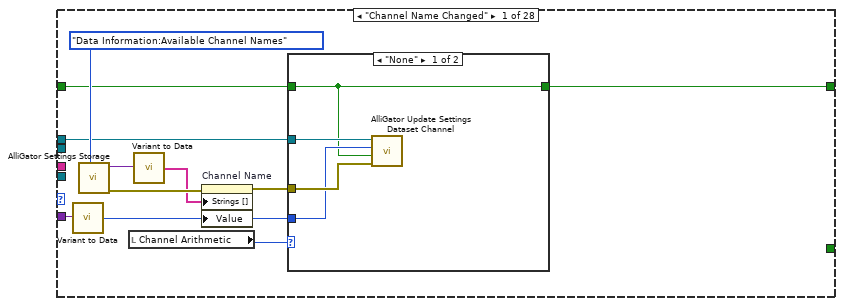
[diagram p2: hidden frame]
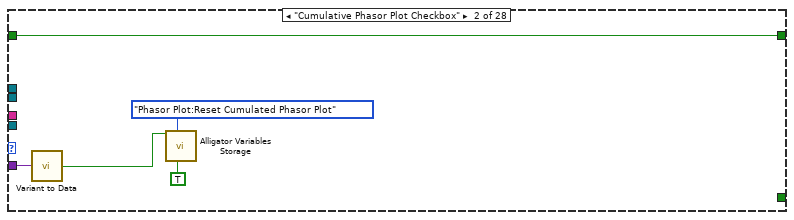
[diagram p4: hidden frame]
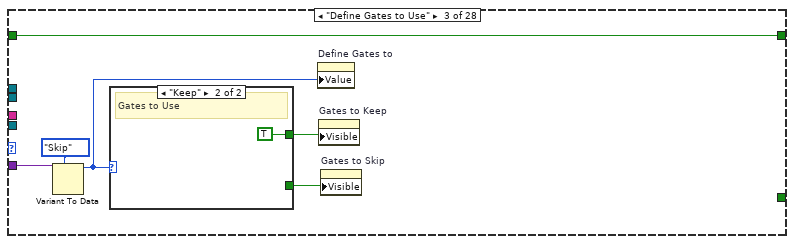
[diagram p5: hidden frame]
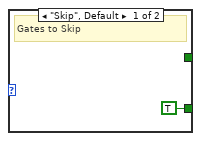
[diagram p6: hidden frame]
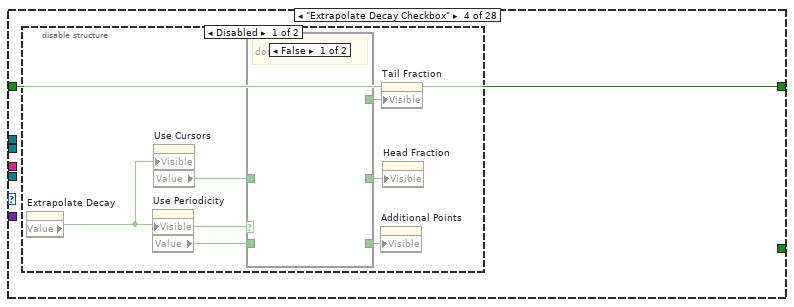
[diagram p7: hidden frame]
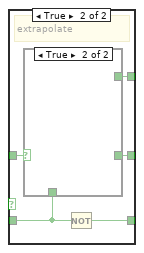
[diagram p8: hidden frame]
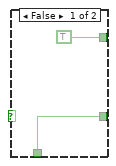
[diagram p9: hidden frame]
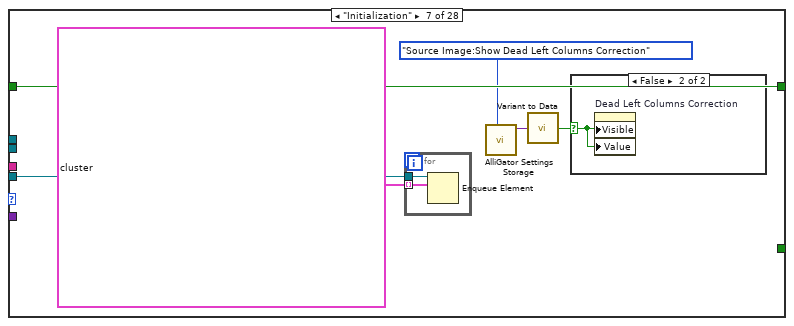
[diagram p12: hidden frame]
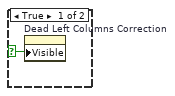
[diagram p13: hidden frame]
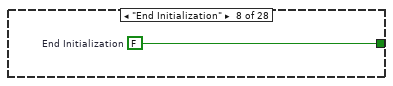
[diagram p14: hidden frame]
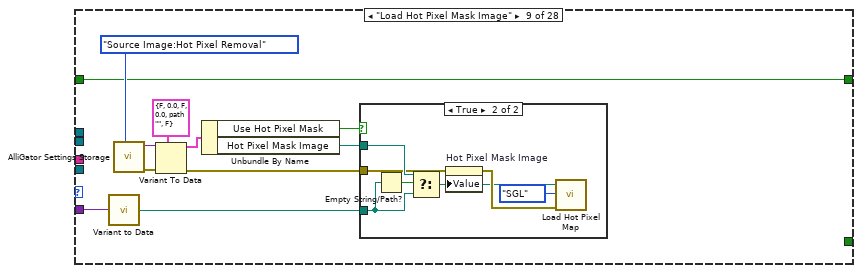
[diagram p15: hidden frame]
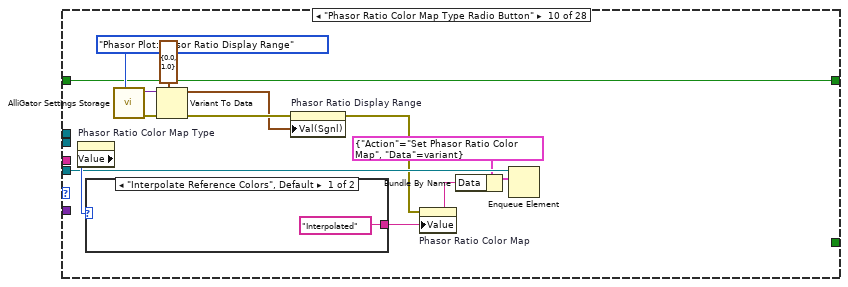
[diagram p17: hidden frame]
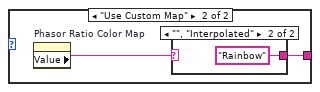
[diagram p18: hidden frame]
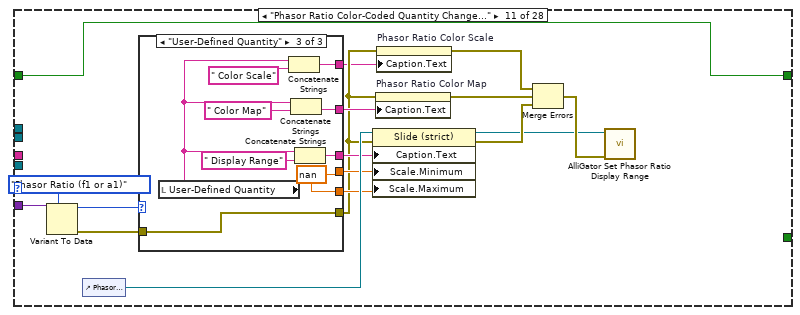
[diagram p20: hidden frame]
diagram:
  w5 = TRUE  # Initialization
  (unwired) AlliGator_Settings_List."Miscellaneous:Verbose Settings Mode"  # Settings List
  w10 = 1 ("Data Entry Limits:Minimum")
  (unwired) AlliGator_Settings_Q_Action."Define Gates to Use" ("Action")
  w17 = T77 {"Action"=enum."Initialization", "Data"=variant} ("AlliGator Settings Q Element")
  w25 = FALSE  # Tracking
  w26 = refnum<vi> refnum ("Guess Parameters")
  # "Author: Xavier Michalet\nCopyright 2025 REGENTS OF THE UNIVERSITY OF CALIFORNIA\n\nRedistribution and use in source and binary forms, with or without modification, are permitted provided that the following conditions are met:\n\n1. Redistributions of source code must retain the above copyright notice, this list of conditions and the following disclaimer.\n\n2. Redistributions in binary form must reproduce the above copyright notice, this list of conditions and the following disclaimer in the documentation and/or other materials provided with the distribution.\n\n3. Neither the name of the copyright holder nor the names of its contributors may be used to endorse or promote products derived from this software without specific prior written permission.\n\nTHIS SOFTWARE IS PROVIDED BY THE COPYRIGHT HOLDERS AND CONTRIBUTORS “AS IS” AND ANY EXPRESS OR IMPLIED WARRANTIES, INCLUDING, BUT NOT LIMITED TO, THE IMPLIED WARRANTIES OF MERCHANTABILITY AND FITNESS FOR A PARTICULAR PURPOSE ARE DISCLAIMED. IN NO EVENT SHALL THE COPYRIGHT HOLDER OR CONTRIBUTORS BE LIABLE FOR ANY DIRECT, INDIRECT, INCIDENTAL, SPECIAL, EXEMPLARY, OR CONSEQUENTIAL DAMAGES (INCLUDING, BUT NOT LIMITED TO, PROCUREMENT OF SUBSTITUTE GOODS OR SERVICES; LOSS OF USE, DATA, OR PROFITS; OR BUSINESS INTERRUPTION) HOWEVER CAUSED AND ON ANY THEORY OF LIABILITY, WHETHER IN CONTRACT, STRICT LIABILITY, OR TORT (INCLUDING NEGLIGENCE OR OTHERWISE) ARISING IN ANY WAY OUT OF THE USE OF THIS SOFTWARE, EVEN IF ADVISED OF THE POSSIBILITY OF SUCH DAMAGE."
  # "add \"Value Change\" event to the common case for each new \"standard\" control\nAlso add case to:\n - AlliGator Settings Storage.vi\n-  AlliGator Init Settings\n-  Get AlliGator Control Notebook String.vi"
  n1 = control-ref of="This VI"() -> (w1:refnum<vi>)
  n2 = call "AlliGator Refnums Storage.vi"("Get(F)/Set"=TRUE, "AlliGator Refnum List"=AlliGator_Refnums_List."AlliGator Settings Refnum", "Data in"=w1) -> ("Error Out"=w8:errorcluster)  [unwired: 7 in, 1 out]
  n3 = property class="VI" props=["Name", "FP.State", "Path"](error in=w8, "FP.State"=T75."Hidden" ("Front Panel Window:State")) -> (reference out=w15:refnum<vi>, error out=w32:errorcluster, "Name"=w31:string)  [unwired: 1 in, 1 out]
  n4 = control-ref of="Guess Parameter Values"() -> (w27:refnum<vi>)
  n5 = call "AlliGator Settings Event Refnum.vi"("Error In"=w32) -> ("AlliGator Settings Event Refnum"=w35:refnum<user-event>, "Error Out"=w34:errorcluster)  [unwired: 7 in]
  n6 = register-events(error in=w34, w35, w27, w26, w26) -> (reference out=w33:refnum<event-registration>, error out=w14:errorcluster)  [unwired: 1 in]
  n7 = Search/Split String(string=w31, search string/char (-)=".vi") -> (substring before match=w20:string)  [unwired: 1 in, 2 out]
  n8 = Obtain Queue(name (unnamed)="AlliGator Settings Q", element data type=w17, error in (no error)=w14) -> (queue out=w21:refnum<queue>, error out=w16:errorcluster)  [unwired: 2 in, 1 out]
  n9 = Enqueue Element At Opposite End(queue=w21, element=w17, error in (no error)=w16) -> (queue out=w18:refnum<queue>)  [unwired: 1 in, 2 out]
  n10 = call "AlliGator Queue.vi"() -> ("AlliGator Q"=w19:refnum<queue>)  [unwired: 8 in, 1 out]
  n11 = while {
    tunnel: w18 -> [w40]
    tunnel: w20 -> [w41]
    tunnel: w19 -> [w39]
    tunnel: w15 -> [w38]
    tunnel: [w38] -> w12
    shift-right: [w36] -> _
    shift-left: w5 -> [w37]
    stop <- w43 stop-if-true
    n12 = Dequeue Element(queue=w40) -> (element=w45:T77)  [unwired: 2 in, 3 out]
    n13 = Unbundle By Name(w45) -> ("Action"=w44:T76, "Data"=w42:variant)
    n14 = case shown="\"Fit Options Changed\"" w44 {
      tunnel: [_ _ _ _ _ _ _ _ _ _ _ _ _ TRUE _ _ _ _ _ _ _ _ _ _ _ _ _ _] -> w43
      tunnel: w42 -> [w54 w66 w72 _ w93 _ _ _ w117 _ w159 _ _ _ _ _ w223 _ _ _ _ _ _ _ w322 _ _ w338]
      tunnel: w41 -> [_ _ _ _ _ _ _ _ _ _ _ _ _ _ _ _ _ _ _ _ _ _ w301 _ _ _ _ _]
      tunnel: w40 -> [_ _ _ _ _ _ w101 _ _ w136 _ _ _ _ _ _ _ _ _ _ _ _ _ _ _ _ _ _]
      tunnel: w39 -> [w50 _ _ _ _ _ _ _ _ _ _ _ _ _ _ w215 _ _ _ _ _ _ _ w319 _ _ w335 _]
      tunnel: w38 -> [_ _ _ _ _ _ _ _ _ _ _ _ _ _ w209 _ _ _ _ w287 _ _ w313 _ _ _ _ _]
      tunnel: w37 -> [w47 w62 w67 w75 w89 w95 w99 _ w107 w126 w146 w192 w200 w201 w203 w210 w220 w274 w281 w283 w288 w290 w295 w318 w321 w333 w334 w337]
      tunnel: [w46 w62 w67 w75 w89 w95 w99 w106 w107 w126 w146 w192 w200 w201 w203 w210 w220 w274 w281 w283 w288 w290 w295 w318 w321 w333 w334 w337] -> w36
      frame "Channel Name Changed" {
        n15 = call-poly "Variant to Data.vi"("Variant"=w54) -> ("U16 Value"=w51:u16)  [unwired: 8 in]
        n16 = call "AlliGator Settings Storage.vi"("AlliGator Settings List"=AlliGator_Settings_List."Data Information:Available Channel Names") -> ("Error Out"=w53:errorcluster, "Variant Data out"=w56:variant)  [unwired: 9 in]
        n17 = local read "Channel Arithmetic"() -> (w52:T11)
        n18 = call-poly "Variant to Data.vi"("Variant"=w56) -> ("String Array"=w48:string[])  [unwired: 8 in]
        n19 = property on="Channel Name" class="Ring (strict)"(error in=w53, "Strings []"=w48, "Value"=w51) -> (error out=w49:errorcluster)  [unwired: 1 in, 1 out]
        n20 = case shown="\"None\"" w52 {
          tunnel: w51 -> [w58 _]
          tunnel: w50 -> [w60 _]
          tunnel: w49 -> [w59 _]
          tunnel: w47 -> [w57 w61]
          tunnel: [w57 w61] -> w46
          frame "None" {
            n21 = call "AlliGator Update Settings Dataset Channel.vi"("error in (no error)"=w59, "Initialization?"=w57, "Selected Channel"=w58, "AlliGator Queue"=w60) -> ()  [unwired: 7 in, 1 out]
          }
          frame "INT-G2", Default {
          }
        }
      }
      frame "Cumulative Phasor Plot Checkbox" {
        n22 = call-poly "Variant to Data.vi"("Variant"=w66) -> ("Value"=w65:bool)  [unwired: 8 in]
        n23 = call "Alligator Variables Storage.vi"("Get(F)/Set"=TRUE, "AlliGator Variable"=AlliGator_Variables_List."Phasor Plot:Reset Cumulated Phasor Plot" ("Alligator Variable"), "Data in"=w65) -> ()  [unwired: 6 in, 3 out]
      }
      frame "Define Gates to Use" {
        n24 = Variant To Data(type=AlliGator_Define_Gates_to."Skip" ("Define Gates to"), Variant=w72) -> (data=w68:T13)  [unwired: 1 in, 1 out]
        n25 = case shown="\"Keep\"" w68 {
          tunnel: [TRUE ("Visible") _] -> w70
          tunnel: [_ TRUE ("Visible")] -> w69
          frame "Skip", Default {
            # "Gates to Skip"
          }
          frame "Keep" {
            # "Gates to Use"
          }
        }
        n26 = property on="Define Gates to" class="RadioBtnsControl (strict)"("Value"=w68) -> ()  [unwired: 2 in, 2 out]
        n27 = property on="Gates to Keep" class="Clust (strict)"("Visible"=w69) -> ()  [unwired: 2 in, 2 out]
        n28 = property on="Gates to Skip" class="Clust (strict)"("Visible"=w70) -> ()  [unwired: 2 in, 2 out]
      }
      frame "Extrapolate Decay Checkbox" {
        n29 = disable-structure shown="Disabled" {
          frame Disabled {
            n30 = property on="Extrapolate Decay" class="Bool (strict)"() -> ("Value"=w79:bool)  [unwired: 2 in, 2 out]
            n31 = property on="Use Periodicity" class="Bool (strict)"("Visible"=w79) -> ("Value"=w81:bool)  [unwired: 2 in, 2 out]
            n32 = property on="Use Cursors" class="Bool (strict)"("Visible"=w79) -> ("Value"=w76:bool)  [unwired: 2 in, 2 out]
            n33 = case shown="False" w79 {
              tunnel: w81 -> [_ w82]
              tunnel: [_ w83] -> w80
              tunnel: w76 -> [_ w86]
              tunnel: [_ w84] -> w78
              tunnel: [_ w85] -> w77
              frame False {
                # "don't extrapolate"
              }
              frame True {
                # "extrapolate"
                n34 = case shown="True" w86 {
                  tunnel: [TRUE ("Use Cursors") _] -> w85
                  tunnel: [w87 _] -> w84
                  tunnel: w82 -> [w87 _]
                  frame False {
                  }
                  frame True {
                  }
                }
                n35 = Not(x=w82) -> (.not. x?=w83:bool)
              }
            }
            n36 = property on="Additional Points" class="DigNum (strict)"("Visible"=w80) -> ()  [unwired: 2 in, 2 out]
            n37 = property on="Tail Fraction" class="DigNum (strict)"("Visible"=w77) -> ()  [unwired: 2 in, 2 out]
            n38 = property on="Head Fraction" class="DigNum (strict)"("Visible"=w78) -> ()  [unwired: 2 in, 2 out]
          }
          frame Enabled {
          }
        }
      }
      frame "Fit Options Changed" {
        n39 = control-ref of="Use Data Information Laser Period"() -> (w92:refnum<vi>)
        n40 = control-ref of="Fit Options"() -> (w94:refnum<vi>)
        n41 = call-poly "Variant to Data.vi"("Variant"=w93) -> ("String"=w91:string)  [unwired: 8 in]
        n42 = call "AlliGator Check Fit Options.vi"("Modified Option"=w91, "Use Data Information Period Refnum"=w92, "Fit Options Refnum"=w94) -> ("MLE Options Visible?"=w90:bool)  [unwired: 7 in, 1 out]
        n43 = property on="MLE Baseline Offset Type" class="RadioBtnsControl (strict)"("Visible"=w90) -> ()  [unwired: 2 in, 2 out]
        n44 = property on="MLE Baseline Offset" class="DigNum (strict)"("Visible"=w90) -> ()  [unwired: 2 in, 2 out]
      }
      frame "Idle", Default {
      }
      frame "Initialization" {
        n45 = for {
          tunnel: w101 -> [w105]
          tunnel: T77[] [{"Action"=enum."Refresh All Parameters", "Data"=variant}, {"Action"=enum."Extrapolate Decay Checkbox", "Data"=variant}, {"Action"=enum."Phasor Ratio Color Map Type Radio Button", "Data"=variant}, {"Action"=enum."Shift Decay Checkbox", "Data"=variant}, {"Action"=enum."Use Cursor (Extrapolate) Checkbox", "Data"=variant}, {"Action"=enum."Baseline Subtraction Method", "Data"=variant}, {"Action"=enum."Show Window", "Data"=variant}, {"Action"=enum."Define Gates to Use", "Data"=variant}, {"Action"=enum."Update Natural Frequency", "Data"=variant}, {"Action"=enum."Load Hot Pixel Mask Image", "Data"=variant}, {"Action"=enum."Fit Options Changed", "Data"=variant}, {"Action"=enum."Phasor Ratio Color-Coded Quantity Changed", "Data"=variant}, {"Action"=enum."Get Phasor Ratio Color Scale Hi/Lo Colors", "Data"=variant}, {"Action"=enum."End Initialization", "Data"=variant}] ("element") -> [w104] mode=indexing
          n46 = Enqueue Element(queue=w105, element=w104) -> ()  [unwired: 2 in, 3 out]
        }
        n47 = call "AlliGator Settings Storage.vi"("AlliGator Settings List"=AlliGator_Settings_List."Source Image:Show Dead Left Columns Correction") -> ("Variant Data out"=w97:variant)  [unwired: 9 in, 1 out]
        n48 = call-poly "Variant to Data.vi"("Variant"=w97) -> ("Value"=w96:bool)  [unwired: 8 in]
        n49 = case shown="False" w96 {
          selector: w96 -> [w102 w103]
          frame True {
            n50 = property on="Dead Left Columns Correction" class="Bool (strict)"("Visible"=w102) -> ()  [unwired: 2 in, 2 out]
          }
          frame False {
            n51 = property on="Dead Left Columns Correction" class="Bool (strict)"("Visible"=w103, "Value"=w103) -> ()  [unwired: 2 in, 2 out]
          }
        }
      }
      frame "End Initialization" {
        w106 = FALSE  # End Initialization
      }
      frame "Load Hot Pixel Mask Image" {
        n52 = call-poly "Variant to Data.vi"("Variant"=w117) -> ("Path"=w116:path)  [unwired: 8 in]
        n53 = call "AlliGator Settings Storage.vi"("AlliGator Settings List"=AlliGator_Settings_List."Source Image:Hot Pixel Removal") -> ("Error Out"=w113:errorcluster, "Variant Data out"=w114:variant)  [unwired: 9 in]
        n54 = Variant To Data(error in=w113, type=T3 {"Remove Screamers"=FALSE, "Delta"=0.0, "Equalize Histogram"=FALSE, "Percentile"=0.0, "Hot Pixel Mask Image"=path "", "Use Hot Pixel Mask"=FALSE} ("Image Display Options"), Variant=w114) -> (data=w111:T3, error out=w109:errorcluster)
        n55 = Unbundle By Name(w111) -> ("Use Hot Pixel Mask"=w108:bool, "Hot Pixel Mask Image"=w110:path)
        n56 = case shown="True" w108 {
          tunnel: w116 -> [_ w124]
          tunnel: w110 -> [_ w123]
          tunnel: w109 -> [_ w121]
          frame False {
          }
          frame True {
            n57 = Empty String/Path?(string/path=w124) -> (empty?=w122:bool)
            n58 = Select(t=w123, s=w122, f=w124) -> (s? t:f=w119:path)
            n59 = property on="Hot Pixel Mask Image" class="Path"(error in=w121, "Value"=w119) -> (error out=w120:errorcluster)  [unwired: 1 in, 1 out]
            n60 = call "Load Hot Pixel Map.vi"("Error In"=w120, "Hot Pixel Map Target"=Image_Hot_Pixel_Map_Target."SGL", "Hot Pixel Mask Image Path"=w119) -> ()  [unwired: 7 in, 2 out]
          }
        }
      }
      frame "Phasor Ratio Color Map Type Radio Button" {
        n61 = property on="Phasor Ratio Color Map Type" class="RadioBtnsControl (strict)"() -> ("Value"=w137:T46)  [unwired: 2 in, 2 out]
        n62 = case shown="\"Interpolate Reference Colors\", Default" w137 {
          tunnel: ["Interpolated" w139] -> w133
          frame "Interpolate Reference Colors", Default {
          }
          frame "Use Custom Map" {
            n63 = property on="Phasor Ratio Color Map" class="Str"() -> ("Value"=w140:string)  [unwired: 2 in, 2 out]
            n64 = case shown="\"\", \"Interpolated\"" w140 {
              selector: w140 -> [w141 _]
              tunnel: [w141 "Rainbow"] -> w139
              frame Default {
              }
              frame "", "Interpolated" {
              }
            }
          }
        }
        n65 = call "AlliGator Settings Storage.vi"("AlliGator Settings List"=AlliGator_Settings_List."Phasor Plot:Phasor Ratio Display Range") -> ("Error Out"=w131:errorcluster, "Variant Data out"=w129:variant)  [unwired: 9 in]
        n66 = Variant To Data(error in=w131, type=cluster{dbl, dbl} {0.0, 1.0} ("Phasor Ratio Display Range 2"), Variant=w129) -> (data=w125:cluster{dbl, dbl}, error out=w128:errorcluster)
        n67 = property on="Phasor Ratio Display Range" class="Slide (strict)"(error in=w128, "Val(Sgnl)"=w125) -> (error out=w127:errorcluster)  [unwired: 1 in, 1 out]
        n68 = property on="Phasor Ratio Color Map" class="Str"(error in=w127, "Value"=w133) -> ()  [unwired: 1 in, 2 out]
        n69 = Bundle By Name(cluster=T77 {"Action"=enum."Set Phasor Ratio Color Map", "Data"=variant} ("element"), "Data"=w133) -> (w134:T77)
        n70 = Enqueue Element(queue=w136, element=w134) -> ()  [unwired: 2 in, 3 out]
      }
      frame "Phasor Ratio Color-Coded Quantity Changed" {
        n71 = Variant To Data(type=AlliGator_Phasor_Ratio_Color-Coded_Quantity."Phasor Ratio (f1 or a1)" ("Fit Options"), Variant=w159) -> (data=w157:T47, error out=w153:errorcluster)  [unwired: 1 in]
        n72 = control-ref of="Phasor Ratio Display Range"() -> (w152:refnum<vi>)
        n73 = case shown="\"User-Defined Quantity\"" w157 {
          tunnel: ["Phasor Ratio Color Scale" ("Caption.Text") "Average Lifetime Color Scale" ("Caption.Text") w182] -> w144
          tunnel: ["Phasor Ratio Color Map" ("Caption.Text") "Average Lifetime Color Map" ("Caption.Text") w180] -> w156
          tunnel: ["Phasor Ratio Display Range" ("Caption.Text") "Average Lifetime Display Range" ("Caption.Text") w177] -> w151
          tunnel: [0.0 ("Scale.Range:Minimum") w169 w175] -> w150
          tunnel: [1.0 ("Scale.Range:Maximum") w168 w175] -> w149
          tunnel: [w160 w167 w176] -> w145
          tunnel: w153 -> [w160 w166 w176]
          frame "Phasor Ratio (f1 or a1)", Default {
          }
          frame "Average Lifetime (<tau>_i or <tau>_a))" {
            n74 = call "AlliGator Get-Set Phasor Ratio References.vi"("error in (no error)"=w166) -> ("Reference Lifetime 1"=w171:dbl[unit], "Reference Lifetime 2"=w170:dbl[unit], "error out"=w167:errorcluster)  [unwired: 7 in, 5 out]
            n75 = node(w171) -> (w169:dbl)
            n76 = node(w170) -> (w168:dbl)
          }
          frame "User-Defined Quantity" {
            w175 = nan ("Scale.Range:Minimum")
            n77 = local read "User-Defined Quantity"() -> (w179:string)
            n78 = Concatenate Strings(w179, " Color Scale" ("Caption.Text")) -> (w182:string)
            n79 = Concatenate Strings(w179, " Color Map" ("Caption.Text")) -> (w180:string)
            n80 = Concatenate Strings(w179, " Display Range" ("Caption.Text")) -> (w177:string)
          }
        }
        n81 = property class="Slide (strict)"(reference=w152, error in=w145, "Caption.Text"=w151, "Scale.Minimum"=w150, "Scale.Maximum"=w149) -> (reference out=w147:refnum<vi>, error out=w148:errorcluster)
        n82 = property on="Phasor Ratio Color Map" class="Str"(error in=w145, "Caption.Text"=w156) -> (error out=w154:errorcluster)  [unwired: 1 in, 1 out]
        n83 = property on="Phasor Ratio Color Scale" class="ColRmp (strict)"(error in=w145, "Caption.Text"=w144) -> (error out=w143:errorcluster)  [unwired: 1 in, 1 out]
        n84 = Merge Errors(w143, w154, w148) -> (w155:errorcluster)
        n85 = call "AlliGator Set Phasor Ratio Display Range.vi"("error in (no error)"=w155, "Phasor Ratio Display Range"=w147) -> ()  [unwired: 9 in, 1 out]
      }
      frame "Get Phasor Ratio Color Scale Hi/Lo Colors" {
        n86 = call "AlliGator Settings Storage.vi"("AlliGator Settings List"=AlliGator_Settings_List."Phasor Plot:Color Scale Low Color") -> ("Error Out"=w190:errorcluster, "Variant Data out"=w185:variant)  [unwired: 9 in]
        n87 = call-poly "Variant to Data.vi"("Variant"=w185) -> ("Value"=w184:u32)  [unwired: 8 in]
        n88 = call "AlliGator Settings Storage.vi"("AlliGator Settings List"=AlliGator_Settings_List."Phasor Plot:Color Scale High Color", "Error In"=w190) -> ("Error Out"=w188:errorcluster, "Variant Data out"=w187:variant)  [unwired: 8 in]
        n89 = call-poly "Variant to Data.vi"("Variant"=w187) -> ("Value"=w186:u32)  [unwired: 8 in]
        n90 = property on="Phasor Ratio Color Scale" class="ColRmp (strict)"(error in=w188, "Scale.High Color"=w186, "Scale.Low Color"=w184) -> ()  [unwired: 1 in, 2 out]
      }
      frame "Store Phasor Ratio Color Scale Hi/Lo Colors" {
        w197 = TRUE ("Get(F)/Set")
        n91 = property on="Phasor Ratio Color Scale" class="ColRmp (strict)"() -> (error out=w193:errorcluster, "Scale.High Color"=w195:u32, "Scale.Low Color"=w194:u32)  [unwired: 2 in, 1 out]
        n92 = call "AlliGator Settings Storage.vi"("Get(F)/Set"=w197, "AlliGator Settings List"=AlliGator_Settings_List."Phasor Plot:Color Scale Low Color", "Error In"=w193, "Variant Data in"=w194) -> ("Error Out"=w198:errorcluster)  [unwired: 6 in, 1 out]
        n93 = call "AlliGator Settings Storage.vi"("Get(F)/Set"=w197, "AlliGator Settings List"=AlliGator_Settings_List."Phasor Plot:Color Scale High Color", "Error In"=w198, "Variant Data in"=w195) -> ()  [unwired: 6 in, 2 out]
      }
      frame "Quit" {
      }
      frame "Refresh All Parameters" {
        n94 = call "AlliGator Settings Storage.vi"("AlliGator Settings List"=AlliGator_Settings_List."Miscellaneous:Verbose Settings Mode") -> ("Error Out"=w205:errorcluster, "Variant Data out"=w207:variant)  [unwired: 9 in]
        n95 = call-poly "Variant to Data.vi"("Variant"=w207) -> ("Value"=w206:bool)  [unwired: 8 in]
        n96 = call "AlliGator Refresh All Settings.vi"("Error In"=w205, "Verbose (T)"=w206, "VI Refnum in"=w209) -> ("Error Out"=w204:errorcluster)  [unwired: 8 in]
        n97 = call "Tiny Clear Error.vi"("Error In"=w204) -> ()  [unwired: 8 in, 1 out]
      }
      frame "Send Parameters JSON Strings to Clipboard" {
        n98 = Bundle By Name(cluster=T80 {"AlliGator Q Event"=enum."GUI:Send Parameters JSON Strings to Clipboard", "Data"=variant} ("element"), "Data"="Parameter Names only") -> (w212:T80)
        n99 = Build Array(w212) -> (w213:T80[])
        n100 = Enqueue Element(queue=w215, element=w213) -> ()  [unwired: 2 in, 3 out]
      }
      frame "Set Phasor Ratio Color Map" {
        w217 = AlliGator_Variables_List."Phasor Plot:Phasor Ratio Palette List" ("Alligator Variable")
        n101 = local read "Phasor Ratio Color Map Type"() -> (w221:T46)
        n102 = call "Alligator Variables Storage.vi"("Get(F)/Set"=FALSE, "AlliGator Variable"=w217) -> ("Data out"=w219:variant)  [unwired: 7 in, 2 out]
        n103 = call-poly "Variant to Data.vi"("Variant"=w219) -> ("String Array"=w218:string[])  [unwired: 8 in]
        n104 = call-poly "Variant to Data.vi"("Variant"=w223) -> ("String"=w222:string)  [unwired: 8 in]
        n105 = case shown="\"Use Custom Map\"" w221 {
          tunnel: w222 -> [w226 _]
          tunnel: w218 -> [w225 _]
          tunnel: w217 -> [w224 _]
          frame "Use Custom Map" {
            n106 = case shown="Default" w226 {
              selector: w226 -> [_ w237]
              tunnel: w225 -> [w228 w235]
              tunnel: w224 -> [w227 w233]
              frame "Edit Palette List..." {
                n107 = call "Edit Image Palette List Dialog.vi"("Palette List (in)"=w228) -> ("Palette List (out)"=w230:string[])  [unwired: 10 in]
                n108 = call "Alligator Variables Storage.vi"("Get(F)/Set"=TRUE, "AlliGator Variable"=w227, "Data in"=w230) -> ()  [unwired: 6 in, 3 out]
              }
              frame Default {
                w241 = TRUE ("Get(F)/Set")
                n109 = call "Get User Palette Choice.vi"("Palette"=w237) -> ("Error Out"=w244:errorcluster, "Palette Colors"=w247:u32[], "Palette Type"=w248:T83, "Palette Name (# Colors)"=w234:string, "Interpolate?"=w243:bool, "Built-in Palette?"=w232:bool)  [unwired: 3 in, 2 out]
                n110 = Bundle(cluster=T82 {"Palette Name [# Colors,int?,inv?]"="", "Palette Type"=0, "Palette Colors"=[], "Interpolate?"=FALSE} ("Image Display Palette Information"), "Palette Name [# Colors,int?,inv?]"=w234, "Palette Type"=w248, "Palette Colors"=w247, "Interpolate?"=w243) -> (w239:T82)
                n111 = call "Alligator Variables Storage.vi"("Get(F)/Set"=w241, "AlliGator Variable"=AlliGator_Variables_List."Phasor Plot:Phasor Ratio Palette Information" ("Alligator Variable"), "Error In"=w244, "Data in"=w239) -> ("Error Out"=w240:errorcluster)  [unwired: 5 in, 2 out]
                n112 = local write "Phasor Ratio Color Map"(w234) -> ()
                n113 = control-ref of="Phasor Ratio Color Scale"() -> (w231:refnum<vi>)
                n114 = call "AlliGator Settings Storage.vi"("Get(F)/Set"=w241, "AlliGator Settings List"=AlliGator_Settings_List."Phasor Plot:Phasor Ratio Color Map", "Error In"=w240, "Variant Data in"=w234) -> ("Error Out"=w238:errorcluster)  [unwired: 6 in, 1 out]
                n115 = call "Set Color Ramp Palette v3.vi"("error in (no error)"=w238, "Image Display Palette Information"=w239, "ColorRamp in"=w231) -> ("Error Out"=w236:errorcluster)  [unwired: 6 in, 2 out]
                n116 = case shown="False" w232 {
                  tunnel: w236 -> [w255 _]
                  tunnel: w234 -> [w254 _]
                  tunnel: w235 -> [w253 _]
                  tunnel: w233 -> [w251 _]
                  frame False {
                    n117 = Build Array (concatenate)(w253, w254) -> (w252:string[])
                    n118 = call "Remove Duplicates From 1D Array.vim"("array"=w252) -> ("array with duplicates removed"=w250:string[])  [unwired: 10 in]
                    n119 = call "Alligator Variables Storage.vi"("Get(F)/Set"=TRUE, "AlliGator Variable"=w251, "Error In"=w255, "Data in"=w250) -> ()  [unwired: 5 in, 3 out]
                  }
                  frame True {
                  }
                }
              }
            }
          }
          frame "Interpolate Reference Colors" {
            w265 = TRUE ("Get(F)/Set")
            n120 = property on="Reference 1" class="ColBox"() -> ("Value"=w259:u32)  [unwired: 2 in, 2 out]
            n121 = property on="Reference 2" class="ColBox"() -> ("Value"=w258:u32)  [unwired: 2 in, 2 out]
            n122 = call "AlliGator Get Phasor Ratio Interpolated Color Scale.vi"("Reference 2 Color"=w258, "Reference 1 Color"=w259) -> ("Error Out"=w260:errorcluster, "Interpolated Color Scale Definition"=w261:T84)  [unwired: 8 in]
            n123 = call "Get User Palette Choice.vi"("Error In"=w260, "Interpolated Color Scale Definition"=w261, "Palette"="Interpolated") -> ("Error Out"=w269:errorcluster, "Palette Colors"=w272:u32[], "Palette Type"=w273:T83, "Palette Name (# Colors)"=w267:string, "Interpolate?"=w268:bool)  [unwired: 1 in, 3 out]
            n124 = control-ref of="Phasor Ratio Color Scale"() -> (w256:refnum<vi>)
            n125 = Bundle(cluster=T82 {"Palette Name [# Colors,int?,inv?]"="", "Palette Type"=0, "Palette Colors"=[], "Interpolate?"=FALSE} ("Image Display Palette Information"), "Palette Name [# Colors,int?,inv?]"=w267, "Palette Type"=w273, "Palette Colors"=w272, "Interpolate?"=w268) -> (w263:T82)
            n126 = call "Alligator Variables Storage.vi"("Get(F)/Set"=w265, "AlliGator Variable"=AlliGator_Variables_List."Phasor Plot:Phasor Ratio Palette Information" ("Alligator Variable"), "Error In"=w269, "Data in"=w263) -> ("Error Out"=w264:errorcluster)  [unwired: 5 in, 2 out]
            n127 = call "AlliGator Settings Storage.vi"("Get(F)/Set"=w265, "AlliGator Settings List"=AlliGator_Settings_List."Phasor Plot:Phasor Ratio Color Map", "Error In"=w264, "Variant Data in"=w267) -> ("Error Out"=w262:errorcluster)  [unwired: 6 in, 1 out]
            n128 = local write "Phasor Ratio Color Map"(w267) -> ()
            n129 = call "Set Color Ramp Palette v3.vi"("error in (no error)"=w262, "Image Display Palette Information"=w263, "ColorRamp in"=w256) -> ()  [unwired: 6 in, 3 out]
          }
        }
      }
      frame "Set SEPL Parameters to Dataset Ones" {
        n130 = local read "Nanotime Gate Separation"() -> (w279:dbl[unit])
        n131 = local read "# Gates"() -> (w278:u32)
        n132 = control-ref of="Gate Parameters"() -> (w277:refnum<vi>)
        n133 = local read "Gate Width"() -> (w280:dbl[unit])
        n134 = property on="Match Laser Period" class="Bool (strict)"("Value"=FALSE ("Match Laser Period")) -> (error out=w275:errorcluster)  [unwired: 2 in, 1 out]
        n135 = call "AlliGator Update Settings SEPL Parameters.vi"("Gate Duration"=w280, "Error In"=w275, "Gate Separation"=w279, "# Gates"=w278, "Gate Parameters Refnum"=w277) -> ()  [unwired: 6 in, 1 out]
      }
      frame "Shift Decay Checkbox" {
        n136 = control-ref of="Decay Shift Parameters"() -> (w282:refnum<vi>)
        n137 = call "AlliGator Update Settings Decay Shift Parameters Visibility.vi"("Shift Parameters Refnum"=w282) -> ()  [unwired: 9 in, 2 out]
      }
      frame "Show Window" {
        # "This updates the Natural Frequency"
        n138 = local read "Extrapolate Decay"() -> (w286:bool)
        n139 = property on="Extrapolate Decay" class="Bool (strict)"("Val(Sgnl)"=w286) -> (error out=w284:errorcluster)  [unwired: 2 in, 1 out]
        n140 = property class="VI"(reference=w287, error in=w284, "FP.State"=T75."Standard" ("Front Panel Window:State")) -> ()  [unwired: 2 out]
      }
      frame "Smooth Decay Checkbox" {
        n141 = disable-structure shown="Enabled" {
          frame Disabled {
            n142 = property on="Smoothen Decay" class="Bool (strict)"() -> ("Value"=w289:bool)  [unwired: 2 in, 2 out]
            n143 = property on="Smoothing Parameter" class="DigNum (strict)"("Visible"=w289) -> ()  [unwired: 2 in, 2 out]
          }
          frame Enabled {
          }
        }
      }
      frame "Update Natural Frequency" {
        n144 = call "AlliGator Compute Natural Frequency.vi"() -> ("Natural Frequency"=w291:dbl[unit])  [unwired: 10 in, 1 out]
        n145 = local write "Natural Frequency"(w291) -> ()
      }
      frame "Update SEPL Parameters" {
        n146 = property on="Gate Type" class="Enum (strict)"() -> ("Value"=w293:T62)  [unwired: 2 in, 2 out]
        n147 = control-ref of="Decay & IRF Parameters"() -> (w300:refnum<vi>)
        n148 = control-ref of="Phasor Parameters"() -> (w297:refnum<vi>)
        n149 = control-ref of="Gate Parameters"() -> (w298:refnum<vi>)
        n150 = control-ref of="Display Parameters"() -> (w299:refnum<vi>)
        n151 = call "Phasor Explorer Update Parameters.vi"("VI in"=w313) -> ("error out"=w312:errorcluster, "Display Parameters"=w303:T53, "Decay & IRF Parameters"=w304:T58, "Gate Parameters"=w305:T61, "Phasor Parameters"=w306:T55)  [unwired: 3 in, 3 out]
        n152 = Build Array(w297, w298, w300, w299) -> (w296:refnum<vi>[])
        n153 = To Variant(anything=w306) -> (Variant=w308:variant)
        n154 = To Variant(anything=w305) -> (Variant=w309:variant)
        n155 = To Variant(anything=w304) -> (Variant=w310:variant)
        n156 = To Variant(anything=w303) -> (Variant=w307:variant)
        n157 = Equal?(x=Phasor_Gate_Type."User-defined" ("Value"), y=w293) -> (x = y?=w292:bool)
        n158 = call <vilib>:"Clear Errors.vi"("error in (no error)"=w312) -> ("error out"=w311:errorcluster)  [unwired: 5 in, 1 out]
        n159 = Build Array(w308, w309, w310, w307) -> (w302:variant[])
        n160 = property on="Edit User-defined Function" class="Bool"("Visible"=w292) -> ()  [unwired: 2 in, 2 out]
        n161 = for {
          tunnel: w311 -> [w317]
          tunnel: w302 -> [w316] mode=indexing
          tunnel: w301 -> [w315]
          tunnel: w296 -> [w314] mode=indexing
          n162 = call "AlliGator Update Settings & Control.vi"("Error In"=w317, "Value"=w316, "Sender"=w315, "CtlRef"=w314) -> ()  [unwired: 7 in, 1 out]
        }
      }
      frame "Update SEPL Plot" {
        n163 = Enqueue Element(queue=w319, element=T80[] [{"AlliGator Q Event"=enum."Phasor Graph:Update SEPL Plot", "Data"=variant}]) -> ()  [unwired: 2 in, 3 out]
      }
      frame "Use Cursor (Extrapolate) Checkbox" {
        n164 = disable-structure shown="Enabled" {
          disable-tunnel: w322 -> [w328 _]
          frame Disabled {
            n165 = call-poly "Variant to Data.vi"("Variant"=w328) -> ("Value"=w326:bool)  [unwired: 8 in]
            n166 = property on="Use Periodicity" class="Bool (strict)"() -> ("Value"=w325:bool)  [unwired: 2 in, 2 out]
            n167 = Not(x=w326) -> (.not. x?=w327:bool)
            n168 = case shown="True" w326 {
              tunnel: w325 -> [w330 w332]
              tunnel: [w330 _] -> w324
              tunnel: [w329 w331] -> w323
              frame False {
                # "No Cursor: show Head Fraction/Add'l Points if Use Periodicity"
                n169 = Not(x=w330) -> (.not. x?=w329:bool)
              }
              frame True {
                # "Use Cursor: don't show Head Fraction/Add'l Points"
                n170 = Not(x=w332) -> (.not. x?=w331:bool)
              }
            }
            n171 = property on="Head Fraction" class="DigNum (strict)"("Visible"=w324) -> ()  [unwired: 2 in, 2 out]
            n172 = property on="Additional Points" class="DigNum (strict)"("Visible"=w323) -> ()  [unwired: 2 in, 2 out]
            n173 = property on="Tail Fraction" class="DigNum (strict)"("Visible"=w327) -> ()  [unwired: 2 in, 2 out]
          }
          frame Enabled {
          }
        }
      }
      frame "Use File Timestamp Checkbox" {
        # "deprecated"
      }
      frame "Use Fixed ROI Diameter Checkbox" {
        n174 = Enqueue Element(queue=w335, element=T80[] [{"AlliGator Q Event"=enum."Image:Set ROI Diameter", "Data"=variant}]) -> ()  [unwired: 2 in, 3 out]
      }
      frame "Use Periodicity (Extrapolate) Checkbox" {
        n175 = disable-structure shown="Disabled" {
          disable-tunnel: w338 -> [w343 _]
          frame Disabled {
            n176 = call-poly "Variant to Data.vi"("Variant"=w343) -> ("Value"=w340:bool)  [unwired: 8 in]
            n177 = property on="Use Cursors" class="Bool (strict)"() -> ("Value"=w341:bool)  [unwired: 2 in, 2 out]
            n178 = Not(x=w340) -> (.not. x?=w342:bool)
            n179 = case shown="False" w341 {
              tunnel: w340 -> [w344 _]
              tunnel: [w344 _] -> w339
              frame False {
              }
              frame True {
              }
            }
            n180 = property on="Additional Points" class="DigNum (strict)"("Visible"=w342) -> ()  [unwired: 2 in, 2 out]
            n181 = property on="Head Fraction" class="DigNum (strict)"("Visible"=w339) -> ()  [unwired: 2 in, 2 out]
          }
          frame Enabled {
          }
        }
      }
    }
  }
  n182 = case shown="\"Source Image\", Default" "Settings Tabs" {
    tunnel: "Fluorescence Decay Tabs" -> [_ _ w346 _ _ _ _ _ _ _ _ _]
    tunnel: "SEPL Tabs" -> [_ _ _ _ _ _ _ w348 _ _ _ _]
    tunnel: "Source Image Tabs" -> [w345 _ _ _ _ _ _ _ _ _ _ _]
    tunnel: "Phasor Plot Tabs" -> [_ _ _ _ _ w347 _ _ _ _ _ _]
    frame "Source Image", Default {
      n183 = case shown="\"Image Processing\"" w345 {
        frame "Pixel Processing", Default {
        }
        frame "Image Processing" {
        }
        frame "Image Cosmetics" {
        }
      }
    }
    frame "Data Information" {
    }
    frame "Fluorescence Decay" {
      n184 = case shown="\"Fit Parameters\"" w346 {
        frame "Decay Pre-Processing", Default {
        }
        frame "Advanced Analysis" {
        }
        frame "Fit Options" {
        }
        frame "Fit Parameters" {
        }
        frame "Styles" {
        }
      }
    }
    frame "Fluorescence Decay Statistics" {
    }
    frame "Intensity Time Trace" {
    }
    frame "Phasor Plot" {
      n185 = case shown="\"Phasor Plot Calculation\", Default" w347 {
        frame "Phasor Plot Calculation", Default {
        }
        frame "Phasor Plot Information Overlay" {
        }
        frame "Phasor Plot Appearance" {
        }
      }
    }
    frame "Phasor Graph" {
    }
    frame "Single-Exponential Phasor Locus (SEPL)" {
      n186 = case shown="\"IRF\"" w348 {
        frame "Display", Default {
        }
        frame "Phasor" {
        }
        frame "IRF" {
        }
        frame "Gates" {
        }
      }
    }
    frame "Phasor Calibration" {
    }
    frame "Lifetime Analysis" {
    }
    frame "Plugins" {
    }
    frame "Miscellaneous" {
    }
  }
  n187 = while {
    tunnel: w15 -> [w357]
    tunnel: w33 -> [w358]
    tunnel: w20 -> [w356]
    tunnel: w14 -> [w352]
    shift-right: [w354] -> _
    shift-left: w25 -> [w355]
    tunnel: w18 -> [w353]
    tunnel: refnum<vi> refnum ("event source") -> [w349]
    stop <- w359 stop-if-true
    n188 = event shown="[16] \"Gate Width\", \"Nanotime Gate Separation\", \"Gate Step\", \"Background Definition Range\", \"Gates to Skip\", \"Reject Low Decay Peak Pixels\", \"Min Peak Value\", \"Time Step\", \"Phasor Plot Size\", \"Phasor Plot Graphics Options\", \"Use Phasor Brightness\", \"Calibration Lifetime\", \"Verbose Mode\", \"Saved Displayed Image File Format\", \"Phasor Ratio Decay Range\", \"Phasor Ratio Reference Colors\", \"Exponential Fading\", \"Include Loading in Timing\", \"1-Normalize Decay\", \"Smoothing Parameter\", \"Beep after Script\", \"Use Backup Calibration if needed\", \"Backup Calibration Type\", \"Reject High Decay Peak Pixels\", \"Max Peak Value\", \"Use Intensity Correction File\", \"Phasor Ratio Type\", \"Fit Options\", \"Pixel-level Phasor Computation\", \"Show Last Decay Only\", \"Decay Graph Color Array\", \"Save Phasor Graph Image\", \"Export Tabulated Results\", \"Peak Threshold\", \"IRF Optimization Options\", \"Wavelet Analysis Options\", \"Tail Fraction\", \"Additional Points\", \"Verbose Settings Mode\", \"Extract IRF instead of Decay\", \"High Count Pixels Rejection Options\", \"Reverse Gates\", \"Laser Period\", \"Pixel Well Capacity\", \"Low Count Pixels Rejection Options\", \"Use Image Brightness\", \"Phasor Plot Smoothing Options\", \"Use Image Histogram for Contrast\", \"ROI Diameter\", \"ROI Center Color\", \"Verbose Error Mode\", \"Straighten Decay\", \"Verbose Decay Pre-Processing\", \"Square Pulse Options\", \"# Gates\", \"Exported Gate Image Settings\", \"Constant Background\", \"Pixel-Normalize Decay\", \"Phasor Ratio Display Range\", \"IRF Extraction Options\", \"Phasor Graph Frequency\", \"SYNC Period\", \"Pile-up Correction\", \"Head Fraction\", \"Invert Binary Mask\", \"Use Decay Pre-Processing\", \"Intensity Threshold\", \"Reference Radius\", \"Gates to Keep\", \"Selected Image ROI(s)\", \"All Image ROIs\", \"All Phasor Plot ROIs\", \"Selected Phasor Plot ROI(s)\", \"Calibration Type\", \"Fold Decay\", \"# Folds\", \"Histogram Options\", \"# Logical Processors Used\", \"Channel Name\", \"Channel Arithmetic\", \"Background File Subtraction\", \"Background Scaling Factor\", \"Background Pile-up Correction\", \"Background Pixel Well Capacity\", \"Define Shortest Lifetime as\", \"Python Settings\", \"Beep on Error\", \"Hot Pixel Removal\", \"Average Lifetime Options\", \"[0-1]-Normalize Decay\", \"Calibration Map Algorithm\", \"Gate Image Exposure\", \"Gate Image Integration\", \"Use Legacy Fitting Approach\", \"ROI Description Max Characters\", \"Available Channel Names\", \"Guess Parameters Options\", \"Transparent Mask Color\", \"Use Data Information Laser Period\", \"Phasor SDV Options\", \"Save Source Image\", \"Draw Reference Segment\", \"Dataset Scaling Factor\", \"Blend Overlay with Image Background\", \"Blend Overlay with Phasor Background\", \"Overlay Analyzed ROI Center\", \"User-Defined Quantity\", \"Scale Bar Options\", \"Image Resolution (Pixel Size)\", \"MLE Baseline Offset Type\", \"MLE Baseline Offset\", \"Dead Left Columns Correction\", \"Overlay ROI Median\", \"Median Overlay Color\", \"Optimal Offset Selection Criterion\", \"Intensity-weighted Phasor Plot\", \"Intensity-weighted Phasor Graph\": Value Change" {
      selector: w358 -> [_ _ _ _ _ _ _ _ _ _ _ _ _ _ _ _ _ _ _ _ _ _ _ _ _ _ _ _ _ _ _ _ _ _ _ _ _ _ _ _ _ _ _ _ _ _ _ _ _ w1006 w1062 _ w1073 w1078 _]
      dyn-events: [_ _ _ _ _ _ _ _ _ _ _ _ _ _ _ _ _ _ _ _ _ _ _ _ _ _ _ _ _ _ _ _ _ _ _ _ _ _ _ _ _ _ _ _ _ _ _ _ _ _ w1061 _ w1072 _ _] -> _
      timeout: 1000 -> [_ _ _ _ _ _ _ _ _ _ _ _ _ _ _ _ _ _ _ _ _ _ _ _ _ _ _ _ _ _ _ _ _ _ _ _ _ _ _ _ _ _ _ _ _ _ _ _ _ _ _ _ _ _ _]
      tunnel: [_ _ _ _ _ _ _ _ _ _ _ _ _ _ _ _ _ _ _ _ _ _ _ _ _ _ _ _ _ _ _ _ _ _ _ _ _ _ _ _ _ _ _ _ _ _ _ _ _ w1009 _ _ _ w1074 _] -> w359
      tunnel: w357 -> [_ _ _ _ _ _ _ _ _ _ _ _ _ _ _ _ w507 _ _ _ _ _ _ _ _ _ _ _ _ _ _ _ _ _ _ _ _ w896 _ _ _ _ _ _ _ _ _ _ _ w1012 _ _ _ _ _]
      tunnel: w356 -> [w365 w374 w383 w393 _ _ w411 _ w425 w437 w445 _ w480 _ w498 _ w506 _ w715 w730 _ w747 w757 _ _ _ _ w805 _ _ _ _ w861 _ _ _ _ _ _ w935 w943 _ _ _ w967 w975 w983 w992 _ w1010 _ _ _ _ _]
      tunnel: w355 -> [w367 w375 w382 w392 w396 w400 w412 w418 w429 w436 w446 w468 w479 w484 w499 w501 w516 w709 w724 w729 w740 w751 w756 w767 w775 w795 w798 w804 w809 w833 w846 w849 w860 w867 w876 w887 w893 w898 w923 w934 w942 w946 w953 w959 w966 w974 w981 w991 w995 w1008 _ w1068 _ w1077 w1081]
      tunnel: [w367 w375 w382 w392 w396 w400 w412 w418 w429 w436 w446 w468 w479 w484 w499 w501 w516 w709 w724 w729 w740 w751 w756 w767 w775 w795 w798 w804 w809 w833 w846 w849 w860 w867 w876 w887 w893 w898 w923 w934 w942 w946 w953 w959 w966 w974 w981 w991 w995 w1008 w1058 w1068 w1071 w1077 w1081] -> w354
      tunnel: w353 -> [_ w371 w381 w391 w395 _ _ _ _ w435 _ w449 w478 _ _ _ w513 _ _ _ _ _ _ w766 _ _ _ w803 _ w832 _ _ w859 _ _ _ w891 _ _ w933 w941 _ _ w958 w965 w973 w980 w990 _ w1007 _ _ _ w1076 w1079]
      tunnel: w352 -> [_ _ _ _ _ _ _ _ _ _ _ _ _ _ _ _ _ _ _ _ _ _ _ _ _ _ _ _ _ _ _ _ _ _ _ _ _ _ _ _ _ _ _ _ _ _ _ _ _ w1005 _ _ _ _ _]
      tunnel: [w366 w368 w376 w385 _ w397 w410 w415 w424 w432 w444 w447 w474 _ w497 _ w509 _ w712 w725 w737 w746 w752 w764 w771 _ _ w799 w807 w830 w841 _ w856 _ _ w877 _ w894 w922 w929 w937 _ _ _ w962 w969 w977 w987 _ w1005 _ w1063 _ _ _] -> w351
      tunnel: w349 -> [_ _ _ _ _ _ _ _ _ _ _ _ _ _ _ _ _ _ _ _ _ _ _ _ _ _ _ _ _ _ _ _ _ _ _ _ _ _ _ _ _ _ _ _ _ _ _ _ _ _ _ _ _ _ _]
      event "Background File", "Intensity Correction File": Value Change {
        # "Fixes a LabVIEW bug in 2021 SP1"
        n189 = event-data() -> ("CtlRef"=w362:refnum<vi>, "NewVal"=w364:path)  [unwired: 1 in]
        n190 = property class="Path"(reference=w362, "Value"=w364) -> (reference out=w361:refnum<vi>, error out=w363:errorcluster, "Label.Text"=w360:string)  [unwired: 1 in]
        n191 = call "AlliGator Update Settings & Control.vi"("Control Label"=w360, "Error In"=w363, "Value"=w364, "Sender"=w365, "CtlRef"=w361) -> ("Error Out"=w366:errorcluster)  [unwired: 6 in]
      }
      event "Background Subtraction": Value Change {
        n192 = event-data() -> ("CtlRef"=w373:refnum<vi>, "NewVal"=w372:bool)  [unwired: 1 in]
        n193 = call "AlliGator Update Settings & Control.vi"("Value"=w372, "Sender"=w374, "CtlRef"=w373) -> ("Error Out"=w370:errorcluster)  [unwired: 8 in]
        n194 = Enqueue Element(queue=w371, element=T77 {"Action"=enum."Baseline Subtraction Method", "Data"=variant}, error in (no error)=w370) -> (error out=w368:errorcluster)  [unwired: 1 in, 2 out]
      }
      event Value Change {
        n195 = event-data() -> ("CtlRef"=w384:refnum<vi>, "NewVal"=w377:T16)  [unwired: 1 in]
        n196 = call "AlliGator Update Settings & Control.vi"("Value"=w377, "Sender"=w383, "CtlRef"=w384) -> ("Error Out"=w380:errorcluster)  [unwired: 8 in]
        n197 = Bundle By Name(cluster=T77 {"Action"=enum."Baseline Subtraction Method", "Data"=variant} ("element"), "Data"=w377) -> (w378:T77)
        n198 = Enqueue Element(queue=w381, element=w378, error in (no error)=w380) -> (error out=w376:errorcluster)  [unwired: 1 in, 2 out]
      }
      event "Cumulative Phasor Plot": Value Change {
        n199 = event-data() -> ("CtlRef"=w389:refnum<vi>, "NewVal"=w386:bool)  [unwired: 1 in]
        n200 = call "AlliGator Update Settings & Control.vi"("Value"=w386, "Sender"=w393, "CtlRef"=w389) -> ("Error Out"=w390:errorcluster)  [unwired: 8 in]
        n201 = Bundle By Name(cluster=T77 {"Action"=enum."Cumulative Phasor Plot Checkbox", "Data"=variant} ("element"), "Data"=w386) -> (w387:T77)
        n202 = Enqueue Element(queue=w391, element=w387, error in (no error)=w390) -> (error out=w385:errorcluster)  [unwired: 1 in, 2 out]
      }
      event "Match Laser Period": Value Change {
        n203 = event-data() -> ()  [unwired: 1 in, 1 out]
        n204 = Enqueue Element(queue=w395, element=T77 {"Action"=enum."Update SEPL Parameters", "Data"=variant}) -> ()  [unwired: 2 in, 3 out]
      }
      event Shortcut Menu Selection (User) {
        n205 = event-data() -> ("ItemTag"=w399:string, "CtlRef"=w398:refnum<vi>)  [unwired: 1 in]
        n206 = case shown="\"Use Dataset Period\"" w399 {
          tunnel: w398 -> [_ w401]
          tunnel: [_ w402] -> w397
          frame "", Default {
          }
          frame "Use Dataset Period" {
            n207 = control-ref of="Laser Period"() -> (w406:refnum<vi>)
            n208 = To More Specific Class(target class=w406, reference=w401) -> (specific class reference=w407:refnum<vi>, error out=w405:errorcluster)  [unwired: 1 in]
            n209 = property class="DigNum (strict)"(reference=w406, error in=w405) -> (error out=w403:errorcluster, "Value"=w404:dbl[unit])  [unwired: 1 out]
            n210 = property class="DigNum (strict)"(reference=w407, error in=w403, "Val(Sgnl)"=w404) -> (error out=w402:errorcluster)  [unwired: 1 out]
          }
        }
      }
      event Value Change {
        n211 = event-data() -> ("CtlRef"=w414:refnum<vi>, "NewVal"=w408:T18)  [unwired: 1 in]
        n212 = call "AlliGator Update Settings Decay Shift Parameters Visibility.vi"("Shift Parameters Refnum"=w414) -> ("error out"=w409:errorcluster, "Shift Parameters Refnum"=w413:refnum<vi>)  [unwired: 9 in]
        n213 = call "AlliGator Update Settings & Control.vi"("Error In"=w409, "Value"=w408, "Sender"=w411, "CtlRef"=w413) -> ("Error Out"=w410:errorcluster)  [unwired: 7 in]
      }
      event "Decay Pre-Processing Operations Order": Shortcut Menu Selection (User) {
        n214 = event-data() -> ("CtlRef"=w417:refnum<vi>, "ItemTag"=w416:string)  [unwired: 1 in]
        n215 = case shown="\"Reorder Operations\"" w416 {
          tunnel: w417 -> [_ w420 w422]
          tunnel: [_ w419 w421] -> w415
          frame "", Default {
          }
          frame "Reorder Operations" {
            n216 = call "AlliGator Reorder Decay Pre-processing Operations.vi"("Ring in"=w420) -> ("Error Out"=w419:errorcluster)  [unwired: 10 in]
          }
          frame "Export JSON String to Clipboard" {
            n217 = call "AlliGator Export Settings Parameter JSON String to Clipboard.vi"("Control Refnum"=w422) -> ("Error Out"=w421:errorcluster)  [unwired: 9 in, 1 out]
          }
        }
      }
      event "Decay Pre-Processing Operations Order": Value Change {
        n218 = event-data() -> ("CtlRef"=w428:refnum<vi>)  [unwired: 1 in]
        n219 = property class="Ring (strict)"(reference=w428) -> (reference out=w426:refnum<vi>, error out=w423:errorcluster, "Strings []"=w427:string[])  [unwired: 1 in]
        n220 = call "AlliGator Update Settings & Control.vi"("Error In"=w423, "Value"=w427, "Sender"=w425, "CtlRef"=w426) -> ("Error Out"=w424:errorcluster)  [unwired: 7 in]
      }
      event Value Change {
        n221 = event-data() -> ("CtlRef"=w438:refnum<vi>, "NewVal"=w430:T13)  [unwired: 1 in]
        n222 = call "AlliGator Update Settings & Control.vi"("Value"=w430, "Sender"=w437, "CtlRef"=w438) -> ("Error Out"=w433:errorcluster)  [unwired: 8 in]
        n223 = Bundle By Name(cluster=T77 {"Action"=enum."Define Gates to Use", "Data"=variant} ("element"), "Data"=w430) -> (w431:T77)
        n224 = Enqueue Element(queue=w435, element=w431, error in (no error)=w433) -> (error out=w432:errorcluster)  [unwired: 1 in, 2 out]
      }
      event "Displayed Fit Parameters": Value Change {
        n225 = event-data() -> ("CtlRef"=w443:refnum<vi>, "NewVal"=w442:T42[])  [unwired: 1 in]
        n226 = call "Remove Duplicates From 1D Array.vim"("array"=w442) -> ("array with duplicates removed"=w439:T42[])  [unwired: 10 in]
        n227 = property class="Arr (strict)"(reference=w443, "Value"=w439) -> (reference out=w441:refnum<vi>, error out=w440:errorcluster)  [unwired: 1 in]
        n228 = call "AlliGator Update Settings & Control.vi"("Error In"=w440, "Value"=w439, "Sender"=w445, "CtlRef"=w441) -> ("Error Out"=w444:errorcluster)  [unwired: 7 in]
      }
      event "Edit User-defined Function": Value Change {
        n229 = event-data() -> ("CtlRef"=w465:refnum<vi>)  [unwired: 1 in]
        n230 = property class="Bool"(reference=w465) -> (error out=w463:errorcluster, "BoolText.Text"=w458:string)  [unwired: 1 in, 1 out]
        n231 = Equal?(x="Gate", y=w458) -> (x = y?=w456:bool)
        n232 = Select(t=AlliGator_Settings_List."Single-Exponential Phasor Locus (SEPL):User-defined Gate" ("AlliGator Settings List"), s=w456, f=AlliGator_Settings_List."Single-Exponential Phasor Locus (SEPL):User-defined IRF" ("AlliGator Settings List")) -> (s? t:f=w451:T73)
        n233 = call "AlliGator Settings Storage.vi"("AlliGator Settings List"=w451, "Error In"=w463) -> ("Error Out"=w462:errorcluster, "Variant Data out"=w461:variant)  [unwired: 8 in]
        n234 = Variant To Data(error in=w462, Variant=w461) -> (data=w459:T88, error out=w460:errorcluster)  [unwired: 1 in]
        n235 = Format Into String(format string="User-defined %s Plot" ("Original Graph Name"), error in=w460, w458) -> (resulting string=w467:string, error out=w464:errorcluster)  [unwired: 1 in]
        n236 = call "Plot Editor.vi"("Original Graph Name"=w467, "Error In"=w464, "Plot in"=w459) -> ("Error Out"=w453:errorcluster, "Plot out"=w452:T88)  [unwired: 6 in, 1 out]
        n237 = call "AlliGator Settings Storage.vi"("Get(F)/Set"=TRUE, "AlliGator Settings List"=w451, "Error In"=w453, "Variant Data in"=w452) -> ("Error Out"=w448:errorcluster)  [unwired: 6 in, 1 out]
        n238 = disable-structure shown="Disabled" {
          disable-tunnel: w449 -> [w471 _]
          disable-tunnel: w448 -> [w470 w473]
          disable-tunnel: [w469 w473] -> w447
          frame Disabled {
            n239 = Enqueue Element(queue=w471, element=T77 {"Action"=enum."Update SEPL Plot", "Data"=variant}, error in (no error)=w470) -> (error out=w469:errorcluster)  [unwired: 1 in, 2 out]
          }
          frame Enabled {
          }
        }
      }
      event "Extrapolate Decay": Value Change {
        n240 = event-data() -> ("CtlRef"=w481:refnum<vi>, "NewVal"=w477:bool)  [unwired: 1 in]
        n241 = call "AlliGator Update Settings & Control.vi"("Value"=w477, "Sender"=w480, "CtlRef"=w481) -> ("Error Out"=w476:errorcluster)  [unwired: 8 in]
        n242 = Enqueue Element(queue=w478, element=T77 {"Action"=enum."Extrapolate Decay Checkbox", "Data"=variant}, error in (no error)=w476) -> (error out=w474:errorcluster)  [unwired: 1 in, 2 out]
      }
      event Shortcut Menu Selection (User) {
        n243 = event-data() -> ("CtlRef"=w482:refnum<vi>, "ItemTag"=w483:string)  [unwired: 1 in]
        n244 = case shown="\"Export JSON String to Clipboard\"" w483 {
          tunnel: w482 -> [_ w485 w487]
          frame "", Default {
          }
          frame "Use Data Information >> Laser Period" {
            n245 = property on="Laser Period" class="DigNum (strict)"() -> ("Value"=w486:dbl[unit])  [unwired: 2 in, 2 out]
            n246 = property class="DigNum (strict)"(reference=w485, "Val(Sgnl)"=w486) -> ()  [unwired: 1 in, 2 out]
          }
          frame "Export JSON String to Clipboard" {
            n247 = call "AlliGator Export Settings Parameter JSON String to Clipboard.vi"("Control Refnum"=w487) -> ()  [unwired: 9 in, 2 out]
          }
        }
      }
      event "Fit Parameter Constraints": Value Change {
        n248 = event-data() -> ("CtlRef"=w496:refnum<vi>, "OldVal"=w495:T41[], "NewVal"=w494:T41[])  [unwired: 1 in]
        n249 = call "AlliGator Remove Duplicated Fit Parameter Constraints.vi"("New Constraints in"=w494, "Old Constraints"=w495) -> ("Error Out"=w489:errorcluster, "Offset Fitted?"=w490:bool, "New Constraints out"=w492:T41[])  [unwired: 7 in]
        n250 = property on="Optimal Offset Selection Criterion" class="Enum (strict)"(error in=w489, "Visible"=w490) -> (error out=w488:errorcluster)  [unwired: 1 in, 1 out]
        n251 = property class="Arr (strict)"(reference=w496, error in=w488, "Value"=w492) -> (reference out=w493:refnum<vi>, error out=w491:errorcluster)
        n252 = call "AlliGator Update Settings & Control.vi"("Error In"=w491, "Value"=w492, "Sender"=w498, "CtlRef"=w493) -> ("Error Out"=w497:errorcluster)  [unwired: 7 in]
      }
      event "Fluorescence Decay Tabs": Value Change {
        n253 = event-data() -> ("NewVal"=w500:T15)  [unwired: 1 in]
        n254 = case shown="\"Decay Pre-Processing\"" w500 {
          frame "Decay Pre-Processing" {
            n255 = call "AlliGator Settings Storage.vi"("AlliGator Settings List"=AlliGator_Settings_List."Fluorescence Decay_Decay Pre-Processing:Decay Pre-Processing Operations Order") -> ("Error Out"=w502:errorcluster, "Variant Data out"=w504:variant)  [unwired: 9 in]
            n256 = call-poly "Variant to Data.vi"("Variant"=w504) -> ("String Array"=w503:string[])  [unwired: 8 in]
            n257 = property on="Decay Pre-Processing Operations Order" class="Ring (strict)"(error in=w502, "Strings []"=w503) -> ()  [unwired: 1 in, 2 out]
          }
          frame "Advanced Analysis", Default {
          }
        }
      }
      event "Gate Width", "Nanotime Gate Separation", "Gate Step", "Background Definition Range", "Reject Low Decay Peak Pixels", "Min Peak Value", "Time Step", "Use Phasor Brightness", "Calibration Lifetime", "Verbose Mode", "Phasor Ratio Decay Range", "Phasor Ratio Reference Colors", "Exponential Fading", "Include Loading in Timing", "1-Normalize Decay", "Smoothing Parameter", "Beep after Script", "Use Backup Calibration if needed", "Backup Calibration Type", "Reject High Decay Peak Pixels", "Max Peak Value", "Use Intensity Correction File", "Pixel-level Phasor Computation", "Show Last Decay Only", "Decay Graph Color Array", "Save Phasor Graph Image", "Export Tabulated Results", "Peak Threshold", "Tail Fraction", "Additional Points", "Verbose Settings Mode", "Extract IRF instead of Decay", "Reverse Gates", "Laser Period", "Pixel Well Capacity", "Use Image Brightness", "Use Image Histogram for Contrast", "ROI Diameter", "ROI Center Color", "Verbose Error Mode", "Straighten Decay", "Verbose Decay Pre-Processing", "# Gates", "Constant Background", "Pixel-Normalize Decay", "Phasor Ratio Display Range", "Phasor Graph Frequency", "SYNC Period", "Pile-up Correction", "Head Fraction", "Invert Binary Mask", "Use Decay Pre-Processing", "Intensity Threshold", "Reference Radius", "Selected Image ROI(s)", "All Image ROIs", "All Phasor Plot ROIs", "Selected Phasor Plot ROI(s)", "Fold Decay", "# Folds", "# Logical Processors Used", "Channel Name", "Background File Subtraction", "Background Scaling Factor", "Background Pile-up Correction", "Background Pixel Well Capacity", "Beep on Error", "[0-1]-Normalize Decay", "Gate Image Exposure", "Gate Image Integration", "Use Legacy Fitting Approach", "ROI Description Max Characters", "Available Channel Names", "Transparent Mask Color", "Use Data Information Laser Period", "Save Source Image", "Draw Reference Segment", "Dataset Scaling Factor", "Blend Overlay with Image Background", "Blend Overlay with Phasor Background", "Overlay Analyzed ROI Center", "User-Defined Quantity", "Image Resolution (Pixel Size)", "MLE Baseline Offset", "Dead Left Columns Correction", "Overlay ROI Median", "Median Overlay Color", "Intensity-weighted Phasor Plot", "Intensity-weighted Phasor Graph": Value Change {
        n258 = event-data() -> ("CtlRef"=w515:refnum<vi>, "NewVal"=w512:variant)  [unwired: 1 in]
        n259 = call "AlliGator Update Settings & Control.vi"("Value"=w512, "Sender"=w506, "CtlRef"=w515) -> ("Error Out"=w510:errorcluster)  [unwired: 8 in]
        n260 = property class="Ctl"(reference=w515, error in=w510) -> (reference out=w508:refnum<vi>, error out=w511:errorcluster, "Label.Text"=w514:string)
        n261 = case shown="\"Fit Options\", \"Use Data Information Laser Period\"" w514 {
          selector: w514 -> [_ _ _ _ _ _ _ _ _ _ w594 _ _ _ _ _ _ _ _ _ _ _ _]
          tunnel: w513 -> [_ w521 _ _ _ _ _ _ _ w593 w598 _ w610 w620 w634 _ _ w652 _ _ _ _ _]
          tunnel: w512 -> [_ _ w526 w530 w543 w551 _ w577 _ w588 _ w601 w607 _ w632 w639 w645 w651 w666 _ w682 w690 w702]
          tunnel: w511 -> [w517 w519 w522 w529 w541 w549 w560 w572 w579 w592 _ w602 w609 w619 w631 w637 w643 w650 w665 w677 w680 w688 w701]
          tunnel: [w517 w518 w523 w528 w540 w548 w559 w573 w578 w591 w597 w599 w608 w618 w630 w636 w642 w649 w664 w678 w679 w687 w695] -> w509
          tunnel: w506 -> [_ _ _ _ _ _ _ _ _ _ _ _ _ _ w625 w640 w646 w648 _ _ _ _ _]
          tunnel: w508 -> [_ _ _ _ _ _ _ _ _ _ _ _ _ _ _ _ _ _ _ w676 _ _ _]
          tunnel: w507 -> [_ _ _ _ _ _ _ _ _ _ _ _ _ _ _ _ _ _ _ _ _ _ _]
          frame "", Default {
          }
          frame "# Gates", "Additional Points", "Decay Shift Parameters", "Extrapolate Decay", "Gate Separation", "Gate Step", "Gates to Skip", "Shift Decay", "Use Decay Pre-Processing" {
            n262 = Enqueue Element(queue=w521, element=T77 {"Action"=enum."Update Natural Frequency", "Data"=variant}, error in (no error)=w519) -> (error out=w518:errorcluster)  [unwired: 1 in, 2 out]
          }
          frame "# Logical Processors Used" {
            n263 = call-poly "Variant to Data.vi"("Variant"=w526) -> ("Value"=w524:i32)  [unwired: 8 in]
            n264 = call "Logical Processors Used.vi"("Set/Get (F)"=TRUE, "# Logical Processor Used"=w524) -> ()  [unwired: 4 in, 1 out]
            n265 = call "IMAQ Multi-Core Options"("Get/Set Number of Cores (Get)"=enum32{"Get", "Set", "Set Max Available"}."Set", "error in (no error)"=w522, "Specified Number of Cores"=w524) -> ("error out"=w523:errorcluster)  [unwired: 7 in, 1 out]
          }
          frame "1-Normalize Decay" {
            n266 = disable-structure shown="Disabled" {
              disable-tunnel: w530 -> [w534 _]
              disable-tunnel: w529 -> [w532 _]
              disable-tunnel: [w531 _] -> w528
              frame Disabled {
                n267 = call-poly "Variant to Data.vi"("Variant"=w534) -> ("Value"=w533:bool)  [unwired: 8 in]
                n268 = case shown="True" w533 {
                  selector: w533 -> [_ w539]
                  tunnel: w532 -> [w535 w537]
                  tunnel: [w535 w536] -> w531
                  frame False {
                  }
                  frame True {
                    n269 = Not(x=w539) -> (.not. x?=w538:bool)
                    n270 = property on="Pixel-Normalize Decay" class="Bool (strict)"(error in=w537, "Val(Sgnl)"=w538) -> (error out=w536:errorcluster)  [unwired: 1 in, 1 out]
                  }
                }
              }
              frame Enabled {
              }
            }
          }
          frame "All Image ROIs" {
            n271 = call-poly "Variant to Data.vi"("Variant"=w543) -> ("Value"=w542:bool)  [unwired: 8 in]
            n272 = case shown="False" w542 {
              tunnel: w541 -> [w544 w546]
              tunnel: [w544 w545] -> w540
              frame False {
              }
              frame True {
                n273 = property on="Selected Image ROI(s)" class="Bool (strict)"(error in=w546, "Val(Sgnl)"=FALSE ("Value (Signaling)")) -> (error out=w545:errorcluster)  [unwired: 1 in, 1 out]
              }
            }
          }
          frame "All Phasor Plot ROIs" {
            n274 = call-poly "Variant to Data.vi"("Variant"=w551) -> ("Value"=w550:bool)  [unwired: 8 in]
            n275 = case shown="True" w550 {
              tunnel: w549 -> [w552 w554]
              tunnel: [w552 w553] -> w548
              frame False {
              }
              frame True {
                n276 = property on="Selected Phasor Plot ROI(s)" class="Bool (strict)"(error in=w554, "Val(Sgnl)"=FALSE ("Value (Signaling)")) -> (error out=w553:errorcluster)  [unwired: 1 in, 1 out]
              }
            }
          }
          frame "Backup Calibration Type" {
            n277 = call "AlliGator Settings Storage.vi"("AlliGator Settings List"=AlliGator_Settings_List."Phasor Calibration:Use Backup Calibration if needed") -> ("Variant Data out"=w557:variant)  [unwired: 9 in, 1 out]
            n278 = call-poly "Variant to Data.vi"("Variant"=w557) -> ("Value"=w556:bool)  [unwired: 8 in]
            n279 = case shown="True" w556 {
              tunnel: w560 -> [w561 w563]
              tunnel: [w561 w562] -> w559
              frame False {
              }
              frame True {
                n280 = call "Alligator Variables Storage.vi"("AlliGator Variable"=AlliGator_Variables_List."Phasor Plot:Computed" ("Alligator Variable"), "Error In"=w563) -> ("Error Out"=w564:errorcluster, "Data out"=w566:variant)  [unwired: 7 in, 1 out]
                n281 = call-poly "Variant to Data.vi"("Variant"=w566) -> ("Value"=w565:bool)  [unwired: 8 in]
                n282 = case shown="True" w565 {
                  tunnel: w564 -> [w568 w571]
                  tunnel: [w568 w569] -> w562
                  frame False {
                  }
                  frame True {
                    n283 = call "AlliGator Set Phasor Plot Update LED.vi"("error in (no error)"=w571, "Off/On"=TRUE) -> ("error out"=w569:errorcluster)  [unwired: 9 in]
                  }
                }
              }
            }
          }
          frame "Beep on Error" {
            n284 = call-poly "Variant to Data.vi"("Variant"=w577) -> ("Value"=w576:bool)  [unwired: 8 in]
            n285 = call "Notebook Parameter Storage.vi"("Get(F)/Set"=TRUE, "Notebook Parameter List"=Notebook_Parameters_List."Beep on Error?", "Error In"=w572, "Data in"=w576) -> ("Error Out"=w573:errorcluster)  [unwired: 6 in, 1 out]
          }
          frame "Calibration Lifetime", "Calibration Map Algorithm", "Calibration Type", "Use Backup Calibration if needed" {
            n286 = call "Alligator Variables Storage.vi"("AlliGator Variable"=AlliGator_Variables_List."Phasor Plot:Computed" ("Alligator Variable"), "Error In"=w579) -> ("Error Out"=w580:errorcluster, "Data out"=w582:variant)  [unwired: 7 in, 1 out]
            n287 = call-poly "Variant to Data.vi"("Variant"=w582) -> ("Value"=w581:bool)  [unwired: 8 in]
            n288 = case shown="True" w581 {
              tunnel: w580 -> [w584 w587]
              tunnel: [w584 w585] -> w578
              frame False {
              }
              frame True {
                n289 = call "AlliGator Set Phasor Plot Update LED.vi"("error in (no error)"=w587, "Off/On"=TRUE) -> ("error out"=w585:errorcluster)  [unwired: 9 in]
              }
            }
          }
          frame "Channel Name" {
            n290 = Bundle By Name(cluster=T77 {"Action"=enum."Channel Name Changed", "Data"=variant} ("element"), "Data"=w588) -> (w589:T77)
            n291 = Enqueue Element(queue=w593, element=w589, error in (no error)=w592) -> (error out=w591:errorcluster)  [unwired: 1 in, 2 out]
          }
          frame "Fit Options", "Use Data Information Laser Period" {
            n292 = Bundle By Name(cluster=T77 {"Action"=enum."Fit Options Changed", "Data"=variant} ("element"), "Data"=w594) -> (w595:T77)
            n293 = Enqueue Element(queue=w598, element=w595) -> (error out=w597:errorcluster)  [unwired: 2 in, 2 out]
          }
          frame "Fold Decay" {
            n294 = call-poly "Variant to Data.vi"("Variant"=w601) -> ("Value"=w600:bool)  [unwired: 8 in]
            n295 = property on="# Folds" class="DigNum (strict)"(error in=w602, "Visible"=w600) -> (error out=w599:errorcluster)  [unwired: 1 in, 1 out]
          }
          frame "Hot Pixel Removal" {
            n296 = Variant To Data(type=T3 {"Remove Screamers"=TRUE, "Delta"=inf, "Equalize Histogram"=FALSE, "Percentile"=0.0, "Hot Pixel Mask Image"=path "", "Use Hot Pixel Mask"=TRUE} ("Hot Pixel Removal"), Variant=w607) -> (data=w605:T3)  [unwired: 1 in, 1 out]
            n297 = Unbundle By Name(w605) -> ("Use Hot Pixel Mask"=w603:bool, "Hot Pixel Mask Image"=w604:path)
            n298 = case shown="True" w603 {
              tunnel: w610 -> [_ w617]
              tunnel: w609 -> [w611 w616]
              tunnel: [w611 w615] -> w608
              tunnel: w604 -> [_ w613]
              frame False {
              }
              frame True {
                n299 = Bundle By Name(cluster=T77 {"Action"=enum."Load Hot Pixel Mask Image", "Data"=variant} ("element"), "Data"=w613) -> (w612:T77)
                n300 = Enqueue Element(queue=w617, element=w612, error in (no error)=w616) -> (error out=w615:errorcluster)  [unwired: 1 in, 2 out]
              }
            }
          }
          frame "IRF Order" {
            n301 = disable-structure shown="Disabled" {
              disable-tunnel: w620 -> [w623 _]
              disable-tunnel: w619 -> [w622 _]
              disable-tunnel: [w621 _] -> w618
              frame Disabled {
                # "hidden control: unused"
                n302 = Enqueue Element(queue=w623, element=T77 {"Action"=enum."Define IRF Time Constants", "Data"=variant}, error in (no error)=w622) -> (error out=w621:errorcluster)  [unwired: 1 in, 2 out]
              }
              frame Enabled {
              }
            }
          }
          frame "Phasor Graph Frequency" {
            n303 = Variant To Data(error in=w631, type=dbl[unit] 0.0 ("Phasor Frequency 2"), Variant=w632) -> (data=w629:dbl[unit], error out=w628:errorcluster)
            n304 = local write "Phasor Plot Frequency"(w629) -> ()
            n305 = control-ref of="Phasor Plot Frequency"() -> (w626:refnum<vi>)
            n306 = call "AlliGator Update Settings & Control.vi"("Error In"=w628, "Value"=w629, "Sender"=w625, "CtlRef"=w626) -> ("Error Out"=w627:errorcluster)  [unwired: 7 in]
            n307 = Enqueue Element(queue=w634, element=T77 {"Action"=enum."Update SEPL Plot", "Data"=variant}, error in (no error)=w627) -> (error out=w630:errorcluster)  [unwired: 1 in, 2 out]
          }
          frame "Intensity-weighted Phasor Graph" {
            n308 = call-poly "Variant to Data.vi"("Variant"=w639) -> ("Value"=w638:bool)  [unwired: 8 in]
            n309 = local write "Intensity-weighted Phasor Plot"(w638) -> ()
            n310 = control-ref of="Intensity-weighted Phasor Plot"() -> (w641:refnum<vi>)
            n311 = call "AlliGator Update Settings & Control.vi"("Error In"=w637, "Value"=w638, "Sender"=w640, "CtlRef"=w641) -> ("Error Out"=w636:errorcluster)  [unwired: 7 in]
          }
          frame "Intensity-weighted Phasor Plot" {
            n312 = call-poly "Variant to Data.vi"("Variant"=w645) -> ("Value"=w644:bool)  [unwired: 8 in]
            n313 = local write "Intensity-weighted Phasor Graph"(w644) -> ()
            n314 = control-ref of="Intensity-weighted Phasor Graph"() -> (w647:refnum<vi>)
            n315 = call "AlliGator Update Settings & Control.vi"("Error In"=w643, "Value"=w644, "Sender"=w646, "CtlRef"=w647) -> ("Error Out"=w642:errorcluster)  [unwired: 7 in]
          }
          frame "Phasor Plot Frequency" {
            n316 = disable-structure shown="Enabled" {
              disable-tunnel: w652 -> [w662 _]
              disable-tunnel: w651 -> [w660 _]
              disable-tunnel: w650 -> [w659 _]
              disable-tunnel: [w658 _] -> w649
              disable-tunnel: w648 -> [w655 _]
              frame Disabled {
                n317 = Variant To Data(error in=w659, type=dbl[unit] 0.0 ("Phasor Frequency 2"), Variant=w660) -> (data=w653:dbl[unit], error out=w657:errorcluster)
                n318 = local write "Phasor Graph Frequency"(w653) -> ()
                n319 = control-ref of="Phasor Graph Frequency"() -> (w656:refnum<vi>)
                n320 = call "AlliGator Update Settings & Control.vi"("Error In"=w657, "Value"=w653, "Sender"=w655, "CtlRef"=w656) -> ("Error Out"=w654:errorcluster)  [unwired: 7 in]
                n321 = Enqueue Element(queue=w662, element=T77 {"Action"=enum."Update SEPL Plot", "Data"=variant}, error in (no error)=w654) -> (error out=w658:errorcluster)  [unwired: 1 in, 2 out]
              }
              frame Enabled {
              }
            }
          }
          frame "Pixel-Normalize Decay" {
            n322 = disable-structure shown="Enabled" {
              disable-tunnel: w666 -> [w670 _]
              disable-tunnel: w665 -> [w668 _]
              disable-tunnel: [w667 _] -> w664
              frame Disabled {
                n323 = call-poly "Variant to Data.vi"("Variant"=w670) -> ("Value"=w669:bool)  [unwired: 8 in]
                n324 = case shown="True" w669 {
                  selector: w669 -> [_ w675]
                  tunnel: w668 -> [w671 w673]
                  tunnel: [w671 w672] -> w667
                  frame False {
                  }
                  frame True {
                    n325 = Not(x=w675) -> (.not. x?=w674:bool)
                    n326 = property on="1-Normalize Decay" class="Bool (strict)"(error in=w673, "Val(Sgnl)"=w674) -> (error out=w672:errorcluster)  [unwired: 1 in, 1 out]
                  }
                }
              }
              frame Enabled {
              }
            }
          }
          frame "Python Settings" {
            n327 = call "AlliGator Update Settings Python Options.vi"("error in (no error)"=w677, "Python Settings Refnum"=w676) -> ("error out"=w678:errorcluster)  [unwired: 9 in]
          }
          frame "Selected Image ROI(s)" {
            n328 = call-poly "Variant to Data.vi"("Variant"=w682) -> ("Value"=w681:bool)  [unwired: 8 in]
            n329 = case shown="True" w681 {
              tunnel: w680 -> [w683 w685]
              tunnel: [w683 w684] -> w679
              frame False {
              }
              frame True {
                n330 = property on="All Image ROIs" class="Bool (strict)"(error in=w685, "Val(Sgnl)"=FALSE ("Value (Signaling)")) -> (error out=w684:errorcluster)  [unwired: 1 in, 1 out]
              }
            }
          }
          frame "Selected Phasor Plot ROI(s)" {
            n331 = call-poly "Variant to Data.vi"("Variant"=w690) -> ("Value"=w689:bool)  [unwired: 8 in]
            n332 = case shown="True" w689 {
              tunnel: w688 -> [w691 w693]
              tunnel: [w691 w692] -> w687
              frame False {
              }
              frame True {
                n333 = property on="All Phasor Plot ROIs" class="Bool (strict)"(error in=w693, "Val(Sgnl)"=FALSE ("Value (Signaling)")) -> (error out=w692:errorcluster)  [unwired: 1 in, 1 out]
              }
            }
          }
          frame "MLE Baseline Offset Type" {
            n334 = Variant To Data(error in=w701, type=MLE_Baseline_Offset_Type."Absolute" ("MLE Baseline Offset Type"), Variant=w702) -> (data=w699:T37, error out=w696:errorcluster)
            n335 = case shown="\"Absolute\", Default" w699 {
              tunnel: [inf ("Data Entry Limits:Maximum") 100.0 ("Data Entry Limits:Maximum")] -> w698
              tunnel: [-inf ("Data Entry Limits:Minimum") 0.0 ("Data Entry Limits:Minimum")] -> w697
              frame "Absolute", Default {
              }
              frame "Percentage" {
              }
            }
            n336 = property on="MLE Baseline Offset" class="DigNum (strict)"(error in=w696, "Maximum"=w698, "Minimum"=w697) -> (error out=w695:errorcluster)  [unwired: 1 in, 1 out]
          }
        }
      }
      event "Extract IRF instead of Decay", "ROI Diameter", "Use Fixed ROI Diameter", "Verbose Mode", "Use Image Brightness", "Use Phasor Brightness", "ROI Center Color", "Use Image Histogram for Contrast", "Nanotime Gate Separation", "Gate Width", "Gate Step", "Background Subtraction", "Background Definition Range", "Reject Low Decay Peak Pixels", "Time Step", "Use File Timestamp", "Cumulative Phasor Plot", "Calibration Lifetime", "Min Peak Value", "Phasor Ratio Decay Range", "Phasor Ratio Reference Colors", "Exponential Fading", "Include Loading in Timing", "1-Normalize Decay", "Smoothing Parameter", "Smoothen Decay", "Shift Decay", "Use Backup Calibration if needed", "Backup Calibration Type", "Reject High Decay Peak Pixels", "Max Peak Value", "Use Intensity Correction File", "Intensity Correction File", "Show Last Decay Only", "Decay Graph Color Array", "Displayed Fit Parameters", "Fit Parameter Constraints", "Save Phasor Graph Image", "Export Tabulated Results", "Peak Threshold", "Extrapolate Decay", "Tail Fraction", "Additional Points", "Verbose Settings Mode", "Reverse Gates", "Laser Period", "Pile-up Correction", "Pixel Well Capacity", "Guess Parameter Values", "Use Guess Parameters", "Guess Parameter Names", "Verbose Error Mode", "Straighten Decay", "Phasor Ratio Color Map Type", "Restore Skipped Dialogs", "Verbose Decay Pre-Processing", "Fluorescence Decay Graph Default Plot Style", "Lifetime Analysis Graph Default Plot Style", "# Gates", "Ref 2 Label", "Ref 1 Label", "Constant Background", "Pixel-Normalize Decay", "Phasor Ratio Display Range", "Use Current Dataset Parameters", "Use Last Fitted Parameters", "Use Periodicity", "Use Cursors", "Head Fraction", "Invert Binary Mask", "Use Decay Pre-Processing", "Match Laser Period", "Intensity Threshold", "Reference Radius", "Selected Image ROI(s)", "All Image ROIs", "Selected Phasor Plot ROI(s)", "All Phasor Plot ROIs", "Fold Decay", "# Folds", "# Logical Processors", "# Logical Processors Used", "Channel Name", "Background Pixel Well Capacity", "Background Pile-up Correction", "Background File", "Background Scaling Factor", "Background File Subtraction", "Valid Python Session", "[0-1]-Normalize Decay", "Intensity-weighted Phasor Plot", "Intensity-weighted Phasor Graph": Shortcut Menu Selection (User) {
        n337 = event-data() -> ("CtlRef"=w708:refnum<vi>, "ItemTag"=w707:string)  [unwired: 1 in]
        n338 = case shown="\"Export JSON String to Clipboard\"" w707 {
          tunnel: w708 -> [_ w710]
          frame "", Default {
          }
          frame "Export JSON String to Clipboard" {
            n339 = call "AlliGator Export Settings Parameter JSON String to Clipboard.vi"("Control Refnum"=w710) -> ()  [unwired: 9 in, 2 out]
          }
        }
      }
      event "Guess Parameter Values", "Guess Parameter Names": Value Change {
        n340 = event-data() -> ("CtlRef"=w723:refnum<vi>, "OldVal"=w721:variant)  [unwired: 1 in]
        n341 = property class="Arr"(reference=w723) -> (error out=w720:errorcluster, "Label.Text"=w722:string)  [unwired: 1 in, 1 out]
        n342 = control-ref of="Guess Parameter Values"() -> (w719:refnum<vi>)
        n343 = control-ref of="Guess Parameter Names"() -> (w714:refnum<vi>)
        n344 = call "AlliGator Update Settings Guess Parameter Arrays.vi"("Modified Control"=w722, "Error In"=w720, "Old Value"=w721, "Guess Parameter Names"=w714, "Guess Parameters"=w719) -> ("Error Out"=w717:errorcluster, "Guess Parameter Name Array"=w716:T40[], "Guess Parameter Array"=w718:dbl[])  [unwired: 4 in]
        n345 = call "AlliGator Update Settings & Control.vi"("Error In"=w717, "Value"=w718, "Sender"=w715, "CtlRef"=w719) -> ("Error Out"=w713:errorcluster)  [unwired: 7 in]
        n346 = call "AlliGator Update Settings & Control.vi"("Error In"=w717, "Value"=w716, "Sender"=w715, "CtlRef"=w714) -> ("Error Out"=w711:errorcluster)  [unwired: 7 in]
        n347 = Merge Errors(w713, w711) -> (w712:errorcluster)
      }
      event Value Change {
        n348 = event-data() -> ("CtlRef"=w731:refnum<vi>, "NewVal"=w728:T9)  [unwired: 1 in]
        n349 = Unbundle By Name(w728) -> ("Use Image Binning"=w727:bool)
        n350 = call "AlliGator Update Settings & Control.vi"("Value"=w728, "Sender"=w730, "CtlRef"=w731) -> ("Error Out"=w726:errorcluster)  [unwired: 8 in]
        n351 = case shown="False" w727 {
          selector: w727 -> [_ w736]
          tunnel: w726 -> [w732 w734]
          tunnel: [w732 w733] -> w725
          frame False {
          }
          frame True {
            n352 = Not(x=w736) -> (.not. x?=w735:bool)
            n353 = property on="Use Image Smoothing" class="Bool (strict)"(error in=w734, "Val(Sgnl)"=w735) -> (error out=w733:errorcluster)  [unwired: 1 in, 1 out]
          }
        }
      }
      event "Image Pre-Processing Operations Order": Shortcut Menu Selection (User) {
        n354 = event-data() -> ("CtlRef"=w739:refnum<vi>, "ItemTag"=w738:string)  [unwired: 1 in]
        n355 = case shown="\"\", Default" w738 {
          tunnel: w739 -> [_ w742 w744]
          tunnel: [_ w741 w743] -> w737
          frame "", Default {
          }
          frame "Reorder Operations" {
            n356 = call "AlliGator Reorder Decay Pre-processing Operations.vi"("Ring in"=w742) -> ("Error Out"=w741:errorcluster)  [unwired: 10 in]
          }
          frame "Export JSON String to Clipboard" {
            n357 = call "AlliGator Export Settings Parameter JSON String to Clipboard.vi"("Control Refnum"=w744) -> ("Error Out"=w743:errorcluster)  [unwired: 9 in, 1 out]
          }
        }
      }
      event "Image Pre-Processing Operations Order": Value Change {
        n358 = event-data() -> ("CtlRef"=w750:refnum<vi>)  [unwired: 1 in]
        n359 = property class="Ring (strict)"(reference=w750) -> (reference out=w748:refnum<vi>, error out=w745:errorcluster, "Strings []"=w749:string[])  [unwired: 1 in]
        n360 = call "AlliGator Update Settings & Control.vi"("Error In"=w745, "Value"=w749, "Sender"=w747, "CtlRef"=w748) -> ("Error Out"=w746:errorcluster)  [unwired: 7 in]
      }
      event Value Change {
        n361 = event-data() -> ("CtlRef"=w758:refnum<vi>, "NewVal"=w755:T6)  [unwired: 1 in]
        n362 = Unbundle By Name(w755) -> ("Use Image Smoothing"=w754:bool)
        n363 = call "AlliGator Update Settings & Control.vi"("Value"=w755, "Sender"=w757, "CtlRef"=w758) -> ("Error Out"=w753:errorcluster)  [unwired: 8 in]
        n364 = case shown="False" w754 {
          selector: w754 -> [_ w763]
          tunnel: w753 -> [w759 w761]
          tunnel: [w759 w760] -> w752
          frame False {
          }
          frame True {
            n365 = Not(x=w763) -> (.not. x?=w762:bool)
            n366 = property on="Use Image Binning" class="Bool (strict)"(error in=w761, "Val(Sgnl)"=w762) -> (error out=w760:errorcluster)  [unwired: 1 in, 1 out]
          }
        }
      }
      event "Natural Frequency": Shortcut Menu Selection (User) {
        n367 = event-data() -> ()  [unwired: 1 in, 1 out]
        n368 = Enqueue Element(queue=w766, element=T77 {"Action"=enum."Update Natural Frequency", "Data"=variant}) -> (error out=w764:errorcluster)  [unwired: 2 in, 2 out]
      }
      event "Phasor Plot Frequency", "Phasor Graph Frequency": Shortcut Menu Selection (User) {
        n369 = event-data() -> ("CtlRef"=w770:refnum<vi>, "ItemTag"=w774:string)  [unwired: 1 in]
        n370 = case shown="\"Use Harmonic of Current Frequency (n > 1)\"" w774 {
          tunnel: [_ 1 ("Harmonic (1)") 1 ("Harmonic (1)") _ _ _ 1 ("Harmonic (1)") _] -> w773
          tunnel: [_ _ TRUE ("Use n/D") _ TRUE ("Use n/D") _ _ _] -> w772
          tunnel: w770 -> [_ _ _ _ _ _ _ w793]
          tunnel: [_ TRUE TRUE TRUE TRUE TRUE w791 _] -> w769
          tunnel: [_ _ _ _ _ TRUE ("Use n/D") w791 _] -> w768
          frame "", Default {
          }
          frame "f = 1/T" {
          }
          frame "f = 1/D" {
          }
          frame "f = n/T (n > 1)" {
          }
          frame "f = n/D (n > 1)" {
          }
          frame "Use Harmonic of Current Frequency (n > 1)" {
          }
          frame "Use Current Frequency" {
            w791 = TRUE
          }
          frame "Export JSON String to Clipboard" {
            n371 = call "AlliGator Export Settings Parameter JSON String to Clipboard.vi"("Control Refnum"=w793) -> ()  [unwired: 9 in, 2 out]
          }
        }
        n372 = case shown="True" w769 {
          tunnel: w773 -> [_ w780]
          tunnel: w772 -> [_ w779]
          tunnel: [_ w778] -> w771
          tunnel: w770 -> [_ w777]
          tunnel: w768 -> [_ w776]
          frame False {
          }
          frame True {
            n373 = call "AlliGator Set Phasor Harmonic.vi"("Use n/D"=w779, "Harmonic (1)"=w780, "Use Current Frequency"=w776, "Phasor Frequency Refnum"=w777) -> ("Error Out"=w778:errorcluster)  [unwired: 7 in]
          }
        }
      }
      event "Phasor Plot Frequency": Value Change {
        n374 = event-data() -> ("NewVal"=w794:dbl[unit])  [unwired: 1 in]
        n375 = property on="Phasor Graph Frequency" class="DigNum (strict)"("Val(Sgnl)"=w794) -> ()  [unwired: 2 in, 2 out]
      }
      event "Extract IRF instead of Decay", "ROI Diameter", "Use Fixed ROI Diameter", "Verbose Mode", "Use Image Brightness", "Use Phasor Brightness", "ROI Center Color", "Use Image Histogram for Contrast", "Nanotime Gate Separation", "Gate Width", "Gate Step", "Background Subtraction", "Background Definition Range", "Reject Low Decay Peak Pixels", "Time Step", "Use File Timestamp", "Cumulative Phasor Plot", "Calibration Lifetime", "Min Peak Value", "Phasor Ratio Decay Range", "Phasor Ratio Reference Colors", "Exponential Fading", "Include Loading in Timing", "1-Normalize Decay", "Smoothing Parameter", "Smoothen Decay", "Shift Decay", "Use Backup Calibration if needed", "Backup Calibration Type", "Reject High Decay Peak Pixels", "Max Peak Value", "Use Intensity Correction File", "Intensity Correction File", "Pixel-level Phasor Computation", "Show Last Decay Only", "Decay Graph Color Array", "Displayed Fit Parameters", "Fit Parameter Constraints", "Save Phasor Graph Image", "Export Tabulated Results", "Peak Threshold", "Extrapolate Decay", "Tail Fraction", "Additional Points", "Verbose Settings Mode", "Reverse Gates", "Laser Period", "Pile-up Correction", "Pixel Well Capacity", "Guess Parameter Values", "Use Guess Parameters", "Guess Parameter Names", "Verbose Error Mode", "Straighten Decay", "Phasor Ratio Color Map Type", "Decay Pre-Processing Operations Order", "Restore Skipped Dialogs", "Verbose Decay Pre-Processing", "Phasor Plot Frequency", "Fluorescence Decay Graph Default Plot Style", "Lifetime Analysis Graph Default Plot Style", "# Gates", "Ref 2 Label", "Ref 1 Label", "Constant Background", "Pixel-Normalize Decay", "Phasor Ratio Display Range", "Phasor Graph Frequency", "Use Current Dataset Parameters", "SYNC Period", "Use Last Fitted Parameters", "Use Periodicity", "Use Cursors", "Head Fraction", "Invert Binary Mask", "Use Decay Pre-Processing", "Match Laser Period", "Intensity Threshold", "Reference Radius", "Selected Image ROI(s)", "All Image ROIs", "All Phasor Plot ROIs", "Fold Decay", "# Folds", "# Logical Processors", "# Logical Processors Used", "Channel Name", "Background Pixel Well Capacity", "Background Pile-up Correction", "Background File", "Background Scaling Factor", "Background File Subtraction", "Available Channel Names", "[0-1]-Normalize Decay": Shortcut Menu Activation? {
        n376 = event-data() -> ("MenuRef"=w797:refnum<k9>)  [unwired: 1 in]
        n377 = Insert Menu Items(8:string[] ["APP_SEPARATOR", "Export JSON String to Clipboard"], 9:w797) -> ()  [unwired: 4 in, 3 out]
        n378 = event-data() -> ()  [unwired: 2 in, 1 out]
      }
      event "Phasor Ratio Color Map Type": Value Change {
        n379 = event-data() -> ("CtlRef"=w806:refnum<vi>, "NewVal"=w802:T46)  [unwired: 1 in]
        n380 = call "AlliGator Update Settings & Control.vi"("Value"=w802, "Sender"=w805, "CtlRef"=w806) -> ("Error Out"=w801:errorcluster)  [unwired: 8 in]
        n381 = Enqueue Element(queue=w803, element=T77 {"Action"=enum."Phasor Ratio Color Map Type Radio Button", "Data"=variant}, error in (no error)=w801) -> (error out=w799:errorcluster)  [unwired: 1 in, 2 out]
      }
      event "Phasor Ratio Color Map": Shortcut Menu Activation? {
        n382 = event-data() -> ("MenuRef"=w808:refnum<k9>)  [unwired: 1 in]
        n383 = flat-sequence {
          tunnel: w808 -> [w814]
          tunnel: [w810] -> w807
          frame #0 {
            w815 = AlliGator_Variables_List."Phasor Plot:Phasor Ratio Palette List" ("Alligator Variable")
            n384 = call "Alligator Variables Storage.vi"("Get(F)/Set"=FALSE, "AlliGator Variable"=AlliGator_Variables_List."Phasor Plot:Phasor Ratio Palette Information" ("Alligator Variable")) -> ("Error Out"=w825:errorcluster, "Data out"=w826:variant)  [unwired: 7 in, 1 out]
            n385 = call "Alligator Variables Storage.vi"("Get(F)/Set"=FALSE, "AlliGator Variable"=w815) -> ("Error Out"=w812:errorcluster, "Data out"=w819:variant)  [unwired: 7 in, 1 out]
            n386 = Variant To Data(error in=w825, type=T82 {"Palette Name [# Colors,int?,inv?]"="", "Palette Type"=0, "Palette Colors"=[], "Interpolate?"=FALSE} ("Image Display Palette Information"), Variant=w826) -> (data=w824:T82, error out=w823:errorcluster)
            n387 = call-poly "Variant to Data.vi"("Variant"=w819) -> ("String Array"=w818:string[])  [unwired: 8 in]
            n388 = Unbundle By Name(w824) -> ("Palette Name [# Colors,int?,inv?]"=w821:string)
            n389 = Merge Errors(w823, w812) -> (w813:errorcluster)
            n390 = call "Check Selected Palette in Menu.vi"("Error In"=w813, "Palette List"=w818, "Checked Palette"=w821, "Menu in"=w814) -> ("Error Out"=w811:errorcluster, "Stored Palette List"=w816:string[])  [unwired: 5 in, 1 out]
            n391 = call "Alligator Variables Storage.vi"("Get(F)/Set"=TRUE, "AlliGator Variable"=w815, "Error In"=w811, "Data in"=w816) -> ("Error Out"=w810:errorcluster)  [unwired: 5 in, 2 out]
          }
        }
        n392 = event-data() -> ()  [unwired: 2 in, 1 out]
      }
      event "Phasor Ratio Color Map": Shortcut Menu Selection (User) {
        n393 = event-data() -> ("CtlRef"=w829:refnum<vi>, "ItemTag"=w831:string)  [unwired: 1 in]
        n394 = case shown="\"\", Default" w831 {
          selector: w831 -> [w836 _]
          tunnel: w832 -> [w838 _]
          tunnel: [w834 w839] -> w830
          tunnel: w829 -> [_ w840]
          frame "", Default {
            n395 = Bundle By Name(cluster=T77 {"Action"=enum."Set Phasor Ratio Color Map", "Data"=variant} ("element"), "Data"=w836) -> (w835:T77)
            n396 = Enqueue Element(queue=w838, element=w835) -> (error out=w834:errorcluster)  [unwired: 2 in, 2 out]
          }
          frame "Export JSON String to Clipboard" {
            n397 = call "AlliGator Export Settings Parameter JSON String to Clipboard.vi"("Control Refnum"=w840) -> ("Error Out"=w839:errorcluster)  [unwired: 9 in, 1 out]
          }
        }
      }
      event "Phasor Ratio Color Scale": Shortcut Menu Activation? {
        w844 = string[] ["Copy Color Scale to Clipboard"] ("item names")
        n398 = event-data() -> ("MenuRef"=w843:refnum<k9>)  [unwired: 1 in]
        n399 = Delete Menu Items(9:w843) -> (0:w842:errorcluster, 3:w845:refnum<k9>)  [unwired: 3 in]
        n400 = Insert Menu Items(6:w842, 7:w844, 8:w844, 9:w845) -> (0:w841:errorcluster)  [unwired: 2 in, 2 out]
        n401 = event-data() -> ()  [unwired: 2 in, 1 out]
      }
      event "Phasor Ratio Color Scale": Shortcut Menu Selection (User) {
        n402 = event-data() -> ("CtlRef"=w848:refnum<vi>, "ItemTag"=w847:string)  [unwired: 1 in, 3 out]
        n403 = case shown="\"Copy Color Scale to Clipboard\"" w847 {
          tunnel: w848 -> [_ w850 w851]
          frame "", Default {
          }
          frame "Copy Color Scale to Clipboard" {
            n404 = call "Export Color Ramp to Clipboard.vi"("ColorRamp in"=w850) -> ()  [unwired: 11 in]
          }
          frame "Export JSON String to Clipboard" {
            n405 = call "AlliGator Export Settings Parameter JSON String to Clipboard.vi"("Control Refnum"=w851) -> ()  [unwired: 9 in, 2 out]
          }
        }
      }
      event Value Change {
        n406 = event-data() -> ("CtlRef"=w862:refnum<vi>, "NewVal"=w854:T47)  [unwired: 1 in]
        n407 = call "AlliGator Update Settings & Control.vi"("Value"=w854, "Sender"=w861, "CtlRef"=w862) -> ("Error Out"=w857:errorcluster)  [unwired: 8 in]
        n408 = Equal?(x=w854, y=AlliGator_Phasor_Ratio_Color-Coded_Quantity."User-Defined Quantity" ("NewVal")) -> (x = y?=w852:bool)
        n409 = property on="User-Defined Quantity" class="Str"("Visible"=w852) -> ()  [unwired: 2 in, 2 out]
        n410 = Bundle By Name(cluster=T77 {"Action"=enum."Phasor Ratio Color-Coded Quantity Changed", "Data"=variant} ("element"), "Data"=w854) -> (w855:T77)
        n411 = Enqueue Element(queue=w859, element=w855, error in (no error)=w857) -> (error out=w856:errorcluster)  [unwired: 1 in, 2 out]
      }
      event "Plugins Folder": Value Change {
        n412 = event-data() -> ()  [unwired: 1 in, 1 out]
        n413 = call "AlliGator Paths.vi"() -> ("Python Plugins Folder"=w863:path)  [unwired: 7 in, 4 out]
        n414 = Path To String(path=w863) -> (string=w864:string)
        n415 = Concatenate Strings("explorer.exe " ("command line"), w864) -> (w865:string)
        n416 = call <vilib>:"System Exec.vi"("command line"=w865) -> ()  [unwired: 7 in, 4 out]
      }
      event "Reset Python Session": Value Change {
        n417 = event-data() -> ("CtlRef"=w869:refnum<vi>)  [unwired: 1 in]
        n418 = property class="Bool"(reference=w869) -> ("Label.Text"=w868:string)  [unwired: 1 in, 2 out]
        n419 = call "AlliGator Reset Python Session.vi"() -> ("error out"=w873:errorcluster, "Valid Python Session"=w875:bool, "Message"=w874:string)  [unwired: 7 in, 2 out]
        n420 = call "Get Notebook Queue.vi"() -> ("Notebook Queue"=w872:refnum<queue>)  [unwired: 9 in]
        n421 = property on="Valid Python Session" class="Bool (strict)"("Value"=w875) -> ()  [unwired: 2 in, 2 out]
        n422 = call "Send Message to Notebook.vi"("Error In"=w873, "Text"=w874, "Notebook Queue"=w872) -> ("Error Out"=w871:errorcluster, "Notebook Queue"=w870:refnum<queue>)  [unwired: 5 in]
        n423 = call "Send Error to Notebook.vi"("error in (no error)"=w871, "State Machine Case Error Source"=w868, "Notebook Q"=w870) -> ()  [unwired: 8 in, 1 out]
      }
      event "Restore Skipped Dialogs": Value Change {
        w881 = AlliGator_Variables_List."Misc:Skippable Dialog Windows Status" ("Alligator Variable")
        n424 = event-data() -> ()  [unwired: 1 in, 1 out]
        n425 = call "Alligator Variables Storage.vi"("AlliGator Variable"=w881) -> ("Error Out"=w885:errorcluster, "Data out"=w886:variant)  [unwired: 8 in, 1 out]
        n426 = Variant To Data(error in=w885, type=T86[] [], Variant=w886) -> (data=w883:T86[], error out=w879:errorcluster)
        n427 = for {
          tunnel: w883 -> [w890] mode=indexing
          tunnel: [w889] -> w882 mode=indexing
          tunnel: FALSE ("NewVal") -> [w888]
          n428 = Bundle By Name(cluster=w890, "Is skipped"=w888) -> (w889:T86)
        }
        n429 = call "Alligator Variables Storage.vi"("Get(F)/Set"=TRUE, "AlliGator Variable"=w881, "Error In"=w879, "Data in"=w882) -> ("Error Out"=w877:errorcluster)  [unwired: 5 in, 2 out]
      }
      event "Send JSON to Clipboard": Value Change {
        n430 = event-data() -> ()  [unwired: 1 in, 1 out]
        n431 = Enqueue Element(queue=w891, element=T77 {"Action"=enum."Send Parameters JSON Strings to Clipboard", "Data"=variant}) -> ()  [unwired: 2 in, 3 out]
      }
      event "Settings Tabs", "Fluorescence Decay Tabs": Shortcut Menu Selection (User) {
        n432 = event-data() -> ("CtlRef"=w895:refnum<vi>, "ItemTag"=w897:string)  [unwired: 1 in]
        n433 = case shown="\"Reset Parameters to Default (this panel only)\"" w897 {
          tunnel: w896 -> [_ _ _]
          tunnel: w895 -> [_ w909 _]
          tunnel: [_ w899 _] -> w894
          frame "", Default {
          }
          frame "Reset Parameters to Default (this panel only)" {
            n434 = property class="TabCtl"(reference=w909) -> (error out=w906:errorcluster, "Pages"=w905:refnum<vi>[], "Value"=w908:variant)  [unwired: 1 in, 1 out]
            n435 = Variant To Data(type=u32 0 ("index"), Variant=w908) -> (data=w903:u32)  [unwired: 1 in, 1 out]
            n436 = Index Array(array=w905, index=w903) -> (element=w907:refnum<vi>)
            n437 = property class="Page"(reference=w907, error in=w906) -> (error out=w904:errorcluster, "PageLabel"=w901:string)  [unwired: 1 out]
            n438 = Close Reference(reference=w905, error in (no error)=w904) -> ()  [unwired: 1 out]
            n439 = call "AlliGator Init Settings v2.vi"("Settings Panel (Empty: All)"=w901) -> ("error out"=w900:errorcluster)  [unwired: 10 in]
            n440 = case shown="\"Decay Pre-Processing\"" w901 {
              tunnel: w900 -> [w910 w912]
              tunnel: [w910 w911] -> w899
              frame "", Default {
              }
              frame "Decay Pre-Processing" {
                # "Special item to handle"
                n441 = call "AlliGator Settings Storage.vi"("AlliGator Settings List"=AlliGator_Settings_List."Fluorescence Decay_Decay Pre-Processing:Decay Pre-Processing Operations Order", "Error In"=w912) -> ("Error Out"=w914:errorcluster, "Variant Data out"=w916:variant)  [unwired: 8 in]
                n442 = call-poly "Variant to Data.vi"("Variant"=w916) -> ("String Array"=w915:string[])  [unwired: 8 in]
                n443 = property on="Decay Pre-Processing Operations Order" class="Ring (strict)"(error in=w914, "Strings []"=w915) -> (error out=w911:errorcluster)  [unwired: 1 in, 1 out]
              }
            }
          }
          frame "Reset All Parameters to Default" {
            n444 = call "AlliGator Init Settings v2.vi"() -> ("error out"=w917:errorcluster)  [unwired: 11 in]
            n445 = call "AlliGator Settings Storage.vi"("AlliGator Settings List"=AlliGator_Settings_List."Fluorescence Decay_Decay Pre-Processing:Decay Pre-Processing Operations Order", "Error In"=w917) -> ("Error Out"=w919:errorcluster, "Variant Data out"=w921:variant)  [unwired: 8 in]
            n446 = call-poly "Variant to Data.vi"("Variant"=w921) -> ("String Array"=w920:string[])  [unwired: 8 in]
            n447 = property on="Decay Pre-Processing Operations Order" class="Ring (strict)"(error in=w919, "Strings []"=w920) -> ()  [unwired: 1 in, 2 out]
          }
        }
      }
      event "Settings Tabs": Value Change {
        n448 = event-data() -> ("NewVal"=w928:T1)  [unwired: 1 in]
        n449 = Format Into String(w928) -> (resulting string=w926:string)  [unwired: 3 in, 1 out]
        n450 = call "AlliGator Settings Storage.vi"("Get(F)/Set"=TRUE, "AlliGator Settings List"=AlliGator_Settings_List."GUI:Visible Settings Tab", "Variant Data in"=w926) -> ("Error Out"=w924:errorcluster)  [unwired: 7 in, 1 out]
        n451 = call "AlliGator Settings Event Refnum.vi"("Error In"=w924) -> ("Error Out"=w922:errorcluster)  [unwired: 7 in, 1 out]
      }
      event "Shift Decay": Value Change {
        n452 = event-data() -> ("CtlRef"=w936:refnum<vi>, "NewVal"=w932:bool)  [unwired: 1 in]
        n453 = call "AlliGator Update Settings & Control.vi"("Value"=w932, "Sender"=w935, "CtlRef"=w936) -> ("Error Out"=w931:errorcluster)  [unwired: 8 in]
        n454 = Enqueue Element(queue=w933, element=T77 {"Action"=enum."Shift Decay Checkbox", "Data"=variant}, error in (no error)=w931) -> (error out=w929:errorcluster)  [unwired: 1 in, 2 out]
      }
      event "Smoothen Decay": Value Change {
        n455 = event-data() -> ("CtlRef"=w944:refnum<vi>, "NewVal"=w940:bool)  [unwired: 1 in]
        n456 = call "AlliGator Update Settings & Control.vi"("Value"=w940, "Sender"=w943, "CtlRef"=w944) -> ("Error Out"=w938:errorcluster)  [unwired: 8 in]
        n457 = Enqueue Element(queue=w941, element=T77 {"Action"=enum."Smooth Decay Checkbox", "Data"=variant}, error in (no error)=w938) -> (error out=w937:errorcluster)  [unwired: 1 in, 2 out]
      }
      event "Source Image Tabs": Value Change {
        n458 = event-data() -> ("NewVal"=w945:T2)  [unwired: 1 in]
        n459 = case shown="\"Image Processing\"" w945 {
          frame "Pixel Processing", Default {
          }
          frame "Image Processing" {
            n460 = call "AlliGator Settings Storage.vi"("AlliGator Settings List"=AlliGator_Settings_List."Source Image:Image Pre-Processing Operations Order") -> ("Error Out"=w947:errorcluster, "Variant Data out"=w949:variant)  [unwired: 9 in]
            n461 = call-poly "Variant to Data.vi"("Variant"=w949) -> ("String Array"=w948:string[])  [unwired: 8 in]
            n462 = property on="Image Pre-Processing Operations Order" class="Ring (strict)"(error in=w947, "Strings []"=w948) -> ()  [unwired: 1 in, 2 out]
          }
        }
      }
      event "SYNC Period": Shortcut Menu Selection (User) {
        n463 = event-data() -> ("CtlRef"=w951:refnum<vi>, "ItemTag"=w952:string)  [unwired: 1 in]
        n464 = case shown="\"Export JSON String to Clipboard\"" w952 {
          tunnel: w951 -> [_ w954 w956]
          frame "", Default {
          }
          frame "Same as Laser Period" {
            n465 = property on="Laser Period" class="DigNum (strict)"() -> ("Value"=w955:dbl[unit])  [unwired: 2 in, 2 out]
            n466 = property class="DigNum (strict)"(reference=w954, "Val(Sgnl)"=w955) -> ()  [unwired: 1 in, 2 out]
          }
          frame "Export JSON String to Clipboard" {
            n467 = call "AlliGator Export Settings Parameter JSON String to Clipboard.vi"("Control Refnum"=w956) -> ()  [unwired: 9 in, 2 out]
          }
        }
      }
      event "Use Current Dataset Parameters": Value Change {
        n468 = event-data() -> ()  [unwired: 1 in, 1 out]
        n469 = Enqueue Element(queue=w958, element=T77 {"Action"=enum."Set SEPL Parameters to Dataset Ones", "Data"=variant}) -> ()  [unwired: 2 in, 3 out]
      }
      event "Use Cursors": Value Change {
        n470 = event-data() -> ("CtlRef"=w968:refnum<vi>, "NewVal"=w960:bool)  [unwired: 1 in]
        n471 = call "AlliGator Update Settings & Control.vi"("Value"=w960, "Sender"=w967, "CtlRef"=w968) -> ("Error Out"=w964:errorcluster)  [unwired: 8 in]
        n472 = Bundle By Name(cluster=T77 {"Action"=enum."Use Cursor (Extrapolate) Checkbox", "Data"=variant} ("element"), "Data"=w960) -> (w961:T77)
        n473 = Enqueue Element(queue=w965, element=w961, error in (no error)=w964) -> (error out=w962:errorcluster)  [unwired: 1 in, 2 out]
      }
      event "Use File Timestamp": Value Change {
        n474 = event-data() -> ("CtlRef"=w976:refnum<vi>, "NewVal"=w972:bool)  [unwired: 1 in]
        n475 = call "AlliGator Update Settings & Control.vi"("Value"=w972, "Sender"=w975, "CtlRef"=w976) -> ("Error Out"=w971:errorcluster)  [unwired: 8 in]
        n476 = Enqueue Element(queue=w973, element=T77 {"Action"=enum."Use File Timestamp Checkbox", "Data"=variant}, error in (no error)=w971) -> (error out=w969:errorcluster)  [unwired: 1 in, 2 out]
      }
      event "Use Fixed ROI Diameter": Value Change {
        n477 = event-data() -> ("CtlRef"=w984:refnum<vi>, "NewVal"=w982:bool)  [unwired: 1 in]
        n478 = call "AlliGator Update Settings & Control.vi"("Value"=w982, "Sender"=w983, "CtlRef"=w984) -> ("Error Out"=w978:errorcluster)  [unwired: 8 in]
        n479 = Enqueue Element(queue=w980, element=T77 {"Action"=enum."Use Fixed ROI Diameter Checkbox", "Data"=variant}, error in (no error)=w978) -> (error out=w977:errorcluster)  [unwired: 1 in, 2 out]
      }
      event "Use Periodicity": Value Change {
        n480 = event-data() -> ("CtlRef"=w993:refnum<vi>, "NewVal"=w985:bool)  [unwired: 1 in]
        n481 = call "AlliGator Update Settings & Control.vi"("Value"=w985, "Sender"=w992, "CtlRef"=w993) -> ("Error Out"=w989:errorcluster)  [unwired: 8 in]
        n482 = Bundle By Name(cluster=T77 {"Action"=enum."Use Periodicity (Extrapolate) Checkbox", "Data"=variant} ("element"), "Data"=w985) -> (w986:T77)
        n483 = Enqueue Element(queue=w990, element=w986, error in (no error)=w989) -> (error out=w987:errorcluster)  [unwired: 1 in, 2 out]
      }
      event "User-Defined Quantity": Shortcut Menu Selection (User) {
        n484 = event-data() -> ("ItemTag"=w994:string)  [unwired: 1 in]
        n485 = case shown="\"User-defined Quantity List\"" w994 {
          frame "", Default {
          }
          frame "User-defined Quantity List" {
            n486 = vi-ref "Formula.lvlib:Aliases Definition Window.vi"() -> (w1004:refnum<vi>)
            n487 = property class="VI"(reference=w1004) -> (reference out=w1003:refnum<vi>, error out=w999:errorcluster, "Path"=w997:path)  [unwired: 1 in]
            n488 = call "Get-Set Reserved Keywords.vi"("Get (F)/Set"=TRUE, "Error In"=w999, "Formula Interpreter Path"=w997, "Reserved Keywords"=T87 ["f_1", "a_1", "<tau>_a", "<tau>_i", "tau_1", "tau_2"] ("Basic Burst Statistics Names")) -> ("Error Out"=w998:errorcluster, "Formula Interpreter Path"=w996:path)  [unwired: 5 in, 1 out]
            n489 = call "Run Vi.vi"("VI Path"=w996, "error in (no error)"=w998) -> ("error out"=w1002:errorcluster)  [unwired: 6 in, 1 out]
            n490 = Close Reference(reference=w1003, error in (no error)=w1002) -> ()  [unwired: 1 out]
          }
        }
      }
      event User Event {
        n491 = event-data() -> ("AlliGator Settings Message"=w1015:T89, "Control Label"=w1014:string, "Data"=w1013:variant, "Sender"=w1011:string)  [unwired: 1 in]
        n492 = case shown="\"Refresh Parameter\"" w1015 {
          tunnel: w1014 -> [_ _ w1023 _]
          tunnel: w1013 -> [_ _ w1024 _]
          tunnel: w1012 -> [_ _ w1025 _]
          tunnel: w1011 -> [_ _ w1022 _]
          tunnel: w1010 -> [_ _ w1021 _]
          tunnel: [_ TRUE ("Discard?") _ _] -> w1009
          tunnel: w1007 -> [_ w1018 _ w1057]
          tunnel: w1006 -> [_ w1016 _ _]
          frame "Idle", Default {
          }
          frame "Quit" {
            n493 = Unregister For Events(event registration refnum=w1016) -> ()  [unwired: 1 in, 1 out]
            n494 = Enqueue Element(queue=w1018, element=T77 {"Action"=enum."Quit", "Data"=variant}) -> ()  [unwired: 2 in, 3 out]
          }
          frame "Refresh Parameter" {
            n495 = Equal?(x=w1022, y=w1021) -> (x = y?=w1020:bool)
            n496 = case shown="False" w1020 {
              tunnel: w1025 -> [w1033 _]
              tunnel: w1024 -> [w1031 _]
              tunnel: w1023 -> [w1032 _]
              frame False {
                n497 = call "AlliGator Settings Storage.vi"("AlliGator Settings List"=AlliGator_Settings_List."Miscellaneous:Verbose Settings Mode") -> ("Error Out"=w1028:errorcluster, "Variant Data out"=w1030:variant)  [unwired: 9 in]
                n498 = call-poly "Variant to Data.vi"("Variant"=w1030) -> ("Value"=w1029:bool)  [unwired: 8 in]
                n499 = call "AlliGator Refresh Single Setting.vi"("Verbose (T)"=w1029, "Error In"=w1028, "Data"=w1031, "Control Label"=w1032, "VI Ref in"=w1033) -> ("Error Out"=w1035:errorcluster, "VI Ref (dup)"=w1026:refnum<vi>)  [unwired: 5 in]
                n500 = case shown="\"Phasor Graph Frequency\"" w1032 {
                  tunnel: w1031 -> [_ w1040 w1045 w1052]
                  tunnel: w1035 -> [w1036 w1039 w1044 w1051]
                  tunnel: [w1036 w1038 w1043 w1050] -> w1034
                  tunnel: w1026 -> [_ w1037 w1042 w1048]
                  frame "False", Default {
                  }
                  frame "Phasor Graph Frequency" {
                    n501 = call "AlliGator Refresh Single Setting.vi"("Error In"=w1039, "Data"=w1040, "Control Label"="Phasor Plot Frequency", "VI Ref in"=w1037) -> ("Error Out"=w1038:errorcluster)  [unwired: 6 in, 1 out]
                  }
                  frame "Phasor Plot Frequency" {
                    n502 = call "AlliGator Refresh Single Setting.vi"("Error In"=w1044, "Data"=w1045, "Control Label"="Phasor Graph Frequency", "VI Ref in"=w1042) -> ("Error Out"=w1043:errorcluster)  [unwired: 6 in, 1 out]
                  }
                  frame "Phasor Frequency" {
                    n503 = call "Tiny Clear Error.vi"("Error In"=w1051) -> ("no Error Out"=w1047:errorcluster)  [unwired: 8 in]
                    n504 = call "AlliGator Refresh Single Setting.vi"("Error In"=w1047, "Data"=w1052, "Control Label"="Phasor Graph Frequency", "VI Ref in"=w1048) -> ("Error Out"=w1054:errorcluster)  [unwired: 6 in, 1 out]
                    n505 = call "AlliGator Refresh Single Setting.vi"("Error In"=w1047, "Data"=w1052, "Control Label"="Phasor Plot Frequency", "VI Ref in"=w1048) -> ("Error Out"=w1049:errorcluster)  [unwired: 6 in, 1 out]
                    n506 = Merge Errors(w1054, w1049) -> (w1050:errorcluster)
                  }
                }
                n507 = call "Tiny Clear Error.vi"("Error In"=w1034) -> ()  [unwired: 8 in, 1 out]
              }
              frame True {
              }
            }
          }
          frame "Refresh All Parameters" {
            n508 = Enqueue Element(queue=w1057, element=T77 {"Action"=enum."Refresh All Parameters", "Data"=variant}) -> ()  [unwired: 2 in, 3 out]
          }
        }
      }
      event Mouse Down {
        w1058 = TRUE  # Tracking
        n509 = event-data() -> ("CtlRef"=w1060:refnum<vi>)  [unwired: 1 in]
        n510 = register-events(reference=w1062, refnum<vi> refnum ("Guess Parameters"), w1060, w1060) -> (reference out=w1061:refnum<event-registration>)  [unwired: 2 in, 1 out]
      }
      event Mouse Move {
        n511 = event-data() -> ("CtlRef"=w1067:refnum<vi>)  [unwired: 1 in]
        n512 = control-ref of="Guess Parameter Names"() -> (w1066:refnum<vi>)
        n513 = property class="Arr (strict)"(reference=w1067) -> (error out=w1065:errorcluster, "Index Values"=w1064:u32[])  [unwired: 1 in, 1 out]
        n514 = property class="Arr (strict)"(reference=w1066, error in=w1065, "Index Values"=w1064) -> (error out=w1063:errorcluster)  [unwired: 1 out]
      }
      event Mouse Up {
        w1071 = FALSE  # Tracking
        w1070 = refnum<vi> refnum ("Guess Parameters")
        n515 = event-data() -> ("CtlRef"=w1069:refnum<vi>)  [unwired: 1 in]
        n516 = register-events(reference=w1073, w1069, w1070, w1070) -> (reference out=w1072:refnum<event-registration>)  [unwired: 2 in, 1 out]
      }
      event Panel Close? {
        w1074 = TRUE ("Discard?")
        n517 = event-data() -> ()  [unwired: 1 in, 1 out]
        n518 = Unregister For Events(event registration refnum=w1078) -> ()  [unwired: 1 in, 1 out]
        n519 = Enqueue Element(queue=w1076, element=T77 {"Action"=enum."Quit", "Data"=variant}) -> ()  [unwired: 2 in, 3 out]
        n520 = event-data("Discard?"=w1074) -> ()  [unwired: 1 in, 1 out]
      }
      event Timeout {
        n521 = event-data() -> ()  [unwired: 1 in, 3 out]
        n522 = Enqueue Element(queue=w1079, element=T77 {"Action"=enum."Store Phasor Ratio Color Scale Hi/Lo Colors", "Data"=variant}) -> ()  [unwired: 2 in, 3 out]
      }
    }
    n523 = call "AlliGator Check whether Source Image needs update.vi"("Error In"=w351) -> ()  [unwired: 10 in, 1 out]
    n524 = call "AlliGator Check whether Phasor Plot needs update.vi"("Error In"=w351) -> ()  [unwired: 10 in, 1 out]
  }
  n525 = CPU Information() -> (4:w6:i32)  [unwired: 3 out]
  "# Logical Processors" <- w6
  n526 = property on="# Logical Processors Used" class="Digital (strict)"("Maximum"=w6, "Minimum"=w10, "OutOfRngActMin"=w10, "OutOfRngActMax"=w6) -> ()  [unwired: 2 in, 2 out]
  n527 = invoke class="VI" method="FP.Close"(reference=w12) -> (reference out=w24:refnum<vi>, error out=w23:errorcluster)  [unwired: 2 in, 1 out]
  n528 = Close Reference(reference=w24, error in (no error)=w23) -> ()  [unwired: 1 out]
